vi "HandleObservationSync.vi"(8 "error in (no error)":errorcluster, 11 "S4ACS_GUI in":refnum<class "S4GUI.lvclass">) -> (0 "error out":errorcluster, 3 "S4ACS_GUI out":refnum<class "S4GUI.lvclass">)   [LabVIEW 2018, in "S4GUI.lvclass"]
uses:
  S4GUI.lvclass
  S4GUI.lvclass/S4GUI.ctl
  Instrument/Instrument.lvclass/Instrument.ctl
  Device/Optics/Optics.lvclass/Optics.ctl
  Server/Server.lvclass/Server.ctl
  Interface/Interface.lvclass/Interface.ctl
  Device/Optics/Opt_Selector/Opt_Selector.lvclass
  C:/Users/observer/Desktop/Sparc4GUI/SPARC4_GUI/Device/Optics/Optics.lvclass
  Acquisition/Acquisition.lvclass
  C:/Users/observer/Desktop/Sparc4GUI/SPARC4_GUI/Server/Server.lvclass
  SyncBox/Sync Box.lvclass
  Instrument/Instrument.lvclass
  Device/Optics/Opt_Continuous/Opt_Continuous.lvclass
  StateMachine/State Machine.lvclass
  Trigger/Trigger.lvclass
  Channel/Channel.lvclass
  Interface/Interface.lvclass
  Device/Optics/Optics.lvclass
  Server/Server.lvclass
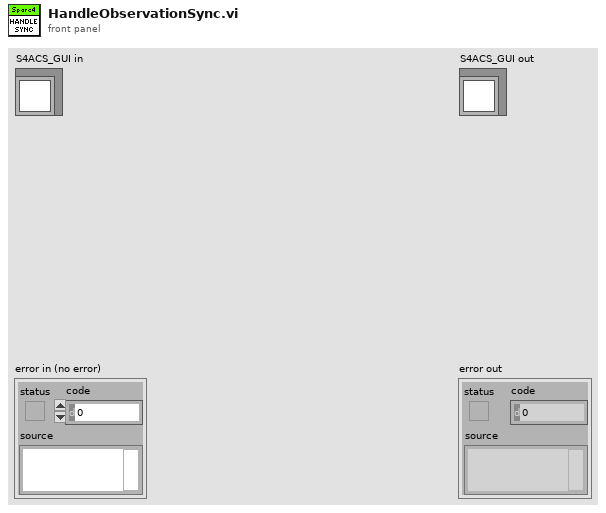
[diagram p1: front panel]
types:
  T1 = cluster{"ACQUISITION_MODE":u8, "TRIGGER_MODE":u8, "READ_MODE":u8, "PREAMP":u8, "READOUT_RATE":u8, "VERTICAL_SHIFT_SPEED":u8, "EM_MODE":u8, "EM_GAIN":u16, "SHUTTER_MODE":u8, "SHUTTER_TTL":u8, "SHUTTER_OPENING_TIME":u16, "SHUTTER_CLOSING_TIME":u16, "VBIN":u16, "HBIN":u16, "INITIAL_LINE":u16, "INITIAL_COLUMN":u16, "FINAL_LINE":u16, "FINAL_COLUMN":u16, "FRAME_TRANSFER":bool, "VERTICAL_CLOCK_VOLTAGE":u8, "AD_CHANNEL":u32}
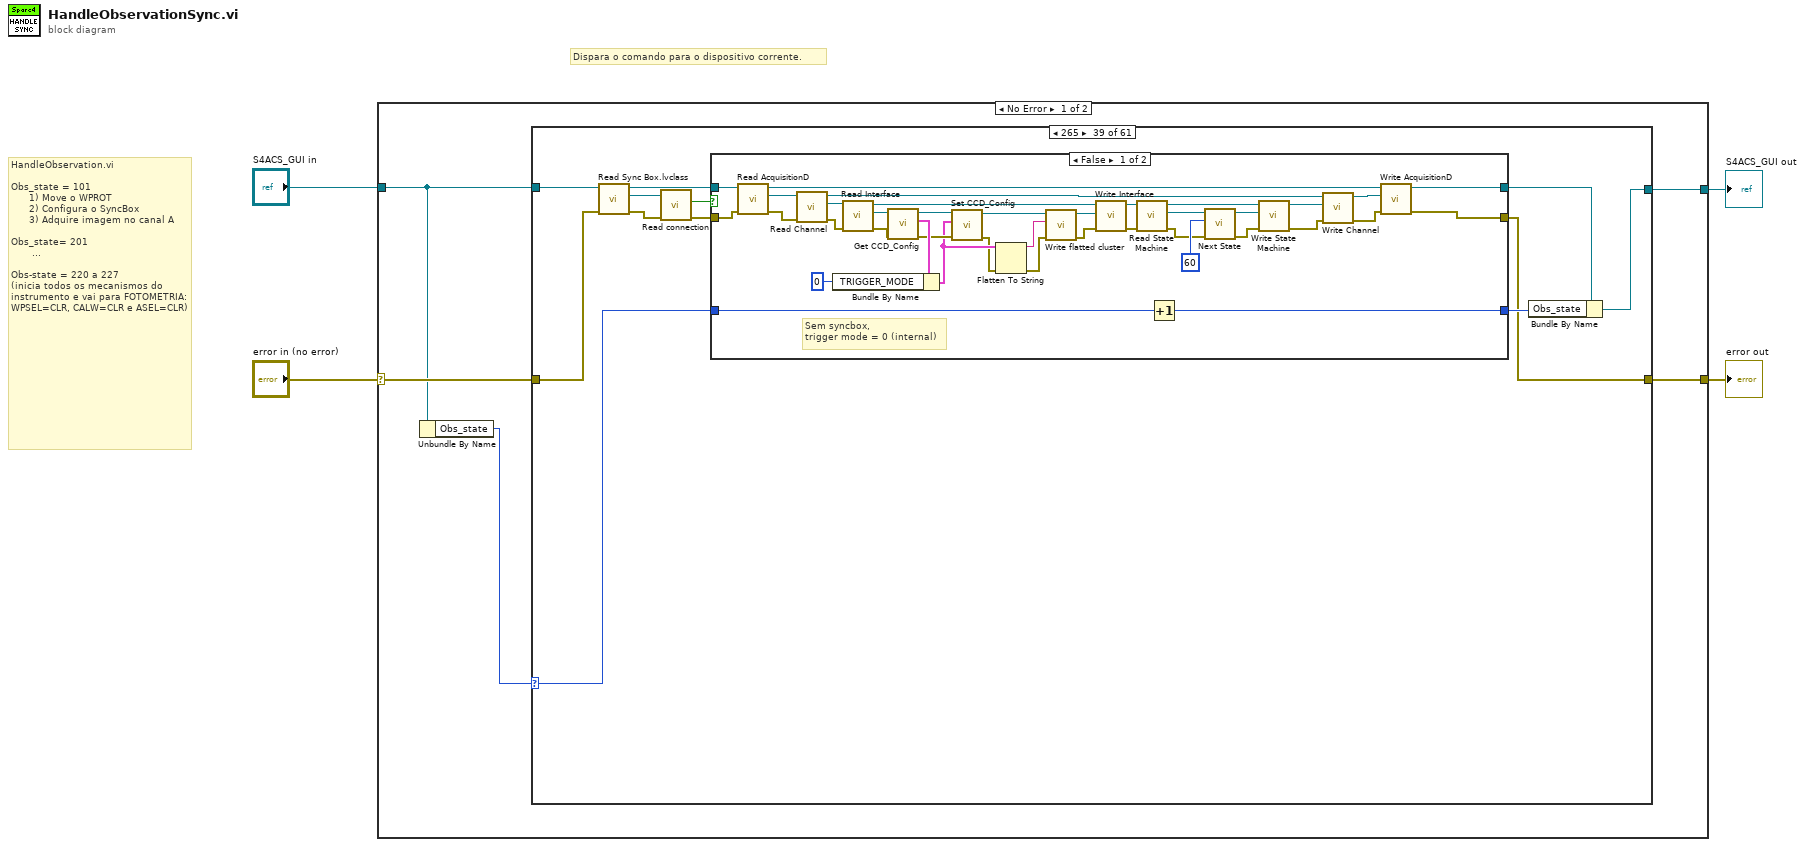
[diagram p0: block diagram]
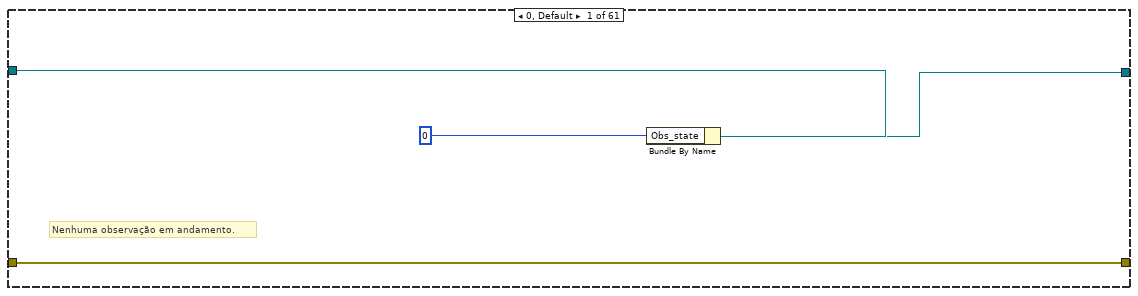
[diagram p2: hidden frame]
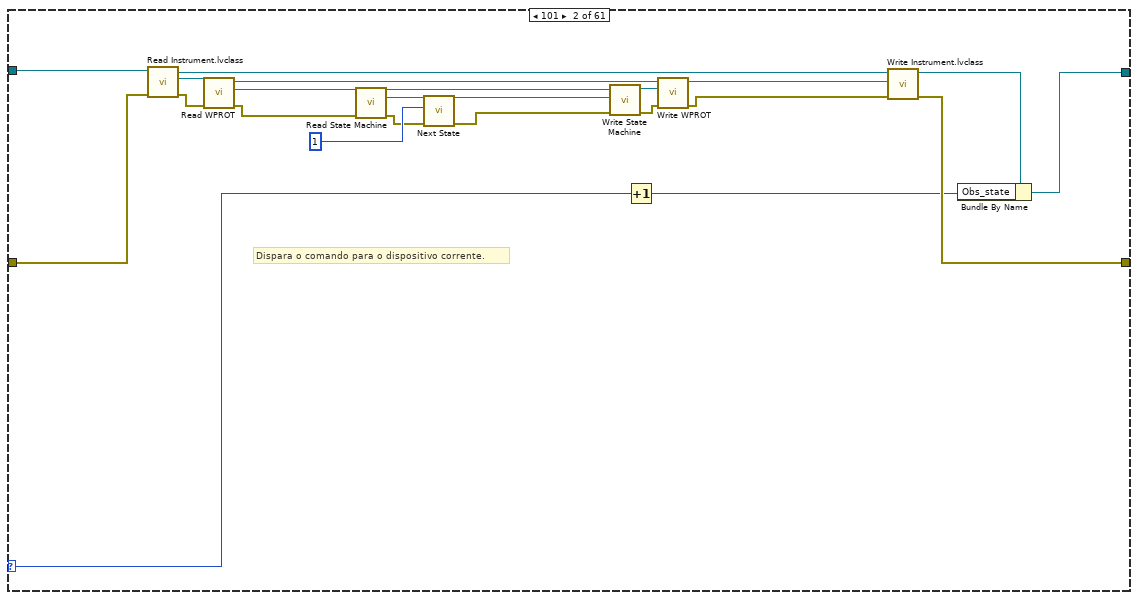
[diagram p3: hidden frame]
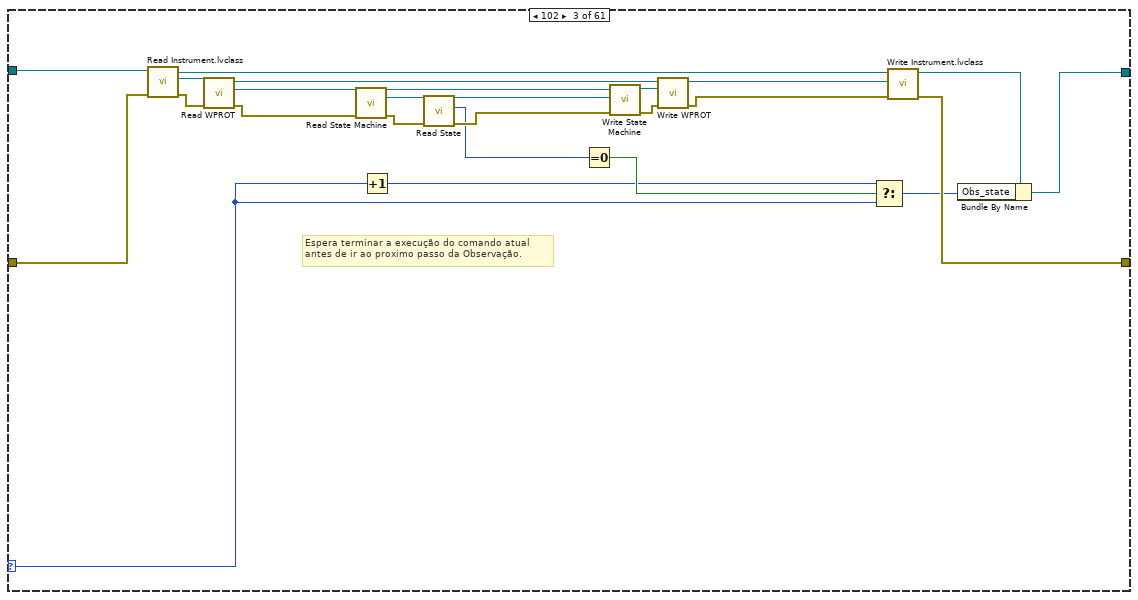
[diagram p4: hidden frame]
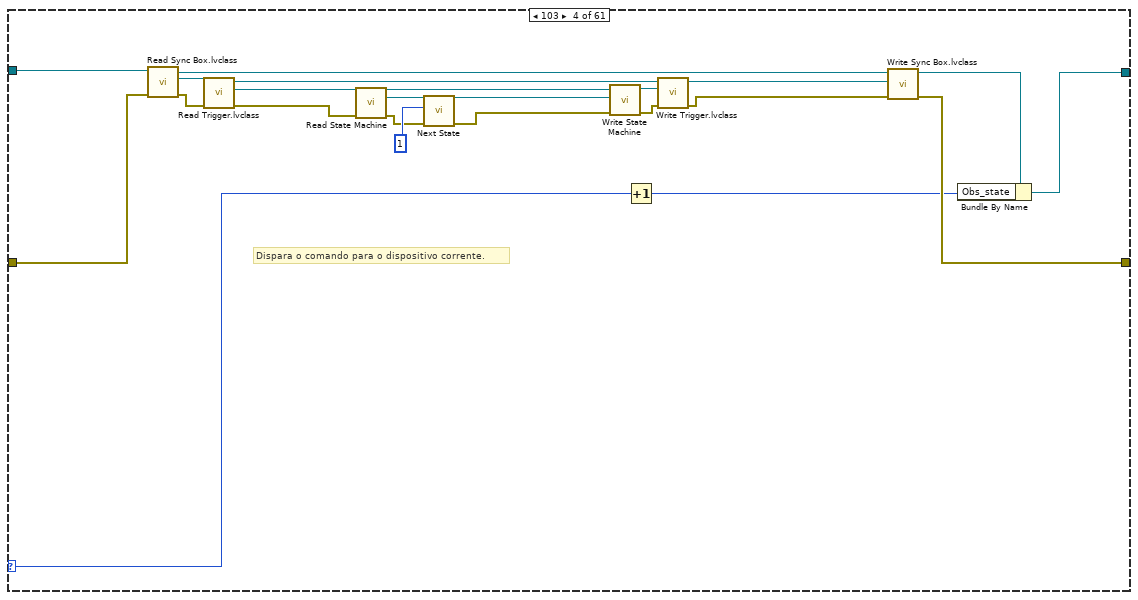
[diagram p5: hidden frame]
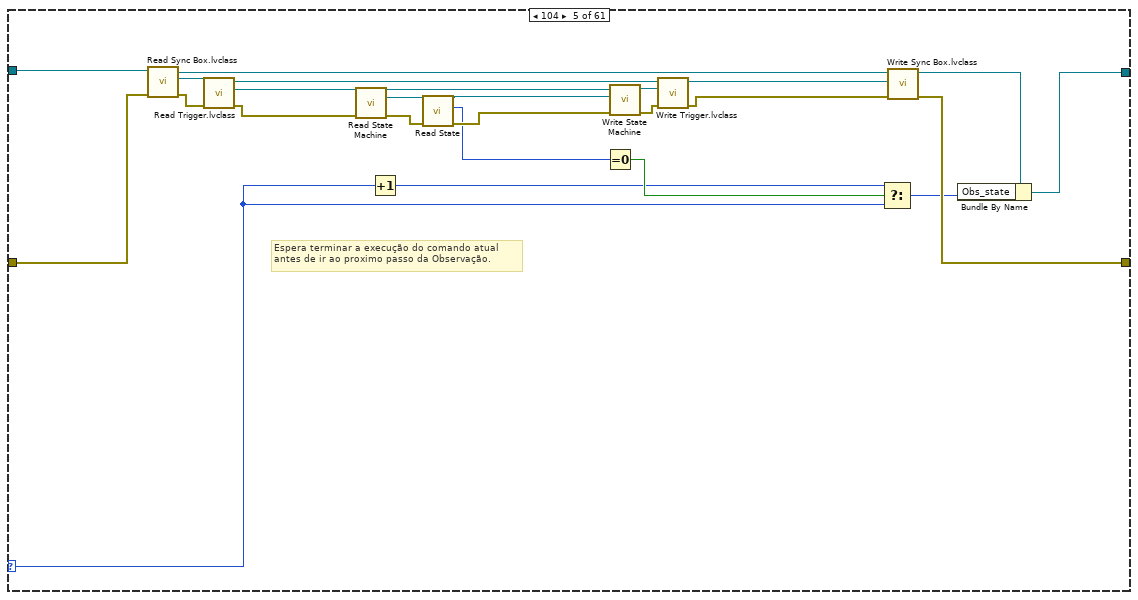
[diagram p6: hidden frame]
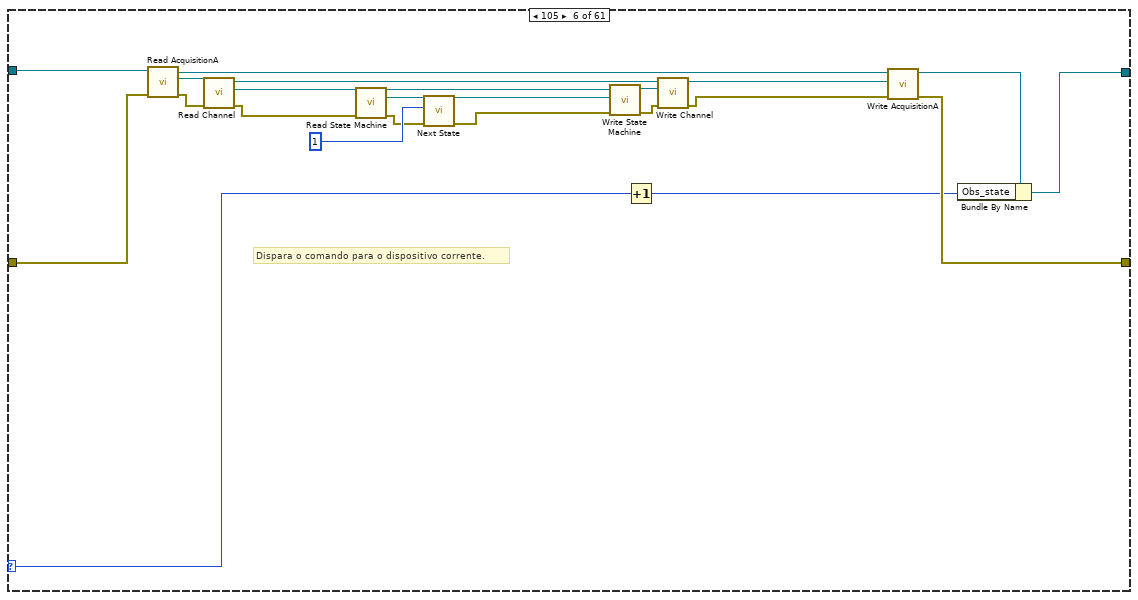
[diagram p7: hidden frame]
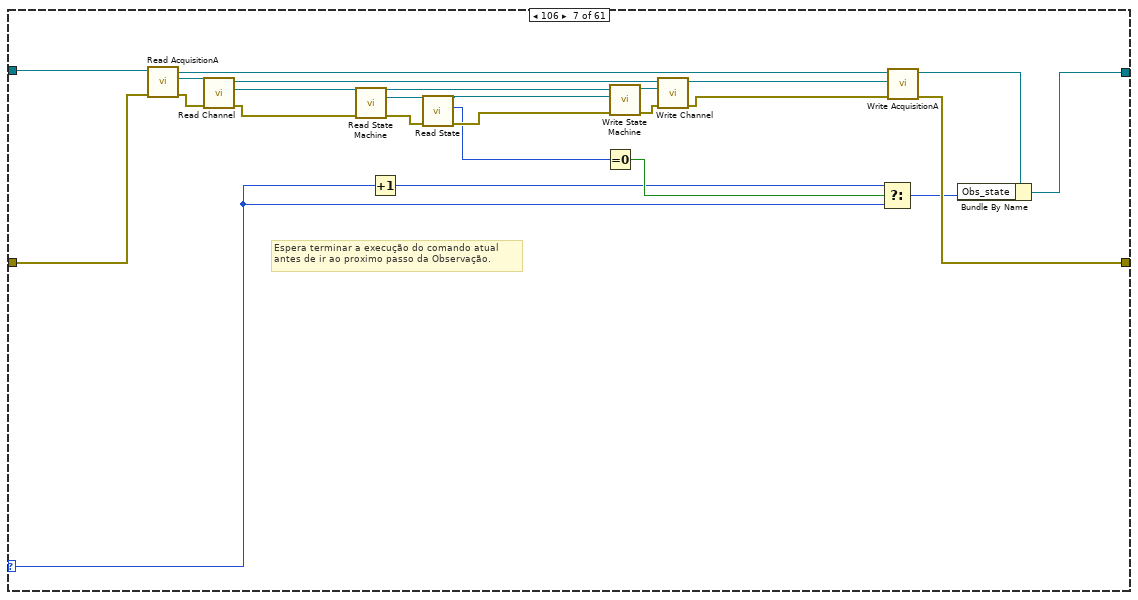
[diagram p8: hidden frame]
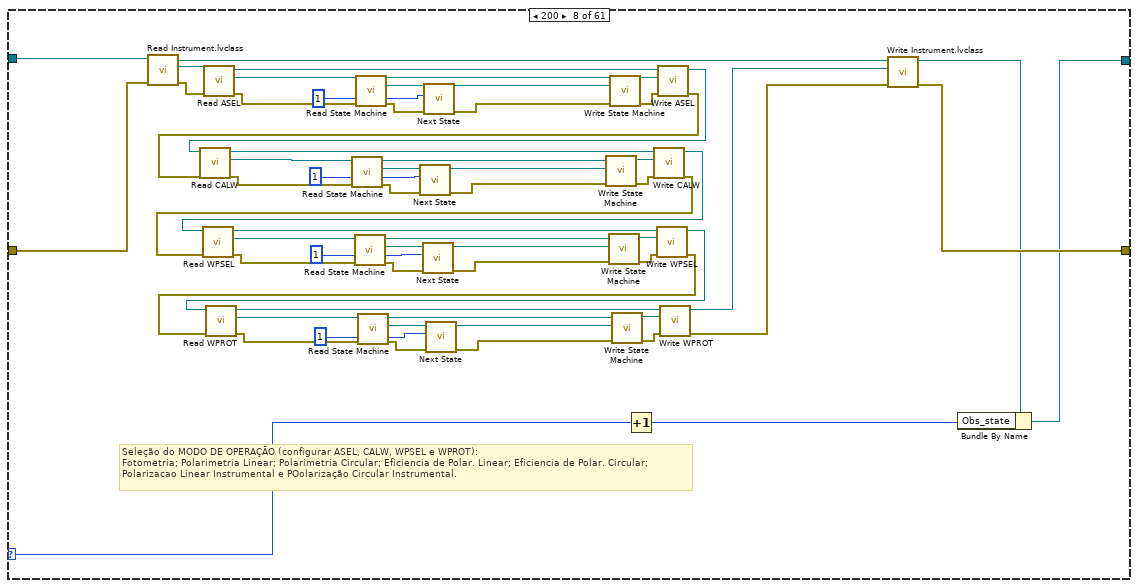
[diagram p9: hidden frame]
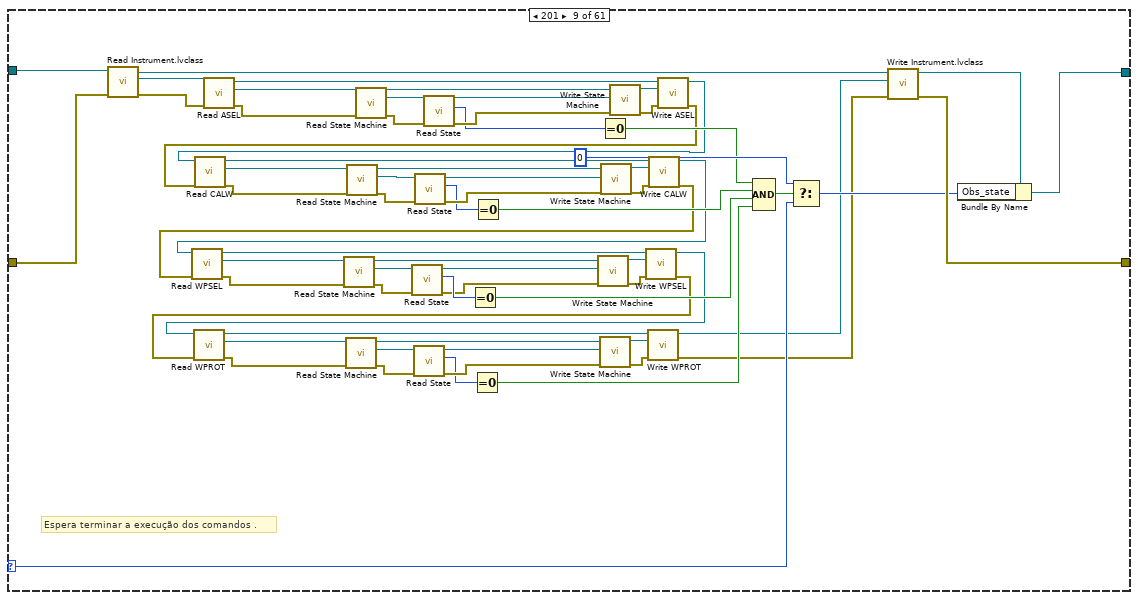
[diagram p10: hidden frame]
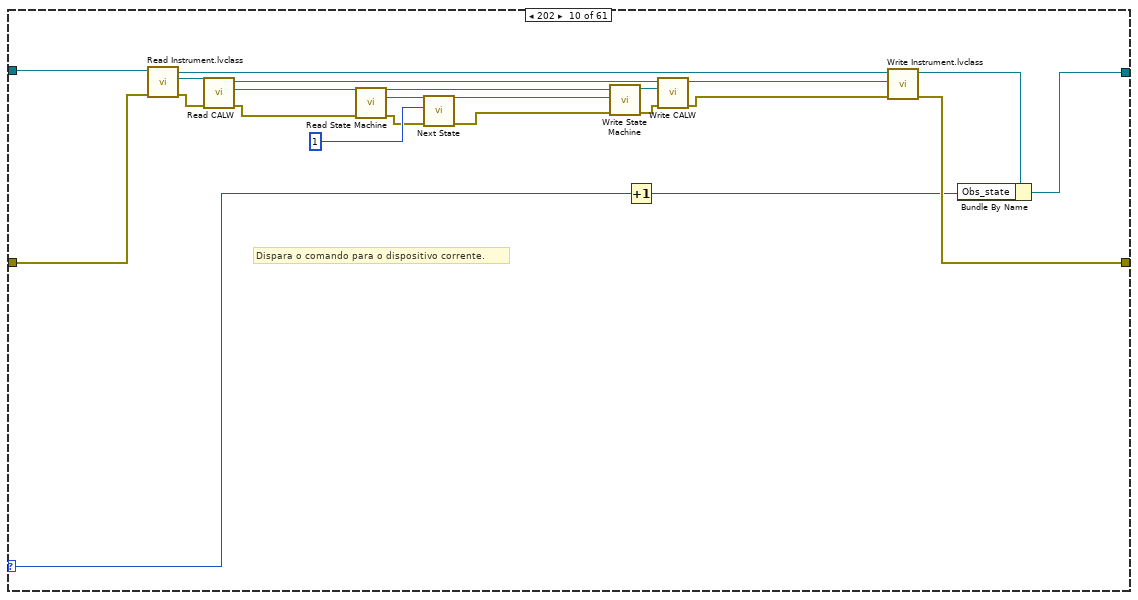
[diagram p11: hidden frame]
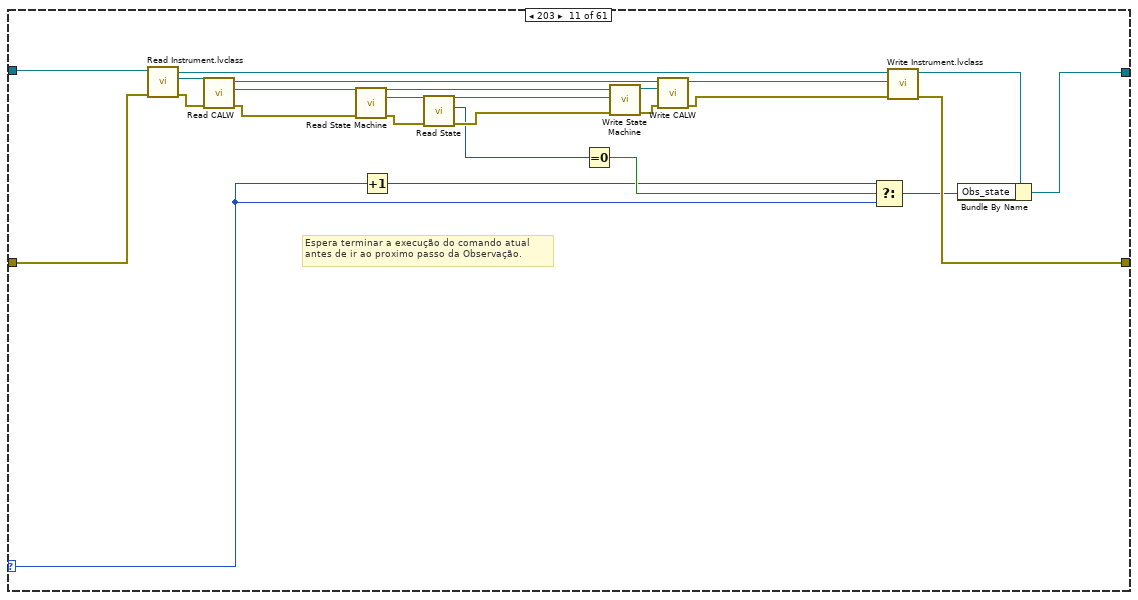
[diagram p12: hidden frame]
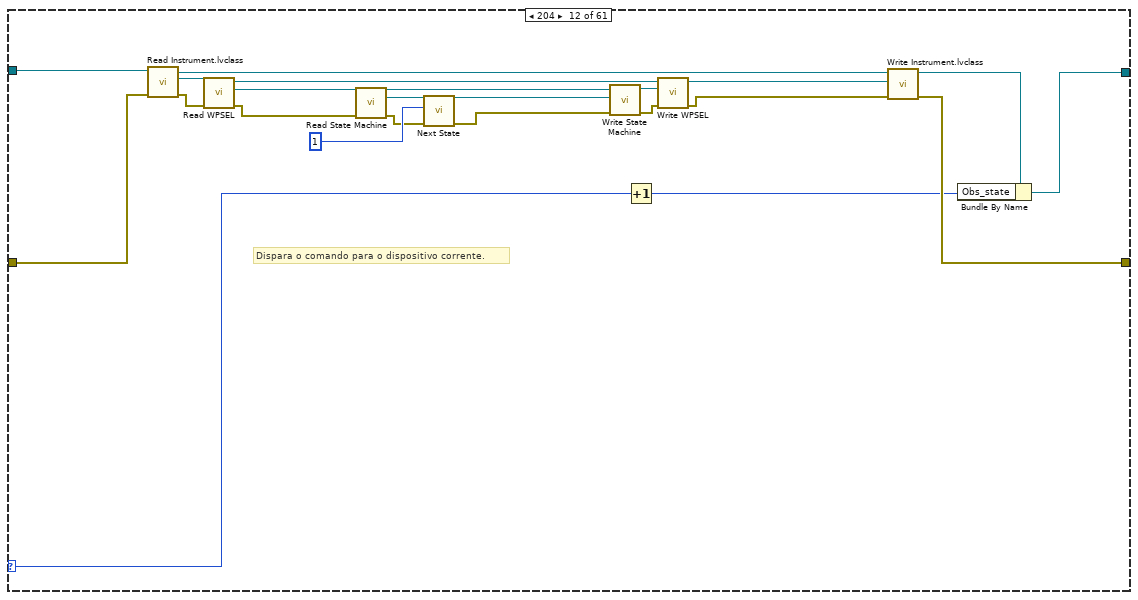
[diagram p13: hidden frame]
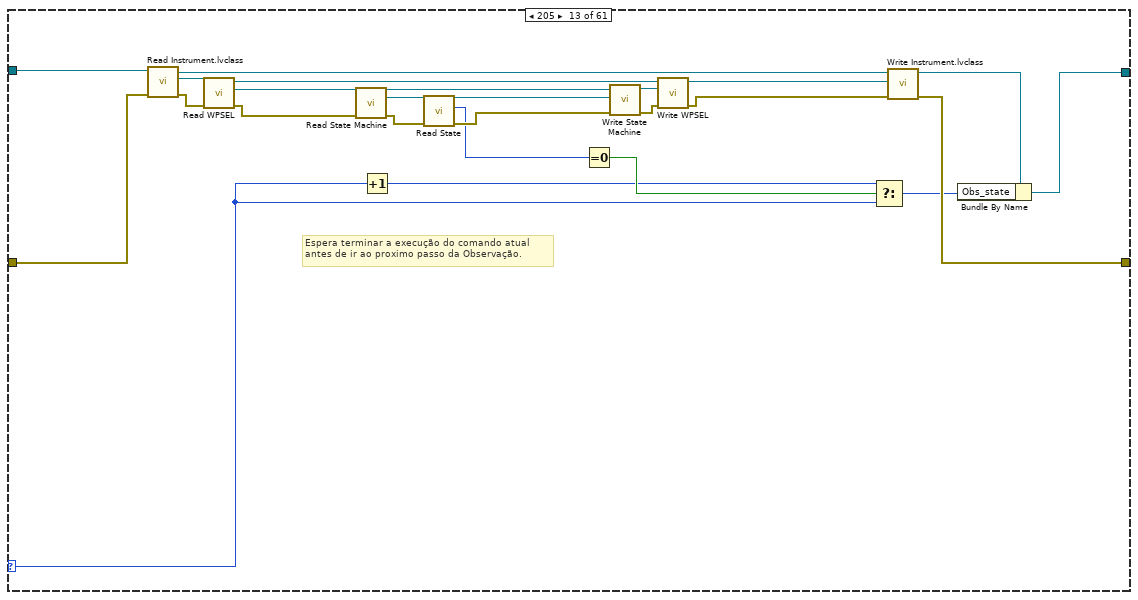
[diagram p14: hidden frame]
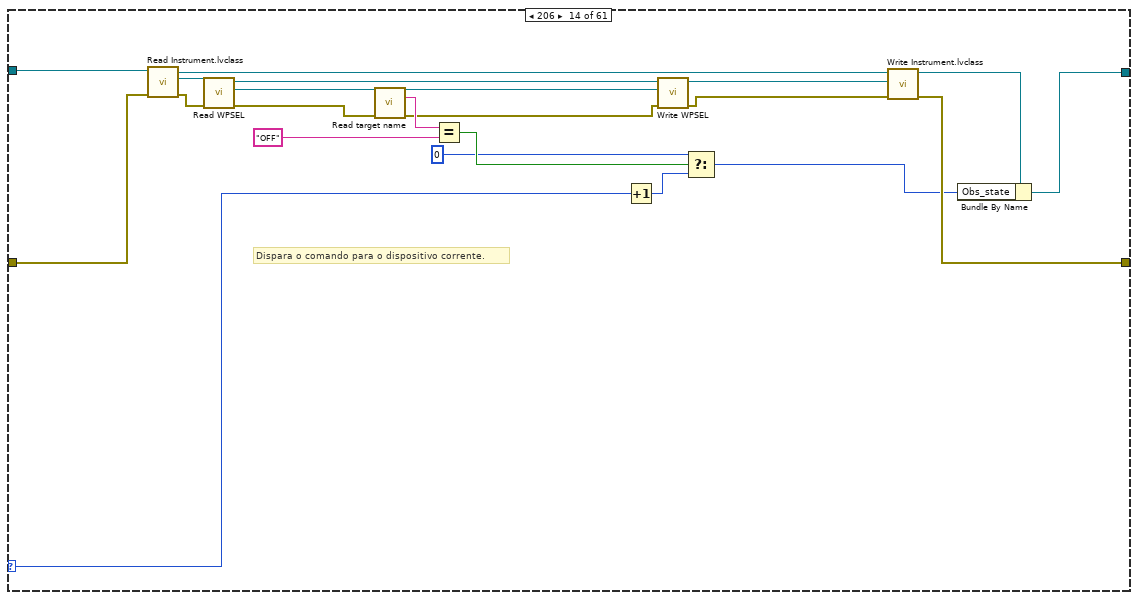
[diagram p15: hidden frame]
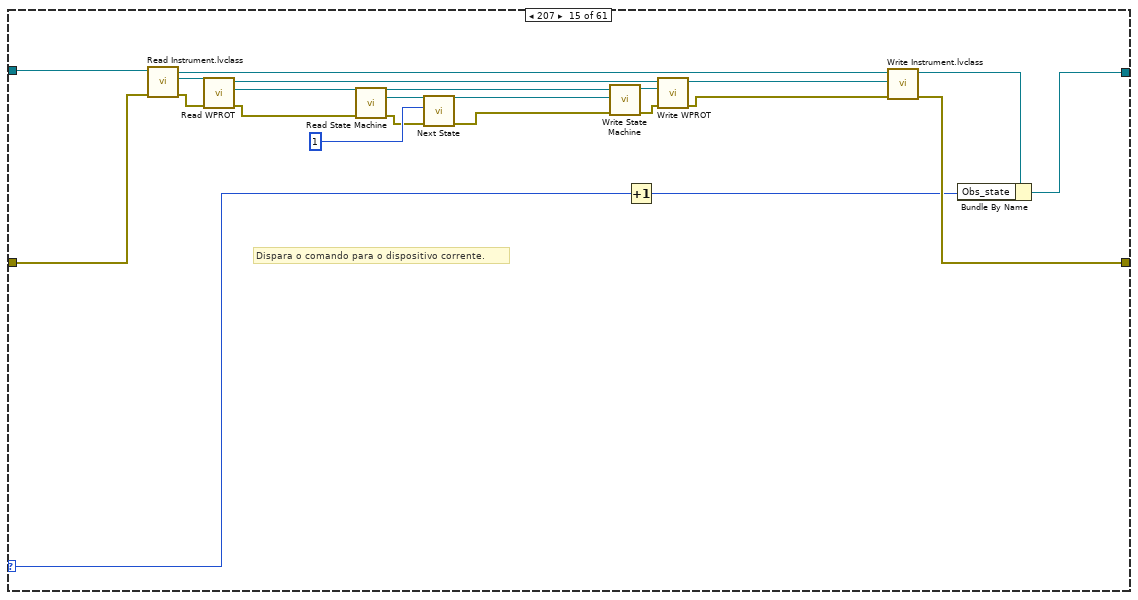
[diagram p16: hidden frame]
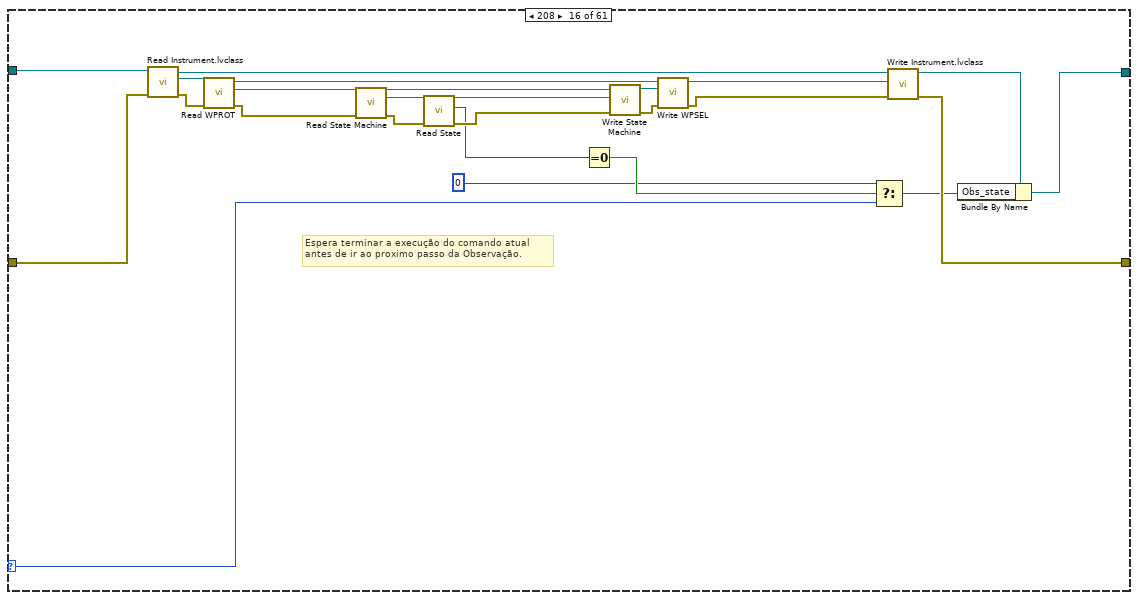
[diagram p17: hidden frame]
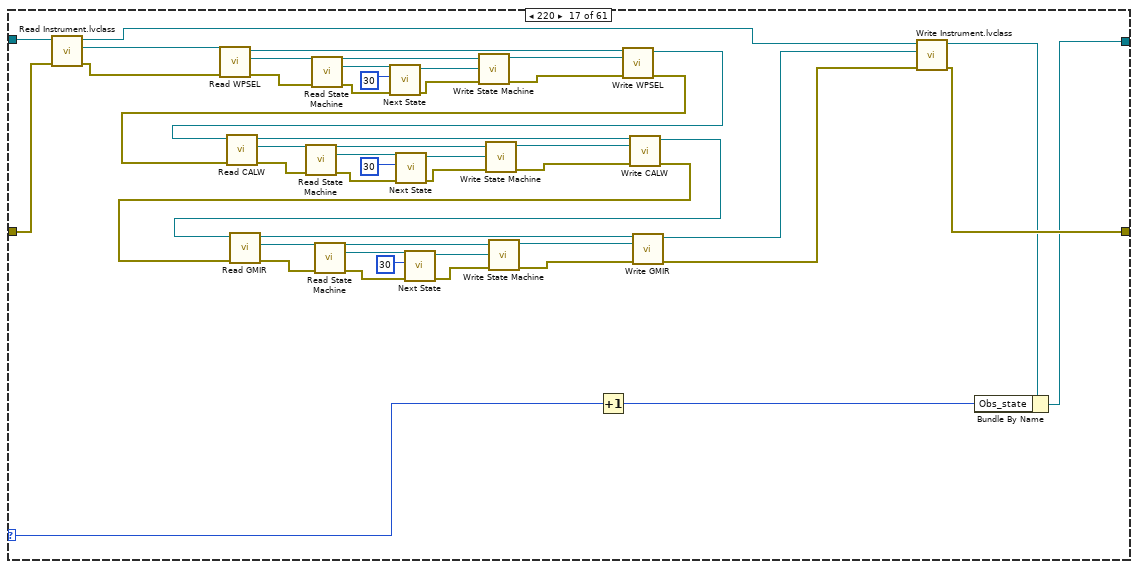
[diagram p18: hidden frame]
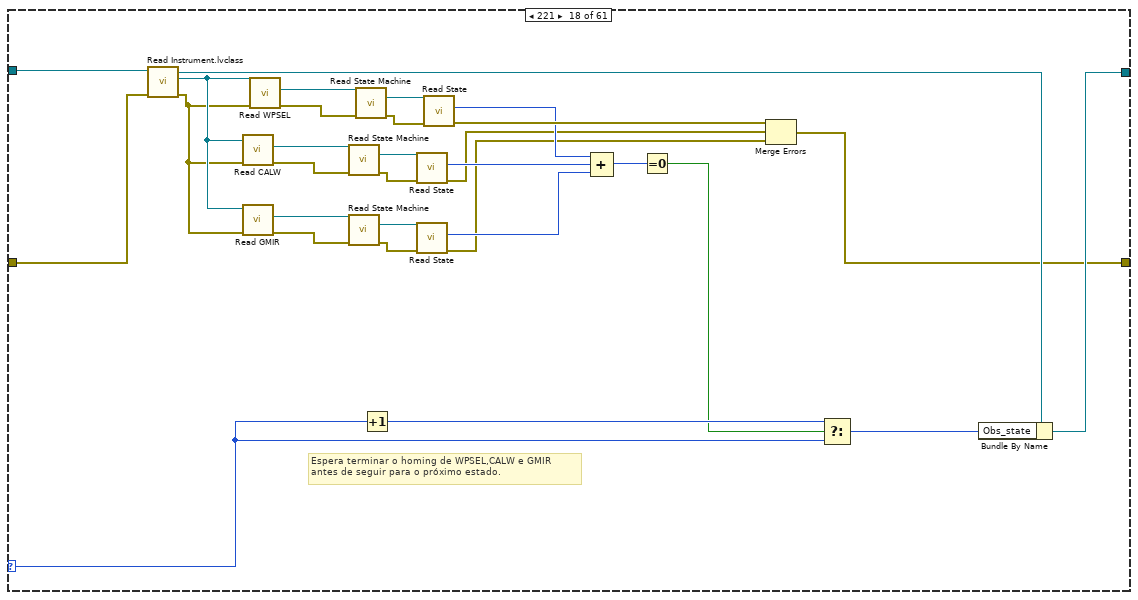
[diagram p19: hidden frame]
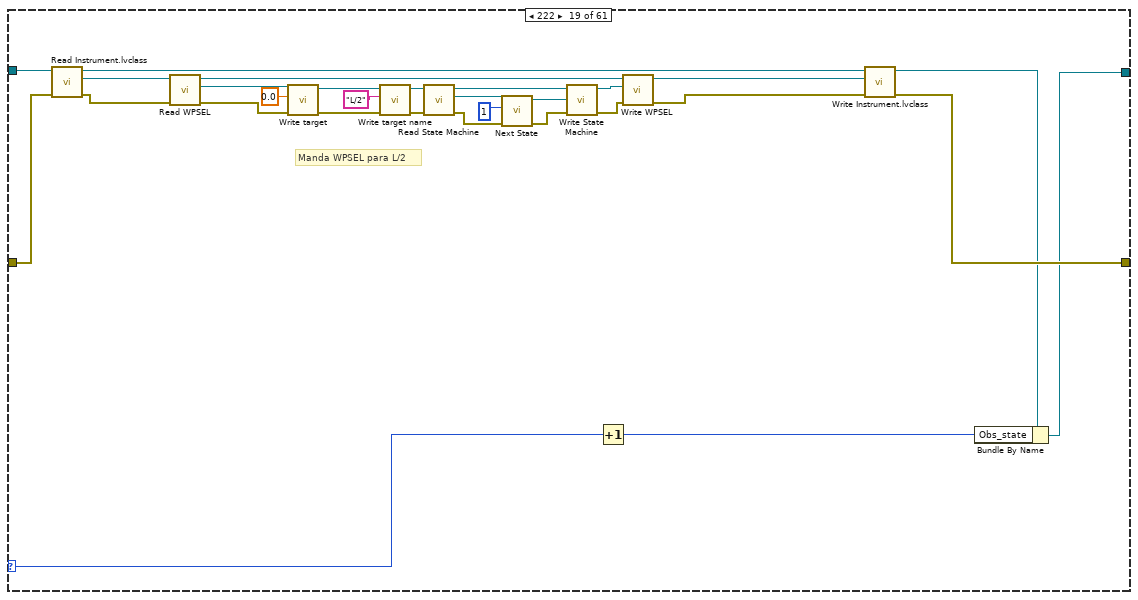
[diagram p20: hidden frame]
diagram:
  # "Dispara o comando para o dispositivo corrente."
  # "HandleObservation.vi\n\nObs_state = 101\n      1) Move o WPROT\n      2) Configura o SyncBox\n      3) Adquire imagem no canal A\n\nObs_state= 201\n       ...\n\nObs-state = 220 a 227 \n(inicia todos os mecanismos do instrumento e vai para FOTOMETRIA: WPSEL=CLR, CALW=CLR e ASEL=CLR)"
  n1 = case shown="No Error" "error in (no error)" {
    selector: "error in (no error)" -> [w8 w2519]
    tunnel: [w7 w2519] -> w3
    tunnel: [w9 w2518] -> w1
    tunnel: "S4ACS_GUI in" -> [w6 w2518]
    frame No Error {
      n2 = Unbundle By Name(w6) -> ("Obs_state"=w5:u32)
      n3 = case shown="265" w5 {
        selector: w5 -> [_ w16 w38 w64 w86 w112 w134 w202 w265 w290 w312 w338 w360 w395 w408 w430 w492 w524 w551 w569 w616 w648 w713 w745 w761 w796 w835 w879 w914 w950 w985 w1030 w1061 w1097 w1132 w1177 w1208 w1240 w1275 w1318 _ w1384 w1430 w1452 w1483 w1517 w1580 w1660 w1792 w1823 w1886 _ w1991 w2031 w2099 w2223 w2312 w2349 w2417 _ _]
        tunnel: w6 -> [w12 w30 w55 w78 w103 w126 w151 w216 w283 w304 w329 w352 w377 w399 w422 w447 w501 w532 w560 w577 w625 w656 w722 w753 w765 w814 w827 w897 w918 w967 w977 w1047 w1065 w1114 w1124 w1194 w1212 w1257 w1267 w1335 w1352 w1388 w1445 w1469 w1487 w1534 w1582 w1701 w1796 w1840 w1895 w1984 w2001 w2048 w2058 w2227 w2322 w2366 w2421 w2510 w2517]
        tunnel: [w10 w14 w42 w62 w94 w110 w142 w200 w270 w288 w316 w336 w364 w394 w406 w434 w496 w526 w555 w571 w620 w650 w717 w747 w759 w805 w833 w888 w912 w958 w983 w1038 w1059 w1105 w1130 w1185 w1206 w1248 w1273 w1326 w1350 w1382 w1434 w1460 w1481 w1525 w1578 w1699 w1790 w1831 w1893 w1980 w1997 w2039 w2097 w2225 w2318 w2357 w2419 w2506 w2517] -> w9
        tunnel: w8 -> [w13 w29 w54 w77 w102 w125 w150 w215 w282 w303 w328 w351 w376 w398 w421 w446 w500 w531 w559 w576 w624 w655 w721 w752 w764 w813 w828 w896 w917 w966 w978 w1046 w1064 w1113 w1125 w1193 w1211 w1256 w1268 w1334 w1351 w1387 w1444 w1468 w1486 w1533 w1581 w1700 w1795 w1839 w1894 w1983 w2000 w2047 w2057 w2226 w2321 w2365 w2420 w2509 w2516]
        tunnel: [w13 w28 w53 w76 w101 w124 w149 w214 w281 w302 w327 w350 w375 w397 w420 w445 w499 w505 w558 w563 w623 w629 w720 w727 w763 w812 w825 w895 w916 w965 w975 w1045 w1063 w1112 w1122 w1192 w1210 w1255 w1265 w1333 w1342 w1386 w1443 w1467 w1485 w1532 w1562 w1682 w1794 w1838 w1868 w1982 w1999 w2046 w2055 w2205 w2320 w2364 w2395 w2508 w2516] -> w7
        frame 0, Default {
          # "Nenhuma observação em andamento."
          n4 = Bundle By Name(cluster=w12, "Obs_state"=u32 0) -> (w10:refnum<class "S4GUI.lvclass">)
        }
        frame 101 {
          # "Dispara o comando para o dispositivo corrente."
          n5 = call "Read Instrument.lvclass.vi"("error in (no error)"=w29, "S4ACS_GUI in"=w30) -> ("error out"=w35:errorcluster, "Instrument.lvclass"=w36:refnum<class "Instrument.lvclass">, "S4ACS_GUI out"=w32:refnum<class "S4GUI.lvclass">)  [unwired: 7 in]
          n6 = call "Read WPROT.vi"("error in (no error)"=w35, "Instrument in"=w36) -> ("error out"=w22:errorcluster, "Opt_Selector.lvclass"=w21:refnum<class "Opt_Selector.lvclass">, "Instrument out"=w34:refnum<class "Instrument.lvclass">)  [unwired: 7 in]
          n7 = call-dynamic "Read State Machine.vi"("error in (no error)"=w22, "Device in"=w21) -> ("error out"=w25:errorcluster, "State Machine.lvclass"=w27:refnum<class "State Machine.lvclass">, "Device out"=w19:refnum<class "Opt_Selector.lvclass">)  [unwired: 7 in]
          n8 = call "Next State.vi"("error in (no error)"=w25, "New_State"=1, "State Machine in"=w27) -> ("error out"=w24:errorcluster, "State Machine out"=w23:refnum<class "State Machine.lvclass">)  [unwired: 7 in]
          n9 = call-dynamic "Write State Machine.vi"("error in (no error)"=w24, "State Machine.lvclass"=w23, "Device in"=w19) -> ("error out"=w18:errorcluster, "Device out"=w20:refnum<class "Opt_Selector.lvclass">)  [unwired: 7 in]
          n10 = Increment(x=w16) -> (x+1=w15:u32)
          n11 = call "Write WPROT.vi"("error in (no error)"=w18, "Opt_Selector.lvclass"=w20, "Instrument in"=w34) -> ("error out"=w31:errorcluster, "Instrument out"=w33:refnum<class "Instrument.lvclass">)  [unwired: 7 in]
          n12 = call "Write Instrument.lvclass.vi"("error in (no error)"=w31, "Instrument.lvclass"=w33, "S4ACS_GUI in"=w32) -> ("error out"=w28:errorcluster, "S4ACS_GUI out"=w17:refnum<class "S4GUI.lvclass">)  [unwired: 7 in]
          n13 = Bundle By Name(cluster=w17, "Obs_state"=w15) -> (w14:refnum<class "S4GUI.lvclass">)
        }
        frame 102 {
          # "Espera terminar a execução do comando atual \nantes de ir ao proximo passo da Observação."
          n14 = call "Read Instrument.lvclass.vi"("error in (no error)"=w54, "S4ACS_GUI in"=w55) -> ("error out"=w60:errorcluster, "Instrument.lvclass"=w61:refnum<class "Instrument.lvclass">, "S4ACS_GUI out"=w57:refnum<class "S4GUI.lvclass">)  [unwired: 7 in]
          n15 = call "Read WPROT.vi"("error in (no error)"=w60, "Instrument in"=w61) -> ("error out"=w48:errorcluster, "Opt_Selector.lvclass"=w47:refnum<class "Opt_Selector.lvclass">, "Instrument out"=w59:refnum<class "Instrument.lvclass">)  [unwired: 7 in]
          n16 = call-dynamic "Read State Machine.vi"("error in (no error)"=w48, "Device in"=w47) -> ("error out"=w51:errorcluster, "State Machine.lvclass"=w52:refnum<class "State Machine.lvclass">, "Device out"=w45:refnum<class "Opt_Selector.lvclass">)  [unwired: 7 in]
          n17 = Increment(x=w38) -> (x+1=w37:u32)
          n18 = call-dynamic "Read State.vi"("error in (no error)"=w51, "State Machine in"=w52) -> ("error out"=w50:errorcluster, "State"=w40:i32, "State Machine out"=w49:refnum<class "State Machine.lvclass">)  [unwired: 7 in]
          n19 = Equal To 0?(x=w40) -> (x = 0?=w41:bool)
          n20 = call-dynamic "Write State Machine.vi"("error in (no error)"=w50, "State Machine.lvclass"=w49, "Device in"=w45) -> ("error out"=w44:errorcluster, "Device out"=w46:refnum<class "Opt_Selector.lvclass">)  [unwired: 7 in]
          n21 = call "Write WPROT.vi"("error in (no error)"=w44, "Opt_Selector.lvclass"=w46, "Instrument in"=w59) -> ("error out"=w56:errorcluster, "Instrument out"=w58:refnum<class "Instrument.lvclass">)  [unwired: 7 in]
          n22 = Select(t=w37, s=w41, f=w38) -> (s? t:f=w39:u32)
          n23 = call "Write Instrument.lvclass.vi"("error in (no error)"=w56, "Instrument.lvclass"=w58, "S4ACS_GUI in"=w57) -> ("error out"=w53:errorcluster, "S4ACS_GUI out"=w43:refnum<class "S4GUI.lvclass">)  [unwired: 7 in]
          n24 = Bundle By Name(cluster=w43, "Obs_state"=w39) -> (w42:refnum<class "S4GUI.lvclass">)
        }
        frame 103 {
          # "Dispara o comando para o dispositivo corrente."
          n25 = call-dynamic "Read Sync Box.lvclass.vi"("error in (no error)"=w77, "SPARC4_AC in"=w78) -> ("error out"=w83:errorcluster, "Sync Box.lvclass"=w84:refnum<class "Sync Box.lvclass">, "SPARC4_AC out"=w80:refnum<class "S4GUI.lvclass">)  [unwired: 7 in]
          n26 = call-dynamic "Read Trigger.lvclass.vi"("error in (no error)"=w83, "Sync Box in"=w84) -> ("error out"=w70:errorcluster, "Trigger.lvclass"=w69:refnum<class "Trigger.lvclass">, "Sync Box out"=w82:refnum<class "Sync Box.lvclass">)  [unwired: 7 in]
          n27 = call-dynamic "Read State Machine.vi"("error in (no error)"=w70, "Device in"=w69) -> ("error out"=w73:errorcluster, "State Machine.lvclass"=w75:refnum<class "State Machine.lvclass">, "Device out"=w67:refnum<class "Trigger.lvclass">)  [unwired: 7 in]
          n28 = call "Next State.vi"("error in (no error)"=w73, "New_State"=1, "State Machine in"=w75) -> ("error out"=w72:errorcluster, "State Machine out"=w71:refnum<class "State Machine.lvclass">)  [unwired: 7 in]
          n29 = call-dynamic "Write State Machine.vi"("error in (no error)"=w72, "State Machine.lvclass"=w71, "Device in"=w67) -> ("error out"=w66:errorcluster, "Device out"=w68:refnum<class "Trigger.lvclass">)  [unwired: 7 in]
          n30 = Increment(x=w64) -> (x+1=w63:u32)
          n31 = call-dynamic "Write Trigger.lvclass.vi"("error in (no error)"=w66, "Trigger.lvclass"=w68, "Sync Box in"=w82) -> ("error out"=w79:errorcluster, "Sync Box out"=w81:refnum<class "Sync Box.lvclass">)  [unwired: 7 in]
          n32 = call-dynamic "Write Sync Box.lvclass.vi"("error in (no error)"=w79, "Sync Box.lvclass"=w81, "SPARC4_AC in"=w80) -> ("error out"=w76:errorcluster, "SPARC4_AC out"=w65:refnum<class "S4GUI.lvclass">)  [unwired: 7 in]
          n33 = Bundle By Name(cluster=w65, "Obs_state"=w63) -> (w62:refnum<class "S4GUI.lvclass">)
        }
        frame 104 {
          # "Espera terminar a execução do comando atual \nantes de ir ao proximo passo da Observação."
          n34 = call-dynamic "Read Sync Box.lvclass.vi"("error in (no error)"=w102, "SPARC4_AC in"=w103) -> ("error out"=w108:errorcluster, "Sync Box.lvclass"=w109:refnum<class "Sync Box.lvclass">, "SPARC4_AC out"=w105:refnum<class "S4GUI.lvclass">)  [unwired: 7 in]
          n35 = call-dynamic "Read Trigger.lvclass.vi"("error in (no error)"=w108, "Sync Box in"=w109) -> ("error out"=w100:errorcluster, "Trigger.lvclass"=w99:refnum<class "Trigger.lvclass">, "Sync Box out"=w107:refnum<class "Sync Box.lvclass">)  [unwired: 7 in]
          n36 = call-dynamic "Read State Machine.vi"("error in (no error)"=w100, "Device in"=w99) -> ("error out"=w91:errorcluster, "State Machine.lvclass"=w93:refnum<class "State Machine.lvclass">, "Device out"=w97:refnum<class "Trigger.lvclass">)  [unwired: 7 in]
          n37 = Increment(x=w86) -> (x+1=w88:u32)
          n38 = call-dynamic "Read State.vi"("error in (no error)"=w91, "State Machine in"=w93) -> ("error out"=w90:errorcluster, "State"=w85:i32, "State Machine out"=w92:refnum<class "State Machine.lvclass">)  [unwired: 7 in]
          n39 = Equal To 0?(x=w85) -> (x = 0?=w89:bool)
          n40 = call-dynamic "Write State Machine.vi"("error in (no error)"=w90, "State Machine.lvclass"=w92, "Device in"=w97) -> ("error out"=w96:errorcluster, "Device out"=w98:refnum<class "Trigger.lvclass">)  [unwired: 7 in]
          n41 = call-dynamic "Write Trigger.lvclass.vi"("error in (no error)"=w96, "Trigger.lvclass"=w98, "Sync Box in"=w107) -> ("error out"=w104:errorcluster, "Sync Box out"=w106:refnum<class "Sync Box.lvclass">)  [unwired: 7 in]
          n42 = Select(t=w88, s=w89, f=w86) -> (s? t:f=w87:u32)
          n43 = call-dynamic "Write Sync Box.lvclass.vi"("error in (no error)"=w104, "Sync Box.lvclass"=w106, "SPARC4_AC in"=w105) -> ("error out"=w101:errorcluster, "SPARC4_AC out"=w95:refnum<class "S4GUI.lvclass">)  [unwired: 7 in]
          n44 = Bundle By Name(cluster=w95, "Obs_state"=w87) -> (w94:refnum<class "S4GUI.lvclass">)
        }
        frame 105 {
          # "Dispara o comando para o dispositivo corrente."
          n45 = call-dynamic "Read AcquisitionA.vi"("error in (no error)"=w125, "S4ACS_GUI in"=w126) -> ("error out"=w131:errorcluster, "Acquisition.lvclass"=w132:refnum<class "Acquisition.lvclass">, "S4ACS_GUI out"=w128:refnum<class "S4GUI.lvclass">)  [unwired: 7 in]
          n46 = call-dynamic "Read Channel.vi"("error in (no error)"=w131, "Acquisition in"=w132) -> ("error out"=w118:errorcluster, "Channel.lvclass"=w117:refnum<class "Channel.lvclass">, "Acquisition out"=w130:refnum<class "Acquisition.lvclass">)  [unwired: 7 in]
          n47 = call-dynamic "Read State Machine.vi"("error in (no error)"=w118, "Device in"=w117) -> ("error out"=w121:errorcluster, "State Machine.lvclass"=w123:refnum<class "State Machine.lvclass">, "Device out"=w115:refnum<class "Channel.lvclass">)  [unwired: 7 in]
          n48 = call "Next State.vi"("error in (no error)"=w121, "New_State"=1, "State Machine in"=w123) -> ("error out"=w120:errorcluster, "State Machine out"=w119:refnum<class "State Machine.lvclass">)  [unwired: 7 in]
          n49 = call-dynamic "Write State Machine.vi"("error in (no error)"=w120, "State Machine.lvclass"=w119, "Device in"=w115) -> ("error out"=w114:errorcluster, "Device out"=w116:refnum<class "Channel.lvclass">)  [unwired: 7 in]
          n50 = Increment(x=w112) -> (x+1=w111:u32)
          n51 = call-dynamic "Write Channel.vi"("error in (no error)"=w114, "Channel.lvclass"=w116, "Acquisition in"=w130) -> ("error out"=w127:errorcluster, "Acquisition out"=w129:refnum<class "Acquisition.lvclass">)  [unwired: 7 in]
          n52 = call-dynamic "Write AcquisitionA.vi"("error in (no error)"=w127, "Acquisition.lvclass"=w129, "S4ACS_GUI in"=w128) -> ("error out"=w124:errorcluster, "S4ACS_GUI out"=w113:refnum<class "S4GUI.lvclass">)  [unwired: 7 in]
          n53 = Bundle By Name(cluster=w113, "Obs_state"=w111) -> (w110:refnum<class "S4GUI.lvclass">)
        }
        frame 106 {
          # "Espera terminar a execução do comando atual \nantes de ir ao proximo passo da Observação."
          n54 = call-dynamic "Read AcquisitionA.vi"("error in (no error)"=w150, "S4ACS_GUI in"=w151) -> ("error out"=w156:errorcluster, "Acquisition.lvclass"=w157:refnum<class "Acquisition.lvclass">, "S4ACS_GUI out"=w153:refnum<class "S4GUI.lvclass">)  [unwired: 7 in]
          n55 = call-dynamic "Read Channel.vi"("error in (no error)"=w156, "Acquisition in"=w157) -> ("error out"=w148:errorcluster, "Channel.lvclass"=w147:refnum<class "Channel.lvclass">, "Acquisition out"=w155:refnum<class "Acquisition.lvclass">)  [unwired: 7 in]
          n56 = call-dynamic "Read State Machine.vi"("error in (no error)"=w148, "Device in"=w147) -> ("error out"=w139:errorcluster, "State Machine.lvclass"=w141:refnum<class "State Machine.lvclass">, "Device out"=w145:refnum<class "Channel.lvclass">)  [unwired: 7 in]
          n57 = Increment(x=w134) -> (x+1=w136:u32)
          n58 = call-dynamic "Read State.vi"("error in (no error)"=w139, "State Machine in"=w141) -> ("error out"=w138:errorcluster, "State"=w133:i32, "State Machine out"=w140:refnum<class "State Machine.lvclass">)  [unwired: 7 in]
          n59 = Equal To 0?(x=w133) -> (x = 0?=w137:bool)
          n60 = call-dynamic "Write State Machine.vi"("error in (no error)"=w138, "State Machine.lvclass"=w140, "Device in"=w145) -> ("error out"=w144:errorcluster, "Device out"=w146:refnum<class "Channel.lvclass">)  [unwired: 7 in]
          n61 = call-dynamic "Write Channel.vi"("error in (no error)"=w144, "Channel.lvclass"=w146, "Acquisition in"=w155) -> ("error out"=w152:errorcluster, "Acquisition out"=w154:refnum<class "Acquisition.lvclass">)  [unwired: 7 in]
          n62 = Select(t=w136, s=w137, f=w134) -> (s? t:f=w135:u32)
          n63 = call-dynamic "Write AcquisitionA.vi"("error in (no error)"=w152, "Acquisition.lvclass"=w154, "S4ACS_GUI in"=w153) -> ("error out"=w149:errorcluster, "S4ACS_GUI out"=w143:refnum<class "S4GUI.lvclass">)  [unwired: 7 in]
          n64 = Bundle By Name(cluster=w143, "Obs_state"=w135) -> (w142:refnum<class "S4GUI.lvclass">)
        }
        frame 200 {
          # "Seleção do MODO DE OPERAÇÃO (configurar ASEL, CALW, WPSEL e WPROT): \nFotometria; Polarimetria Linear; Polarimetria Circular; Eficiencia de Polar. Linear; Eficiencia de Polar. Circular;\nPolarizacao Linear Instrumental e POolarização Circular Instrumental."
          n65 = call "Read Instrument.lvclass.vi"("error in (no error)"=w215, "S4ACS_GUI in"=w216) -> ("error out"=w219:errorcluster, "Instrument.lvclass"=w179:refnum<class "Instrument.lvclass">, "S4ACS_GUI out"=w217:refnum<class "S4GUI.lvclass">)  [unwired: 7 in]
          n66 = call "Read ASEL.vi"("error in (no error)"=w219, "Instrument in"=w179) -> ("error out"=w208:errorcluster, "Opt_Selector.lvclass"=w207:refnum<class "Opt_Selector.lvclass">, "Instrument out"=w218:refnum<class "Instrument.lvclass">)  [unwired: 7 in]
          n67 = call-dynamic "Read State Machine.vi"("error in (no error)"=w208, "Device in"=w207) -> ("error out"=w211:errorcluster, "State Machine.lvclass"=w213:refnum<class "State Machine.lvclass">, "Device out"=w205:refnum<class "Opt_Selector.lvclass">)  [unwired: 7 in]
          n68 = call "Next State.vi"("error in (no error)"=w211, "New_State"=1, "State Machine in"=w213) -> ("error out"=w210:errorcluster, "State Machine out"=w209:refnum<class "State Machine.lvclass">)  [unwired: 7 in]
          n69 = call-dynamic "Write State Machine.vi"("error in (no error)"=w210, "State Machine.lvclass"=w209, "Device in"=w205) -> ("error out"=w204:errorcluster, "Device out"=w206:refnum<class "Opt_Selector.lvclass">)  [unwired: 7 in]
          n70 = Increment(x=w202) -> (x+1=w201:u32)
          n71 = call "Write ASEL.vi"("error in (no error)"=w204, "Opt_Selector.lvclass"=w206, "Instrument in"=w218) -> ("error out"=w160:errorcluster, "Instrument out"=w178:refnum<class "Instrument.lvclass">)  [unwired: 7 in]
          n72 = call "Read CALW.vi"("error in (no error)"=w160, "Instrument in"=w178) -> ("error out"=w195:errorcluster, "Opt_Selector.lvclass"=w196:refnum<class "Opt_Selector.lvclass">, "Instrument out"=w177:refnum<class "Instrument.lvclass">)  [unwired: 7 in]
          n73 = call-dynamic "Read State Machine.vi"("error in (no error)"=w195, "Device in"=w196) -> ("error out"=w192:errorcluster, "State Machine.lvclass"=w190:refnum<class "State Machine.lvclass">, "Device out"=w198:refnum<class "Opt_Selector.lvclass">)  [unwired: 7 in]
          n74 = call "Next State.vi"("error in (no error)"=w192, "New_State"=1, "State Machine in"=w190) -> ("error out"=w193:errorcluster, "State Machine out"=w194:refnum<class "State Machine.lvclass">)  [unwired: 7 in]
          n75 = call-dynamic "Write State Machine.vi"("error in (no error)"=w193, "State Machine.lvclass"=w194, "Device in"=w198) -> ("error out"=w199:errorcluster, "Device out"=w197:refnum<class "Opt_Selector.lvclass">)  [unwired: 7 in]
          n76 = call "Write CALW.vi"("error in (no error)"=w199, "Opt_Selector.lvclass"=w197, "Instrument in"=w177) -> ("error out"=w159:errorcluster, "Instrument out"=w176:refnum<class "Instrument.lvclass">)  [unwired: 7 in]
          n77 = call "Read WPSEL.vi"("error in (no error)"=w159, "Instrument in"=w176) -> ("error out"=w184:errorcluster, "Opt_Selector.lvclass"=w183:refnum<class "Opt_Selector.lvclass">, "Instrument out"=w175:refnum<class "Instrument.lvclass">)  [unwired: 7 in]
          n78 = call-dynamic "Read State Machine.vi"("error in (no error)"=w184, "Device in"=w183) -> ("error out"=w187:errorcluster, "State Machine.lvclass"=w189:refnum<class "State Machine.lvclass">, "Device out"=w181:refnum<class "Opt_Selector.lvclass">)  [unwired: 7 in]
          n79 = call "Next State.vi"("error in (no error)"=w187, "New_State"=1, "State Machine in"=w189) -> ("error out"=w186:errorcluster, "State Machine out"=w185:refnum<class "State Machine.lvclass">)  [unwired: 7 in]
          n80 = call-dynamic "Write State Machine.vi"("error in (no error)"=w186, "State Machine.lvclass"=w185, "Device in"=w181) -> ("error out"=w180:errorcluster, "Device out"=w182:refnum<class "Opt_Selector.lvclass">)  [unwired: 7 in]
          n81 = call "Write WPSEL.vi"("error in (no error)"=w180, "Opt_Selector.lvclass"=w182, "Instrument in"=w175) -> ("error out"=w158:errorcluster, "Instrument out"=w164:refnum<class "Instrument.lvclass">)  [unwired: 7 in]
          n82 = call "Read WPROT.vi"("error in (no error)"=w158, "Instrument in"=w164) -> ("error out"=w170:errorcluster, "Opt_Selector.lvclass"=w171:refnum<class "Opt_Selector.lvclass">, "Instrument out"=w163:refnum<class "Instrument.lvclass">)  [unwired: 7 in]
          n83 = call-dynamic "Read State Machine.vi"("error in (no error)"=w170, "Device in"=w171) -> ("error out"=w167:errorcluster, "State Machine.lvclass"=w165:refnum<class "State Machine.lvclass">, "Device out"=w173:refnum<class "Opt_Selector.lvclass">)  [unwired: 7 in]
          n84 = call "Next State.vi"("error in (no error)"=w167, "New_State"=1, "State Machine in"=w165) -> ("error out"=w168:errorcluster, "State Machine out"=w169:refnum<class "State Machine.lvclass">)  [unwired: 7 in]
          n85 = call-dynamic "Write State Machine.vi"("error in (no error)"=w168, "State Machine.lvclass"=w169, "Device in"=w173) -> ("error out"=w174:errorcluster, "Device out"=w172:refnum<class "Opt_Selector.lvclass">)  [unwired: 7 in]
          n86 = call "Write WPROT.vi"("error in (no error)"=w174, "Opt_Selector.lvclass"=w172, "Instrument in"=w163) -> ("error out"=w161:errorcluster, "Instrument out"=w162:refnum<class "Instrument.lvclass">)  [unwired: 7 in]
          n87 = call "Write Instrument.lvclass.vi"("error in (no error)"=w161, "Instrument.lvclass"=w162, "S4ACS_GUI in"=w217) -> ("error out"=w214:errorcluster, "S4ACS_GUI out"=w203:refnum<class "S4GUI.lvclass">)  [unwired: 7 in]
          n88 = Bundle By Name(cluster=w203, "Obs_state"=w201) -> (w200:refnum<class "S4GUI.lvclass">)
        }
        frame 201 {
          # "Espera terminar a execução dos comandos ."
          n89 = call "Read Instrument.lvclass.vi"("error in (no error)"=w282, "S4ACS_GUI in"=w283) -> ("error out"=w286:errorcluster, "Instrument.lvclass"=w287:refnum<class "Instrument.lvclass">, "S4ACS_GUI out"=w284:refnum<class "S4GUI.lvclass">)  [unwired: 7 in]
          n90 = call "Read ASEL.vi"("error in (no error)"=w286, "Instrument in"=w287) -> ("error out"=w276:errorcluster, "Opt_Selector.lvclass"=w275:refnum<class "Opt_Selector.lvclass">, "Instrument out"=w285:refnum<class "Instrument.lvclass">)  [unwired: 7 in]
          n91 = call-dynamic "Read State Machine.vi"("error in (no error)"=w276, "Device in"=w275) -> ("error out"=w279:errorcluster, "State Machine.lvclass"=w280:refnum<class "State Machine.lvclass">, "Device out"=w273:refnum<class "Opt_Selector.lvclass">)  [unwired: 7 in]
          n92 = call-dynamic "Read State.vi"("error in (no error)"=w279, "State Machine in"=w280) -> ("error out"=w278:errorcluster, "State"=w269:i32, "State Machine out"=w277:refnum<class "State Machine.lvclass">)  [unwired: 7 in]
          n93 = Equal To 0?(x=w269) -> (x = 0?=w264:bool)
          n94 = call-dynamic "Write State Machine.vi"("error in (no error)"=w278, "State Machine.lvclass"=w277, "Device in"=w273) -> ("error out"=w272:errorcluster, "Device out"=w274:refnum<class "Opt_Selector.lvclass">)  [unwired: 7 in]
          n95 = call "Write ASEL.vi"("error in (no error)"=w272, "Opt_Selector.lvclass"=w274, "Instrument in"=w285) -> ("error out"=w226:errorcluster, "Instrument out"=w227:refnum<class "Instrument.lvclass">)  [unwired: 7 in]
          n96 = call "Read CALW.vi"("error in (no error)"=w226, "Instrument in"=w227) -> ("error out"=w259:errorcluster, "Opt_Selector.lvclass"=w260:refnum<class "Opt_Selector.lvclass">, "Instrument out"=w230:refnum<class "Instrument.lvclass">)  [unwired: 7 in]
          n97 = call-dynamic "Read State Machine.vi"("error in (no error)"=w259, "Device in"=w260) -> ("error out"=w256:errorcluster, "State Machine.lvclass"=w255:refnum<class "State Machine.lvclass">, "Device out"=w262:refnum<class "Opt_Selector.lvclass">)  [unwired: 7 in]
          n98 = call-dynamic "Read State.vi"("error in (no error)"=w256, "State Machine in"=w255) -> ("error out"=w257:errorcluster, "State"=w254:i32, "State Machine out"=w258:refnum<class "State Machine.lvclass">)  [unwired: 7 in]
          n99 = Equal To 0?(x=w254) -> (x = 0?=w253:bool)
          n100 = call-dynamic "Write State Machine.vi"("error in (no error)"=w257, "State Machine.lvclass"=w258, "Device in"=w262) -> ("error out"=w263:errorcluster, "Device out"=w261:refnum<class "Opt_Selector.lvclass">)  [unwired: 7 in]
          n101 = call "Write CALW.vi"("error in (no error)"=w263, "Opt_Selector.lvclass"=w261, "Instrument in"=w230) -> ("error out"=w224:errorcluster, "Instrument out"=w225:refnum<class "Instrument.lvclass">)  [unwired: 7 in]
          n102 = call "Read WPSEL.vi"("error in (no error)"=w224, "Instrument in"=w225) -> ("error out"=w247:errorcluster, "Opt_Selector.lvclass"=w246:refnum<class "Opt_Selector.lvclass">, "Instrument out"=w229:refnum<class "Instrument.lvclass">)  [unwired: 7 in]
          n103 = call-dynamic "Read State Machine.vi"("error in (no error)"=w247, "Device in"=w246) -> ("error out"=w250:errorcluster, "State Machine.lvclass"=w251:refnum<class "State Machine.lvclass">, "Device out"=w244:refnum<class "Opt_Selector.lvclass">)  [unwired: 7 in]
          n104 = call-dynamic "Read State.vi"("error in (no error)"=w250, "State Machine in"=w251) -> ("error out"=w249:errorcluster, "State"=w252:i32, "State Machine out"=w248:refnum<class "State Machine.lvclass">)  [unwired: 7 in]
          n105 = Equal To 0?(x=w252) -> (x = 0?=w232:bool)
          n106 = call-dynamic "Write State Machine.vi"("error in (no error)"=w249, "State Machine.lvclass"=w248, "Device in"=w244) -> ("error out"=w243:errorcluster, "Device out"=w245:refnum<class "Opt_Selector.lvclass">)  [unwired: 7 in]
          n107 = call "Write WPSEL.vi"("error in (no error)"=w243, "Opt_Selector.lvclass"=w245, "Instrument in"=w229) -> ("error out"=w222:errorcluster, "Instrument out"=w223:refnum<class "Instrument.lvclass">)  [unwired: 7 in]
          n108 = call "Read WPROT.vi"("error in (no error)"=w222, "Instrument in"=w223) -> ("error out"=w238:errorcluster, "Opt_Selector.lvclass"=w239:refnum<class "Opt_Selector.lvclass">, "Instrument out"=w228:refnum<class "Instrument.lvclass">)  [unwired: 7 in]
          n109 = call-dynamic "Read State Machine.vi"("error in (no error)"=w238, "Device in"=w239) -> ("error out"=w235:errorcluster, "State Machine.lvclass"=w234:refnum<class "State Machine.lvclass">, "Device out"=w241:refnum<class "Opt_Selector.lvclass">)  [unwired: 7 in]
          n110 = call-dynamic "Read State.vi"("error in (no error)"=w235, "State Machine in"=w234) -> ("error out"=w236:errorcluster, "State"=w233:i32, "State Machine out"=w237:refnum<class "State Machine.lvclass">)  [unwired: 7 in]
          n111 = Equal To 0?(x=w233) -> (x = 0?=w231:bool)
          n112 = call-dynamic "Write State Machine.vi"("error in (no error)"=w236, "State Machine.lvclass"=w237, "Device in"=w241) -> ("error out"=w242:errorcluster, "Device out"=w240:refnum<class "Opt_Selector.lvclass">)  [unwired: 7 in]
          n113 = call "Write WPROT.vi"("error in (no error)"=w242, "Opt_Selector.lvclass"=w240, "Instrument in"=w228) -> ("error out"=w220:errorcluster, "Instrument out"=w221:refnum<class "Instrument.lvclass">)  [unwired: 7 in]
          n114 = Compound Arithmetic op=AND(w264, w253, w232, w231) -> (w266:bool)
          n115 = Select(t=u32 0, s=w266, f=w265) -> (s? t:f=w268:u32)
          n116 = call "Write Instrument.lvclass.vi"("error in (no error)"=w220, "Instrument.lvclass"=w221, "S4ACS_GUI in"=w284) -> ("error out"=w281:errorcluster, "S4ACS_GUI out"=w271:refnum<class "S4GUI.lvclass">)  [unwired: 7 in]
          n117 = Bundle By Name(cluster=w271, "Obs_state"=w268) -> (w270:refnum<class "S4GUI.lvclass">)
        }
        frame 202 {
          # "Dispara o comando para o dispositivo corrente."
          n118 = call "Read Instrument.lvclass.vi"("error in (no error)"=w303, "S4ACS_GUI in"=w304) -> ("error out"=w309:errorcluster, "Instrument.lvclass"=w310:refnum<class "Instrument.lvclass">, "S4ACS_GUI out"=w306:refnum<class "S4GUI.lvclass">)  [unwired: 7 in]
          n119 = call "Read CALW.vi"("error in (no error)"=w309, "Instrument in"=w310) -> ("error out"=w296:errorcluster, "Opt_Selector.lvclass"=w295:refnum<class "Opt_Selector.lvclass">, "Instrument out"=w308:refnum<class "Instrument.lvclass">)  [unwired: 7 in]
          n120 = call-dynamic "Read State Machine.vi"("error in (no error)"=w296, "Device in"=w295) -> ("error out"=w299:errorcluster, "State Machine.lvclass"=w301:refnum<class "State Machine.lvclass">, "Device out"=w293:refnum<class "Opt_Selector.lvclass">)  [unwired: 7 in]
          n121 = call "Next State.vi"("error in (no error)"=w299, "New_State"=1, "State Machine in"=w301) -> ("error out"=w298:errorcluster, "State Machine out"=w297:refnum<class "State Machine.lvclass">)  [unwired: 7 in]
          n122 = call-dynamic "Write State Machine.vi"("error in (no error)"=w298, "State Machine.lvclass"=w297, "Device in"=w293) -> ("error out"=w292:errorcluster, "Device out"=w294:refnum<class "Opt_Selector.lvclass">)  [unwired: 7 in]
          n123 = Increment(x=w290) -> (x+1=w289:u32)
          n124 = call "Write CALW.vi"("error in (no error)"=w292, "Opt_Selector.lvclass"=w294, "Instrument in"=w308) -> ("error out"=w305:errorcluster, "Instrument out"=w307:refnum<class "Instrument.lvclass">)  [unwired: 7 in]
          n125 = call "Write Instrument.lvclass.vi"("error in (no error)"=w305, "Instrument.lvclass"=w307, "S4ACS_GUI in"=w306) -> ("error out"=w302:errorcluster, "S4ACS_GUI out"=w291:refnum<class "S4GUI.lvclass">)  [unwired: 7 in]
          n126 = Bundle By Name(cluster=w291, "Obs_state"=w289) -> (w288:refnum<class "S4GUI.lvclass">)
        }
        frame 203 {
          # "Espera terminar a execução do comando atual \nantes de ir ao proximo passo da Observação."
          n127 = call "Read Instrument.lvclass.vi"("error in (no error)"=w328, "S4ACS_GUI in"=w329) -> ("error out"=w334:errorcluster, "Instrument.lvclass"=w335:refnum<class "Instrument.lvclass">, "S4ACS_GUI out"=w331:refnum<class "S4GUI.lvclass">)  [unwired: 7 in]
          n128 = call "Read CALW.vi"("error in (no error)"=w334, "Instrument in"=w335) -> ("error out"=w322:errorcluster, "Opt_Selector.lvclass"=w321:refnum<class "Opt_Selector.lvclass">, "Instrument out"=w333:refnum<class "Instrument.lvclass">)  [unwired: 7 in]
          n129 = call-dynamic "Read State Machine.vi"("error in (no error)"=w322, "Device in"=w321) -> ("error out"=w325:errorcluster, "State Machine.lvclass"=w326:refnum<class "State Machine.lvclass">, "Device out"=w319:refnum<class "Opt_Selector.lvclass">)  [unwired: 7 in]
          n130 = Increment(x=w312) -> (x+1=w311:u32)
          n131 = call-dynamic "Read State.vi"("error in (no error)"=w325, "State Machine in"=w326) -> ("error out"=w324:errorcluster, "State"=w314:i32, "State Machine out"=w323:refnum<class "State Machine.lvclass">)  [unwired: 7 in]
          n132 = Equal To 0?(x=w314) -> (x = 0?=w315:bool)
          n133 = call-dynamic "Write State Machine.vi"("error in (no error)"=w324, "State Machine.lvclass"=w323, "Device in"=w319) -> ("error out"=w318:errorcluster, "Device out"=w320:refnum<class "Opt_Selector.lvclass">)  [unwired: 7 in]
          n134 = call "Write CALW.vi"("error in (no error)"=w318, "Opt_Selector.lvclass"=w320, "Instrument in"=w333) -> ("error out"=w330:errorcluster, "Instrument out"=w332:refnum<class "Instrument.lvclass">)  [unwired: 7 in]
          n135 = Select(t=w311, s=w315, f=w312) -> (s? t:f=w313:u32)
          n136 = call "Write Instrument.lvclass.vi"("error in (no error)"=w330, "Instrument.lvclass"=w332, "S4ACS_GUI in"=w331) -> ("error out"=w327:errorcluster, "S4ACS_GUI out"=w317:refnum<class "S4GUI.lvclass">)  [unwired: 7 in]
          n137 = Bundle By Name(cluster=w317, "Obs_state"=w313) -> (w316:refnum<class "S4GUI.lvclass">)
        }
        frame 204 {
          # "Dispara o comando para o dispositivo corrente."
          n138 = call "Read Instrument.lvclass.vi"("error in (no error)"=w351, "S4ACS_GUI in"=w352) -> ("error out"=w357:errorcluster, "Instrument.lvclass"=w358:refnum<class "Instrument.lvclass">, "S4ACS_GUI out"=w354:refnum<class "S4GUI.lvclass">)  [unwired: 7 in]
          n139 = call "Read WPSEL.vi"("error in (no error)"=w357, "Instrument in"=w358) -> ("error out"=w344:errorcluster, "Opt_Selector.lvclass"=w343:refnum<class "Opt_Selector.lvclass">, "Instrument out"=w356:refnum<class "Instrument.lvclass">)  [unwired: 7 in]
          n140 = call-dynamic "Read State Machine.vi"("error in (no error)"=w344, "Device in"=w343) -> ("error out"=w347:errorcluster, "State Machine.lvclass"=w349:refnum<class "State Machine.lvclass">, "Device out"=w341:refnum<class "Opt_Selector.lvclass">)  [unwired: 7 in]
          n141 = call "Next State.vi"("error in (no error)"=w347, "New_State"=1, "State Machine in"=w349) -> ("error out"=w346:errorcluster, "State Machine out"=w345:refnum<class "State Machine.lvclass">)  [unwired: 7 in]
          n142 = call-dynamic "Write State Machine.vi"("error in (no error)"=w346, "State Machine.lvclass"=w345, "Device in"=w341) -> ("error out"=w340:errorcluster, "Device out"=w342:refnum<class "Opt_Selector.lvclass">)  [unwired: 7 in]
          n143 = Increment(x=w338) -> (x+1=w337:u32)
          n144 = call "Write WPSEL.vi"("error in (no error)"=w340, "Opt_Selector.lvclass"=w342, "Instrument in"=w356) -> ("error out"=w353:errorcluster, "Instrument out"=w355:refnum<class "Instrument.lvclass">)  [unwired: 7 in]
          n145 = call "Write Instrument.lvclass.vi"("error in (no error)"=w353, "Instrument.lvclass"=w355, "S4ACS_GUI in"=w354) -> ("error out"=w350:errorcluster, "S4ACS_GUI out"=w339:refnum<class "S4GUI.lvclass">)  [unwired: 7 in]
          n146 = Bundle By Name(cluster=w339, "Obs_state"=w337) -> (w336:refnum<class "S4GUI.lvclass">)
        }
        frame 205 {
          # "Espera terminar a execução do comando atual \nantes de ir ao proximo passo da Observação."
          n147 = call "Read Instrument.lvclass.vi"("error in (no error)"=w376, "S4ACS_GUI in"=w377) -> ("error out"=w382:errorcluster, "Instrument.lvclass"=w383:refnum<class "Instrument.lvclass">, "S4ACS_GUI out"=w379:refnum<class "S4GUI.lvclass">)  [unwired: 7 in]
          n148 = call "Read WPSEL.vi"("error in (no error)"=w382, "Instrument in"=w383) -> ("error out"=w370:errorcluster, "Opt_Selector.lvclass"=w369:refnum<class "Opt_Selector.lvclass">, "Instrument out"=w381:refnum<class "Instrument.lvclass">)  [unwired: 7 in]
          n149 = call-dynamic "Read State Machine.vi"("error in (no error)"=w370, "Device in"=w369) -> ("error out"=w373:errorcluster, "State Machine.lvclass"=w374:refnum<class "State Machine.lvclass">, "Device out"=w367:refnum<class "Opt_Selector.lvclass">)  [unwired: 7 in]
          n150 = Increment(x=w360) -> (x+1=w359:u32)
          n151 = call-dynamic "Read State.vi"("error in (no error)"=w373, "State Machine in"=w374) -> ("error out"=w372:errorcluster, "State"=w362:i32, "State Machine out"=w371:refnum<class "State Machine.lvclass">)  [unwired: 7 in]
          n152 = Equal To 0?(x=w362) -> (x = 0?=w363:bool)
          n153 = call-dynamic "Write State Machine.vi"("error in (no error)"=w372, "State Machine.lvclass"=w371, "Device in"=w367) -> ("error out"=w366:errorcluster, "Device out"=w368:refnum<class "Opt_Selector.lvclass">)  [unwired: 7 in]
          n154 = call "Write WPSEL.vi"("error in (no error)"=w366, "Opt_Selector.lvclass"=w368, "Instrument in"=w381) -> ("error out"=w378:errorcluster, "Instrument out"=w380:refnum<class "Instrument.lvclass">)  [unwired: 7 in]
          n155 = Select(t=w359, s=w363, f=w360) -> (s? t:f=w361:u32)
          n156 = call "Write Instrument.lvclass.vi"("error in (no error)"=w378, "Instrument.lvclass"=w380, "S4ACS_GUI in"=w379) -> ("error out"=w375:errorcluster, "S4ACS_GUI out"=w365:refnum<class "S4GUI.lvclass">)  [unwired: 7 in]
          n157 = Bundle By Name(cluster=w365, "Obs_state"=w361) -> (w364:refnum<class "S4GUI.lvclass">)
        }
        frame 206 {
          # "Dispara o comando para o dispositivo corrente."
          n158 = call "Read Instrument.lvclass.vi"("error in (no error)"=w398, "S4ACS_GUI in"=w399) -> ("error out"=w404:errorcluster, "Instrument.lvclass"=w405:refnum<class "Instrument.lvclass">, "S4ACS_GUI out"=w401:refnum<class "S4GUI.lvclass">)  [unwired: 7 in]
          n159 = call "Read WPSEL.vi"("error in (no error)"=w404, "Instrument in"=w405) -> ("error out"=w392:errorcluster, "Opt_Selector.lvclass"=w393:refnum<class "Opt_Selector.lvclass">, "Instrument out"=w403:refnum<class "Instrument.lvclass">)  [unwired: 7 in]
          n160 = call "Read target name.vi"("error in (no error)"=w392, "Optics in"=w393) -> ("error out"=w386:errorcluster, "target name"=w391:string, "Optics out"=w385:refnum<class "Opt_Selector.lvclass">)  [unwired: 7 in]
          n161 = Equal?(x=w391, y="OFF") -> (x = y?=w389:bool)
          n162 = Increment(x=w395) -> (x+1=w387:u32)
          n163 = call "Write WPSEL.vi"("error in (no error)"=w386, "Opt_Selector.lvclass"=w385, "Instrument in"=w403) -> ("error out"=w400:errorcluster, "Instrument out"=w402:refnum<class "Instrument.lvclass">)  [unwired: 7 in]
          n164 = Select(t=u32 0, s=w389, f=w387) -> (s? t:f=w384:u32)
          n165 = call "Write Instrument.lvclass.vi"("error in (no error)"=w400, "Instrument.lvclass"=w402, "S4ACS_GUI in"=w401) -> ("error out"=w397:errorcluster, "S4ACS_GUI out"=w396:refnum<class "S4GUI.lvclass">)  [unwired: 7 in]
          n166 = Bundle By Name(cluster=w396, "Obs_state"=w384) -> (w394:refnum<class "S4GUI.lvclass">)
        }
        frame 207 {
          # "Dispara o comando para o dispositivo corrente."
          n167 = call "Read Instrument.lvclass.vi"("error in (no error)"=w421, "S4ACS_GUI in"=w422) -> ("error out"=w427:errorcluster, "Instrument.lvclass"=w428:refnum<class "Instrument.lvclass">, "S4ACS_GUI out"=w424:refnum<class "S4GUI.lvclass">)  [unwired: 7 in]
          n168 = call "Read WPROT.vi"("error in (no error)"=w427, "Instrument in"=w428) -> ("error out"=w414:errorcluster, "Opt_Selector.lvclass"=w413:refnum<class "Opt_Selector.lvclass">, "Instrument out"=w426:refnum<class "Instrument.lvclass">)  [unwired: 7 in]
          n169 = call-dynamic "Read State Machine.vi"("error in (no error)"=w414, "Device in"=w413) -> ("error out"=w417:errorcluster, "State Machine.lvclass"=w419:refnum<class "State Machine.lvclass">, "Device out"=w411:refnum<class "Opt_Selector.lvclass">)  [unwired: 7 in]
          n170 = call "Next State.vi"("error in (no error)"=w417, "New_State"=1, "State Machine in"=w419) -> ("error out"=w416:errorcluster, "State Machine out"=w415:refnum<class "State Machine.lvclass">)  [unwired: 7 in]
          n171 = call-dynamic "Write State Machine.vi"("error in (no error)"=w416, "State Machine.lvclass"=w415, "Device in"=w411) -> ("error out"=w410:errorcluster, "Device out"=w412:refnum<class "Opt_Selector.lvclass">)  [unwired: 7 in]
          n172 = Increment(x=w408) -> (x+1=w407:u32)
          n173 = call "Write WPROT.vi"("error in (no error)"=w410, "Opt_Selector.lvclass"=w412, "Instrument in"=w426) -> ("error out"=w423:errorcluster, "Instrument out"=w425:refnum<class "Instrument.lvclass">)  [unwired: 7 in]
          n174 = call "Write Instrument.lvclass.vi"("error in (no error)"=w423, "Instrument.lvclass"=w425, "S4ACS_GUI in"=w424) -> ("error out"=w420:errorcluster, "S4ACS_GUI out"=w409:refnum<class "S4GUI.lvclass">)  [unwired: 7 in]
          n175 = Bundle By Name(cluster=w409, "Obs_state"=w407) -> (w406:refnum<class "S4GUI.lvclass">)
        }
        frame 208 {
          # "Espera terminar a execução do comando atual \nantes de ir ao proximo passo da Observação."
          n176 = call "Read Instrument.lvclass.vi"("error in (no error)"=w446, "S4ACS_GUI in"=w447) -> ("error out"=w452:errorcluster, "Instrument.lvclass"=w453:refnum<class "Instrument.lvclass">, "S4ACS_GUI out"=w449:refnum<class "S4GUI.lvclass">)  [unwired: 7 in]
          n177 = call "Read WPROT.vi"("error in (no error)"=w452, "Instrument in"=w453) -> ("error out"=w440:errorcluster, "Opt_Selector.lvclass"=w439:refnum<class "Opt_Selector.lvclass">, "Instrument out"=w451:refnum<class "Instrument.lvclass">)  [unwired: 7 in]
          n178 = call-dynamic "Read State Machine.vi"("error in (no error)"=w440, "Device in"=w439) -> ("error out"=w443:errorcluster, "State Machine.lvclass"=w444:refnum<class "State Machine.lvclass">, "Device out"=w437:refnum<class "Opt_Selector.lvclass">)  [unwired: 7 in]
          n179 = call-dynamic "Read State.vi"("error in (no error)"=w443, "State Machine in"=w444) -> ("error out"=w442:errorcluster, "State"=w432:i32, "State Machine out"=w441:refnum<class "State Machine.lvclass">)  [unwired: 7 in]
          n180 = Equal To 0?(x=w432) -> (x = 0?=w433:bool)
          n181 = call-dynamic "Write State Machine.vi"("error in (no error)"=w442, "State Machine.lvclass"=w441, "Device in"=w437) -> ("error out"=w436:errorcluster, "Device out"=w438:refnum<class "Opt_Selector.lvclass">)  [unwired: 7 in]
          n182 = call "Write WPSEL.vi"("error in (no error)"=w436, "Opt_Selector.lvclass"=w438, "Instrument in"=w451) -> ("error out"=w448:errorcluster, "Instrument out"=w450:refnum<class "Instrument.lvclass">)  [unwired: 7 in]
          n183 = Select(t=u32 0, s=w433, f=w430) -> (s? t:f=w431:u32)
          n184 = call "Write Instrument.lvclass.vi"("error in (no error)"=w448, "Instrument.lvclass"=w450, "S4ACS_GUI in"=w449) -> ("error out"=w445:errorcluster, "S4ACS_GUI out"=w435:refnum<class "S4GUI.lvclass">)  [unwired: 7 in]
          n185 = Bundle By Name(cluster=w435, "Obs_state"=w431) -> (w434:refnum<class "S4GUI.lvclass">)
        }
        frame 220 {
          n186 = call "Read Instrument.lvclass.vi"("error in (no error)"=w500, "S4ACS_GUI in"=w501) -> ("error out"=w460:errorcluster, "Instrument.lvclass"=w461:refnum<class "Instrument.lvclass">, "S4ACS_GUI out"=w502:refnum<class "S4GUI.lvclass">)  [unwired: 7 in]
          n187 = call "Read WPSEL.vi"("error in (no error)"=w460, "Instrument in"=w461) -> ("error out"=w486:errorcluster, "Opt_Selector.lvclass"=w487:refnum<class "Opt_Selector.lvclass">, "Instrument out"=w494:refnum<class "Instrument.lvclass">)  [unwired: 7 in]
          n188 = call-dynamic "Read State Machine.vi"("error in (no error)"=w486, "Device in"=w487) -> ("error out"=w489:errorcluster, "State Machine.lvclass"=w491:refnum<class "State Machine.lvclass">, "Device out"=w488:refnum<class "Opt_Selector.lvclass">)  [unwired: 7 in]
          n189 = call "Next State.vi"("error in (no error)"=w489, "New_State"=30, "State Machine in"=w491) -> ("error out"=w485:errorcluster, "State Machine out"=w484:refnum<class "State Machine.lvclass">)  [unwired: 7 in]
          n190 = call-dynamic "Write State Machine.vi"("error in (no error)"=w485, "State Machine.lvclass"=w484, "Device in"=w488) -> ("error out"=w493:errorcluster, "Device out"=w495:refnum<class "Opt_Selector.lvclass">)  [unwired: 7 in]
          n191 = Increment(x=w492) -> (x+1=w497:u32)
          n192 = call "Write WPSEL.vi"("error in (no error)"=w493, "Opt_Selector.lvclass"=w495, "Instrument in"=w494) -> ("error out"=w458:errorcluster, "Instrument out"=w459:refnum<class "Instrument.lvclass">)  [unwired: 7 in]
          n193 = call "Read CALW.vi"("error in (no error)"=w458, "Instrument in"=w459) -> ("error out"=w475:errorcluster, "Opt_Selector.lvclass"=w476:refnum<class "Opt_Selector.lvclass">, "Instrument out"=w482:refnum<class "Instrument.lvclass">)  [unwired: 7 in]
          n194 = call-dynamic "Read State Machine.vi"("error in (no error)"=w475, "Device in"=w476) -> ("error out"=w478:errorcluster, "State Machine.lvclass"=w480:refnum<class "State Machine.lvclass">, "Device out"=w477:refnum<class "Opt_Selector.lvclass">)  [unwired: 7 in]
          n195 = call "Next State.vi"("error in (no error)"=w478, "New_State"=30, "State Machine in"=w480) -> ("error out"=w474:errorcluster, "State Machine out"=w473:refnum<class "State Machine.lvclass">)  [unwired: 7 in]
          n196 = call-dynamic "Write State Machine.vi"("error in (no error)"=w474, "State Machine.lvclass"=w473, "Device in"=w477) -> ("error out"=w481:errorcluster, "Device out"=w483:refnum<class "Opt_Selector.lvclass">)  [unwired: 7 in]
          n197 = call "Write CALW.vi"("error in (no error)"=w481, "Opt_Selector.lvclass"=w483, "Instrument in"=w482) -> ("error out"=w456:errorcluster, "Instrument out"=w457:refnum<class "Instrument.lvclass">)  [unwired: 7 in]
          n198 = call "Read GMIR.vi"("error in (no error)"=w456, "Instrument in"=w457) -> ("error out"=w464:errorcluster, "Opt_Continuous.lvclass"=w465:refnum<class "Opt_Continuous.lvclass">, "Instrument out"=w471:refnum<class "Instrument.lvclass">)  [unwired: 7 in]
          n199 = call-dynamic "Read State Machine.vi"("error in (no error)"=w464, "Device in"=w465) -> ("error out"=w467:errorcluster, "State Machine.lvclass"=w469:refnum<class "State Machine.lvclass">, "Device out"=w466:refnum<class "Opt_Continuous.lvclass">)  [unwired: 7 in]
          n200 = call "Next State.vi"("error in (no error)"=w467, "New_State"=30, "State Machine in"=w469) -> ("error out"=w463:errorcluster, "State Machine out"=w462:refnum<class "State Machine.lvclass">)  [unwired: 7 in]
          n201 = call-dynamic "Write State Machine.vi"("error in (no error)"=w463, "State Machine.lvclass"=w462, "Device in"=w466) -> ("error out"=w470:errorcluster, "Device out"=w472:refnum<class "Opt_Continuous.lvclass">)  [unwired: 7 in]
          n202 = call "Write GMIR.vi"("error in (no error)"=w470, "Opt_Continuous.lvclass"=w472, "Instrument in"=w471) -> ("error out"=w455:errorcluster, "Instrument out"=w454:refnum<class "Instrument.lvclass">)  [unwired: 7 in]
          n203 = call "Write Instrument.lvclass.vi"("error in (no error)"=w455, "Instrument.lvclass"=w454, "S4ACS_GUI in"=w502) -> ("error out"=w499:errorcluster, "S4ACS_GUI out"=w498:refnum<class "S4GUI.lvclass">)  [unwired: 7 in]
          n204 = Bundle By Name(cluster=w498, "Obs_state"=w497) -> (w496:refnum<class "S4GUI.lvclass">)
        }
        frame 221 {
          # "Espera terminar o homing de WPSEL,CALW e GMIR\nantes de seguir para o próximo estado."
          n205 = call "Read Instrument.lvclass.vi"("error in (no error)"=w531, "S4ACS_GUI in"=w532) -> ("error out"=w513:errorcluster, "Instrument.lvclass"=w514:refnum<class "Instrument.lvclass">, "S4ACS_GUI out"=w522:refnum<class "S4GUI.lvclass">)  [unwired: 7 in]
          n206 = call "Read CALW.vi"("error in (no error)"=w513, "Instrument in"=w514) -> ("error out"=w518:errorcluster, "Opt_Selector.lvclass"=w504:refnum<class "Opt_Selector.lvclass">)  [unwired: 7 in, 1 out]
          n207 = call "Read GMIR.vi"("error in (no error)"=w513, "Instrument in"=w514) -> ("error out"=w515:errorcluster, "Opt_Continuous.lvclass"=w503:refnum<class "Opt_Continuous.lvclass">)  [unwired: 7 in, 1 out]
          n208 = call "Read WPSEL.vi"("error in (no error)"=w513, "Instrument in"=w514) -> ("error out"=w528:errorcluster, "Opt_Selector.lvclass"=w527:refnum<class "Opt_Selector.lvclass">)  [unwired: 7 in, 1 out]
          n209 = call-dynamic "Read State Machine.vi"("error in (no error)"=w518, "Device in"=w504) -> ("error out"=w519:errorcluster, "State Machine.lvclass"=w520:refnum<class "State Machine.lvclass">)  [unwired: 7 in, 1 out]
          n210 = call-dynamic "Read State Machine.vi"("error in (no error)"=w515, "Device in"=w503) -> ("error out"=w516:errorcluster, "State Machine.lvclass"=w517:refnum<class "State Machine.lvclass">)  [unwired: 7 in, 1 out]
          n211 = call-dynamic "Read State Machine.vi"("error in (no error)"=w528, "Device in"=w527) -> ("error out"=w529:errorcluster, "State Machine.lvclass"=w530:refnum<class "State Machine.lvclass">)  [unwired: 7 in, 1 out]
          n212 = Increment(x=w524) -> (x+1=w523:u32)
          n213 = call-dynamic "Read State.vi"("error in (no error)"=w519, "State Machine in"=w520) -> ("error out"=w507:errorcluster, "State"=w511:i32)  [unwired: 7 in, 1 out]
          n214 = call-dynamic "Read State.vi"("error in (no error)"=w516, "State Machine in"=w517) -> ("error out"=w506:errorcluster, "State"=w510:i32)  [unwired: 7 in, 1 out]
          n215 = call-dynamic "Read State.vi"("error in (no error)"=w529, "State Machine in"=w530) -> ("error out"=w521:errorcluster, "State"=w512:i32)  [unwired: 7 in, 1 out]
          n216 = Compound Arithmetic op=ADD(w512, w511, w510) -> (w509:i32)
          n217 = Equal To 0?(x=w509) -> (x = 0?=w508:bool)
          n218 = Merge Errors(w521, w507, w506) -> (w505:errorcluster)
          n219 = Select(t=w523, s=w508, f=w524) -> (s? t:f=w525:u32)
          n220 = Bundle By Name(cluster=w522, "Obs_state"=w525) -> (w526:refnum<class "S4GUI.lvclass">)
        }
        frame 222 {
          # "Manda WPSEL para L/2"
          n221 = call "Read Instrument.lvclass.vi"("error in (no error)"=w559, "S4ACS_GUI in"=w560) -> ("error out"=w543:errorcluster, "Instrument.lvclass"=w544:refnum<class "Instrument.lvclass">, "S4ACS_GUI out"=w561:refnum<class "S4GUI.lvclass">)  [unwired: 7 in]
          n222 = call "Read WPSEL.vi"("error in (no error)"=w543, "Instrument in"=w544) -> ("error out"=w539:errorcluster, "Opt_Selector.lvclass"=w538:refnum<class "Opt_Selector.lvclass">, "Instrument out"=w553:refnum<class "Instrument.lvclass">)  [unwired: 7 in]
          n223 = call "Write target.vi"("error in (no error)"=w539, "target"=0.0, "Optics in"=w538) -> ("error out"=w542:errorcluster, "Optics out"=w537:refnum<class "Opt_Selector.lvclass">)  [unwired: 7 in]
          n224 = call "Write target name.vi"("error in (no error)"=w542, "target name"="L/2", "Optics in"=w537) -> ("error out"=w535:errorcluster, "Optics out"=w536:refnum<class "Opt_Selector.lvclass">)  [unwired: 7 in]
          n225 = call-dynamic "Read State Machine.vi"("error in (no error)"=w535, "Device in"=w536) -> ("error out"=w548:errorcluster, "State Machine.lvclass"=w550:refnum<class "State Machine.lvclass">, "Device out"=w547:refnum<class "Opt_Selector.lvclass">)  [unwired: 7 in]
          n226 = call "Next State.vi"("error in (no error)"=w548, "New_State"=1, "State Machine in"=w550) -> ("error out"=w546:errorcluster, "State Machine out"=w545:refnum<class "State Machine.lvclass">)  [unwired: 7 in]
          n227 = call-dynamic "Write State Machine.vi"("error in (no error)"=w546, "State Machine.lvclass"=w545, "Device in"=w547) -> ("error out"=w552:errorcluster, "Device out"=w554:refnum<class "Opt_Selector.lvclass">)  [unwired: 7 in]
          n228 = Increment(x=w551) -> (x+1=w556:u32)
          n229 = call "Write WPSEL.vi"("error in (no error)"=w552, "Opt_Selector.lvclass"=w554, "Instrument in"=w553) -> ("error out"=w533:errorcluster, "Instrument out"=w534:refnum<class "Instrument.lvclass">)  [unwired: 7 in]
          n230 = call "Write Instrument.lvclass.vi"("error in (no error)"=w533, "Instrument.lvclass"=w534, "S4ACS_GUI in"=w561) -> ("error out"=w558:errorcluster, "S4ACS_GUI out"=w557:refnum<class "S4GUI.lvclass">)  [unwired: 7 in]
          n231 = Bundle By Name(cluster=w557, "Obs_state"=w556) -> (w555:refnum<class "S4GUI.lvclass">)
        }
        frame 223 {
          # "Espera terminar o movimento de WPSEL para L/2, \nantes de seguir para o próximo estado."
          n232 = call "Read Instrument.lvclass.vi"("error in (no error)"=w576, "S4ACS_GUI in"=w577) -> ("error out"=w565:errorcluster, "Instrument.lvclass"=w566:refnum<class "Instrument.lvclass">, "S4ACS_GUI out"=w567:refnum<class "S4GUI.lvclass">)  [unwired: 7 in]
          n233 = call "Read WPSEL.vi"("error in (no error)"=w565, "Instrument in"=w566) -> ("error out"=w573:errorcluster, "Opt_Selector.lvclass"=w572:refnum<class "Opt_Selector.lvclass">)  [unwired: 7 in, 1 out]
          n234 = call-dynamic "Read State Machine.vi"("error in (no error)"=w573, "Device in"=w572) -> ("error out"=w574:errorcluster, "State Machine.lvclass"=w575:refnum<class "State Machine.lvclass">)  [unwired: 7 in, 1 out]
          n235 = Increment(x=w569) -> (x+1=w568:u32)
          n236 = call-dynamic "Read State.vi"("error in (no error)"=w574, "State Machine in"=w575) -> ("error out"=w563:errorcluster, "State"=w562:i32)  [unwired: 7 in, 1 out]
          n237 = Equal To 0?(x=w562) -> (x = 0?=w564:bool)
          n238 = Select(t=w568, s=w564, f=w569) -> (s? t:f=w570:u32)
          n239 = Bundle By Name(cluster=w567, "Obs_state"=w570) -> (w571:refnum<class "S4GUI.lvclass">)
        }
        frame 224 {
          n240 = call "Read Instrument.lvclass.vi"("error in (no error)"=w624, "S4ACS_GUI in"=w625) -> ("error out"=w584:errorcluster, "Instrument.lvclass"=w585:refnum<class "Instrument.lvclass">, "S4ACS_GUI out"=w626:refnum<class "S4GUI.lvclass">)  [unwired: 7 in]
          n241 = call "Read WPROT.vi"("error in (no error)"=w584, "Instrument in"=w585) -> ("error out"=w610:errorcluster, "Opt_Selector.lvclass"=w611:refnum<class "Opt_Selector.lvclass">, "Instrument out"=w618:refnum<class "Instrument.lvclass">)  [unwired: 7 in]
          n242 = call-dynamic "Read State Machine.vi"("error in (no error)"=w610, "Device in"=w611) -> ("error out"=w613:errorcluster, "State Machine.lvclass"=w615:refnum<class "State Machine.lvclass">, "Device out"=w612:refnum<class "Opt_Selector.lvclass">)  [unwired: 7 in]
          n243 = call "Next State.vi"("error in (no error)"=w613, "New_State"=30, "State Machine in"=w615) -> ("error out"=w609:errorcluster, "State Machine out"=w608:refnum<class "State Machine.lvclass">)  [unwired: 7 in]
          n244 = call-dynamic "Write State Machine.vi"("error in (no error)"=w609, "State Machine.lvclass"=w608, "Device in"=w612) -> ("error out"=w617:errorcluster, "Device out"=w619:refnum<class "Opt_Selector.lvclass">)  [unwired: 7 in]
          n245 = Increment(x=w616) -> (x+1=w621:u32)
          n246 = call "Write WPROT.vi"("error in (no error)"=w617, "Opt_Selector.lvclass"=w619, "Instrument in"=w618) -> ("error out"=w582:errorcluster, "Instrument out"=w583:refnum<class "Instrument.lvclass">)  [unwired: 7 in]
          n247 = call "Read ASEL.vi"("error in (no error)"=w582, "Instrument in"=w583) -> ("error out"=w599:errorcluster, "Opt_Selector.lvclass"=w600:refnum<class "Opt_Selector.lvclass">, "Instrument out"=w606:refnum<class "Instrument.lvclass">)  [unwired: 7 in]
          n248 = call-dynamic "Read State Machine.vi"("error in (no error)"=w599, "Device in"=w600) -> ("error out"=w602:errorcluster, "State Machine.lvclass"=w604:refnum<class "State Machine.lvclass">, "Device out"=w601:refnum<class "Opt_Selector.lvclass">)  [unwired: 7 in]
          n249 = call "Next State.vi"("error in (no error)"=w602, "New_State"=30, "State Machine in"=w604) -> ("error out"=w598:errorcluster, "State Machine out"=w597:refnum<class "State Machine.lvclass">)  [unwired: 7 in]
          n250 = call-dynamic "Write State Machine.vi"("error in (no error)"=w598, "State Machine.lvclass"=w597, "Device in"=w601) -> ("error out"=w605:errorcluster, "Device out"=w607:refnum<class "Opt_Selector.lvclass">)  [unwired: 7 in]
          n251 = call "Write ASEL.vi"("error in (no error)"=w605, "Opt_Selector.lvclass"=w607, "Instrument in"=w606) -> ("error out"=w580:errorcluster, "Instrument out"=w581:refnum<class "Instrument.lvclass">)  [unwired: 7 in]
          n252 = call "Read GFOC.vi"("error in (no error)"=w580, "Instrument in"=w581) -> ("error out"=w588:errorcluster, "Opt_Continuous.lvclass"=w589:refnum<class "Opt_Continuous.lvclass">, "Instrument out"=w595:refnum<class "Instrument.lvclass">)  [unwired: 7 in]
          n253 = call-dynamic "Read State Machine.vi"("error in (no error)"=w588, "Device in"=w589) -> ("error out"=w591:errorcluster, "State Machine.lvclass"=w593:refnum<class "State Machine.lvclass">, "Device out"=w590:refnum<class "Opt_Continuous.lvclass">)  [unwired: 7 in]
          n254 = call "Next State.vi"("error in (no error)"=w591, "New_State"=30, "State Machine in"=w593) -> ("error out"=w587:errorcluster, "State Machine out"=w586:refnum<class "State Machine.lvclass">)  [unwired: 7 in]
          n255 = call-dynamic "Write State Machine.vi"("error in (no error)"=w587, "State Machine.lvclass"=w586, "Device in"=w590) -> ("error out"=w594:errorcluster, "Device out"=w596:refnum<class "Opt_Continuous.lvclass">)  [unwired: 7 in]
          n256 = call "Write GFOC.vi"("error in (no error)"=w594, "Opt_Continuous.lvclass"=w596, "Instrument in"=w595) -> ("error out"=w579:errorcluster, "Instrument out"=w578:refnum<class "Instrument.lvclass">)  [unwired: 7 in]
          n257 = call "Write Instrument.lvclass.vi"("error in (no error)"=w579, "Instrument.lvclass"=w578, "S4ACS_GUI in"=w626) -> ("error out"=w623:errorcluster, "S4ACS_GUI out"=w622:refnum<class "S4GUI.lvclass">)  [unwired: 7 in]
          n258 = Bundle By Name(cluster=w622, "Obs_state"=w621) -> (w620:refnum<class "S4GUI.lvclass">)
        }
        frame 225 {
          # "Espera terminar o homing de WPROT,ASEL e GFOC\nantes de seguir para o próximo estado."
          n259 = call "Read Instrument.lvclass.vi"("error in (no error)"=w655, "S4ACS_GUI in"=w656) -> ("error out"=w637:errorcluster, "Instrument.lvclass"=w638:refnum<class "Instrument.lvclass">, "S4ACS_GUI out"=w646:refnum<class "S4GUI.lvclass">)  [unwired: 7 in]
          n260 = call "Read ASEL.vi"("error in (no error)"=w637, "Instrument in"=w638) -> ("error out"=w642:errorcluster, "Opt_Selector.lvclass"=w628:refnum<class "Opt_Selector.lvclass">)  [unwired: 7 in, 1 out]
          n261 = call "Read GFOC.vi"("error in (no error)"=w637, "Instrument in"=w638) -> ("error out"=w639:errorcluster, "Opt_Continuous.lvclass"=w627:refnum<class "Opt_Continuous.lvclass">)  [unwired: 7 in, 1 out]
          n262 = call "Read WPROT.vi"("error in (no error)"=w637, "Instrument in"=w638) -> ("error out"=w652:errorcluster, "Opt_Selector.lvclass"=w651:refnum<class "Opt_Selector.lvclass">)  [unwired: 7 in, 1 out]
          n263 = call-dynamic "Read State Machine.vi"("error in (no error)"=w642, "Device in"=w628) -> ("error out"=w643:errorcluster, "State Machine.lvclass"=w644:refnum<class "State Machine.lvclass">)  [unwired: 7 in, 1 out]
          n264 = call-dynamic "Read State Machine.vi"("error in (no error)"=w639, "Device in"=w627) -> ("error out"=w640:errorcluster, "State Machine.lvclass"=w641:refnum<class "State Machine.lvclass">)  [unwired: 7 in, 1 out]
          n265 = call-dynamic "Read State Machine.vi"("error in (no error)"=w652, "Device in"=w651) -> ("error out"=w653:errorcluster, "State Machine.lvclass"=w654:refnum<class "State Machine.lvclass">)  [unwired: 7 in, 1 out]
          n266 = Increment(x=w648) -> (x+1=w647:u32)
          n267 = call-dynamic "Read State.vi"("error in (no error)"=w643, "State Machine in"=w644) -> ("error out"=w631:errorcluster, "State"=w635:i32)  [unwired: 7 in, 1 out]
          n268 = call-dynamic "Read State.vi"("error in (no error)"=w640, "State Machine in"=w641) -> ("error out"=w630:errorcluster, "State"=w634:i32)  [unwired: 7 in, 1 out]
          n269 = call-dynamic "Read State.vi"("error in (no error)"=w653, "State Machine in"=w654) -> ("error out"=w645:errorcluster, "State"=w636:i32)  [unwired: 7 in, 1 out]
          n270 = Compound Arithmetic op=ADD(w636, w635, w634) -> (w633:i32)
          n271 = Equal To 0?(x=w633) -> (x = 0?=w632:bool)
          n272 = Merge Errors(w645, w631, w630) -> (w629:errorcluster)
          n273 = Select(t=w647, s=w632, f=w648) -> (s? t:f=w649:u32)
          n274 = Bundle By Name(cluster=w646, "Obs_state"=w649) -> (w650:refnum<class "S4GUI.lvclass">)
        }
        frame 226 {
          # "Manda WPSEL para CLEAR, CALW para CLEAR e ASEL para CLEAR"
          n275 = call "Read Instrument.lvclass.vi"("error in (no error)"=w721, "S4ACS_GUI in"=w722) -> ("error out"=w705:errorcluster, "Instrument.lvclass"=w706:refnum<class "Instrument.lvclass">, "S4ACS_GUI out"=w723:refnum<class "S4GUI.lvclass">)  [unwired: 7 in]
          n276 = call "Read WPSEL.vi"("error in (no error)"=w705, "Instrument in"=w706) -> ("error out"=w701:errorcluster, "Opt_Selector.lvclass"=w700:refnum<class "Opt_Selector.lvclass">, "Instrument out"=w715:refnum<class "Instrument.lvclass">)  [unwired: 7 in]
          n277 = call "Write target.vi"("error in (no error)"=w701, "target"=80.0, "Optics in"=w700) -> ("error out"=w704:errorcluster, "Optics out"=w699:refnum<class "Opt_Selector.lvclass">)  [unwired: 7 in]
          n278 = call "Write target name.vi"("error in (no error)"=w704, "target name"="CLEAR", "Optics in"=w699) -> ("error out"=w697:errorcluster, "Optics out"=w698:refnum<class "Opt_Selector.lvclass">)  [unwired: 7 in]
          n279 = call-dynamic "Read State Machine.vi"("error in (no error)"=w697, "Device in"=w698) -> ("error out"=w710:errorcluster, "State Machine.lvclass"=w712:refnum<class "State Machine.lvclass">, "Device out"=w709:refnum<class "Opt_Selector.lvclass">)  [unwired: 7 in]
          n280 = call "Next State.vi"("error in (no error)"=w710, "New_State"=1, "State Machine in"=w712) -> ("error out"=w708:errorcluster, "State Machine out"=w707:refnum<class "State Machine.lvclass">)  [unwired: 7 in]
          n281 = call-dynamic "Write State Machine.vi"("error in (no error)"=w708, "State Machine.lvclass"=w707, "Device in"=w709) -> ("error out"=w714:errorcluster, "Device out"=w716:refnum<class "Opt_Selector.lvclass">)  [unwired: 7 in]
          n282 = Increment(x=w713) -> (x+1=w718:u32)
          n283 = call "Write WPSEL.vi"("error in (no error)"=w714, "Opt_Selector.lvclass"=w716, "Instrument in"=w715) -> ("error out"=w668:errorcluster, "Instrument out"=w667:refnum<class "Instrument.lvclass">)  [unwired: 7 in]
          n284 = call "Read CALW.vi"("error in (no error)"=w668, "Instrument in"=w667) -> ("error out"=w686:errorcluster, "Opt_Selector.lvclass"=w666:refnum<class "Opt_Selector.lvclass">, "Instrument out"=w664:refnum<class "Instrument.lvclass">)  [unwired: 7 in]
          n285 = call "Write target.vi"("error in (no error)"=w686, "target"=0.0, "Optics in"=w666) -> ("error out"=w689:errorcluster, "Optics out"=w685:refnum<class "Opt_Selector.lvclass">)  [unwired: 7 in]
          n286 = call "Write target name.vi"("error in (no error)"=w689, "target name"="CLEAR", "Optics in"=w685) -> ("error out"=w683:errorcluster, "Optics out"=w684:refnum<class "Opt_Selector.lvclass">)  [unwired: 7 in]
          n287 = call-dynamic "Read State Machine.vi"("error in (no error)"=w683, "Device in"=w684) -> ("error out"=w693:errorcluster, "State Machine.lvclass"=w695:refnum<class "State Machine.lvclass">, "Device out"=w692:refnum<class "Opt_Selector.lvclass">)  [unwired: 7 in]
          n288 = call "Next State.vi"("error in (no error)"=w693, "New_State"=1, "State Machine in"=w695) -> ("error out"=w691:errorcluster, "State Machine out"=w690:refnum<class "State Machine.lvclass">)  [unwired: 7 in]
          n289 = call-dynamic "Write State Machine.vi"("error in (no error)"=w691, "State Machine.lvclass"=w690, "Device in"=w692) -> ("error out"=w696:errorcluster, "Device out"=w665:refnum<class "Opt_Selector.lvclass">)  [unwired: 7 in]
          n290 = call "Write CALW.vi"("error in (no error)"=w696, "Opt_Selector.lvclass"=w665, "Instrument in"=w664) -> ("error out"=w663:errorcluster, "Instrument out"=w662:refnum<class "Instrument.lvclass">)  [unwired: 7 in]
          n291 = call "Read ASEL.vi"("error in (no error)"=w663, "Instrument in"=w662) -> ("error out"=w672:errorcluster, "Opt_Selector.lvclass"=w661:refnum<class "Opt_Selector.lvclass">, "Instrument out"=w659:refnum<class "Instrument.lvclass">)  [unwired: 7 in]
          n292 = call "Write target.vi"("error in (no error)"=w672, "target"=0.0, "Optics in"=w661) -> ("error out"=w675:errorcluster, "Optics out"=w671:refnum<class "Opt_Selector.lvclass">)  [unwired: 7 in]
          n293 = call "Write target name.vi"("error in (no error)"=w675, "target name"="CLEAR", "Optics in"=w671) -> ("error out"=w669:errorcluster, "Optics out"=w670:refnum<class "Opt_Selector.lvclass">)  [unwired: 7 in]
          n294 = call-dynamic "Read State Machine.vi"("error in (no error)"=w669, "Device in"=w670) -> ("error out"=w679:errorcluster, "State Machine.lvclass"=w681:refnum<class "State Machine.lvclass">, "Device out"=w678:refnum<class "Opt_Selector.lvclass">)  [unwired: 7 in]
          n295 = call "Next State.vi"("error in (no error)"=w679, "New_State"=1, "State Machine in"=w681) -> ("error out"=w677:errorcluster, "State Machine out"=w676:refnum<class "State Machine.lvclass">)  [unwired: 7 in]
          n296 = call-dynamic "Write State Machine.vi"("error in (no error)"=w677, "State Machine.lvclass"=w676, "Device in"=w678) -> ("error out"=w682:errorcluster, "Device out"=w660:refnum<class "Opt_Selector.lvclass">)  [unwired: 7 in]
          n297 = call "Write ASEL.vi"("error in (no error)"=w682, "Opt_Selector.lvclass"=w660, "Instrument in"=w659) -> ("error out"=w657:errorcluster, "Instrument out"=w658:refnum<class "Instrument.lvclass">)  [unwired: 7 in]
          n298 = call "Write Instrument.lvclass.vi"("error in (no error)"=w657, "Instrument.lvclass"=w658, "S4ACS_GUI in"=w723) -> ("error out"=w720:errorcluster, "S4ACS_GUI out"=w719:refnum<class "S4GUI.lvclass">)  [unwired: 7 in]
          n299 = Bundle By Name(cluster=w719, "Obs_state"=w718) -> (w717:refnum<class "S4GUI.lvclass">)
        }
        frame 227 {
          # "Espera terminar o movimento de WPSEL, ASEL e CALW para CLEAR."
          n300 = call "Read Instrument.lvclass.vi"("error in (no error)"=w752, "S4ACS_GUI in"=w753) -> ("error out"=w735:errorcluster, "Instrument.lvclass"=w736:refnum<class "Instrument.lvclass">, "S4ACS_GUI out"=w744:refnum<class "S4GUI.lvclass">)  [unwired: 7 in]
          n301 = call "Read ASEL.vi"("error in (no error)"=w735, "Instrument in"=w736) -> ("error out"=w740:errorcluster, "Opt_Selector.lvclass"=w726:refnum<class "Opt_Selector.lvclass">)  [unwired: 7 in, 1 out]
          n302 = call "Read CALW.vi"("error in (no error)"=w735, "Instrument in"=w736) -> ("error out"=w737:errorcluster, "Opt_Selector.lvclass"=w725:refnum<class "Opt_Selector.lvclass">)  [unwired: 7 in, 1 out]
          n303 = call "Read WPSEL.vi"("error in (no error)"=w735, "Instrument in"=w736) -> ("error out"=w749:errorcluster, "Opt_Selector.lvclass"=w748:refnum<class "Opt_Selector.lvclass">)  [unwired: 7 in, 1 out]
          n304 = call-dynamic "Read State Machine.vi"("error in (no error)"=w740, "Device in"=w726) -> ("error out"=w741:errorcluster, "State Machine.lvclass"=w742:refnum<class "State Machine.lvclass">)  [unwired: 7 in, 1 out]
          n305 = call-dynamic "Read State Machine.vi"("error in (no error)"=w737, "Device in"=w725) -> ("error out"=w738:errorcluster, "State Machine.lvclass"=w739:refnum<class "State Machine.lvclass">)  [unwired: 7 in, 1 out]
          n306 = call-dynamic "Read State Machine.vi"("error in (no error)"=w749, "Device in"=w748) -> ("error out"=w750:errorcluster, "State Machine.lvclass"=w751:refnum<class "State Machine.lvclass">)  [unwired: 7 in, 1 out]
          n307 = call-dynamic "Read State.vi"("error in (no error)"=w741, "State Machine in"=w742) -> ("error out"=w729:errorcluster, "State"=w733:i32)  [unwired: 7 in, 1 out]
          n308 = call-dynamic "Read State.vi"("error in (no error)"=w738, "State Machine in"=w739) -> ("error out"=w728:errorcluster, "State"=w732:i32)  [unwired: 7 in, 1 out]
          n309 = call-dynamic "Read State.vi"("error in (no error)"=w750, "State Machine in"=w751) -> ("error out"=w743:errorcluster, "State"=w734:i32)  [unwired: 7 in, 1 out]
          n310 = Compound Arithmetic op=ADD(w734, w733, w732) -> (w731:i32)
          n311 = Equal To 0?(x=w731) -> (x = 0?=w730:bool)
          n312 = Merge Errors(w743, w729, w728) -> (w727:errorcluster)
          n313 = Select(t=u32 0, s=w730, f=w745) -> (s? t:f=w746:u32)
          n314 = Bundle By Name(cluster=w744, "Obs_state"=w746) -> (w747:refnum<class "S4GUI.lvclass">)
        }
        frame 251 {
          n315 = call-dynamic "Read AcquisitionA.vi"("error in (no error)"=w764, "S4ACS_GUI in"=w765) -> ("error out"=w757:errorcluster, "Acquisition.lvclass"=w758:refnum<class "Acquisition.lvclass">, "S4ACS_GUI out"=w767:refnum<class "S4GUI.lvclass">)  [unwired: 7 in]
          n316 = call "Read connection.vi"("error in (no error)"=w757, "Server in"=w758) -> ("error out"=w756:errorcluster, "connection"=w754:bool, "Server out"=w755:refnum<class "Acquisition.lvclass">)  [unwired: 7 in]
          n317 = case shown="True" w754 {
            tunnel: w755 -> [w775 w795]
            tunnel: w756 -> [w774 w794]
            tunnel: [w775 w792] -> w768
            tunnel: [w774 w791] -> w766
            tunnel: w761 -> [w773 w784]
            tunnel: [w769 w783] -> w760
            frame False {
              n318 = Increment(x=w773) -> (x+1=w772:u32)
              n319 = Increment(x=w772) -> (x+1=w771:u32)
              n320 = Increment(x=w771) -> (x+1=w770:u32)
              n321 = Increment(x=w770) -> (x+1=w769:u32)
            }
            frame True {
              # "configura o canal,\nmas não dispara\na exposicao."
              n322 = call-dynamic "Read Channel.vi"("error in (no error)"=w794, "Acquisition in"=w795) -> ("error out"=w780:errorcluster, "Channel.lvclass"=w782:refnum<class "Channel.lvclass">, "Acquisition out"=w793:refnum<class "Acquisition.lvclass">)  [unwired: 7 in]
              n323 = call-dynamic "Write expose.vi"("error in (no error)"=w780, "expose"=FALSE, "Channel in"=w782) -> ("error out"=w779:errorcluster, "Channel out"=w781:refnum<class "Channel.lvclass">)  [unwired: 7 in]
              n324 = call-dynamic "Read State Machine.vi"("error in (no error)"=w779, "Device in"=w781) -> ("error out"=w788:errorcluster, "State Machine.lvclass"=w790:refnum<class "State Machine.lvclass">, "Device out"=w786:refnum<class "Channel.lvclass">)  [unwired: 7 in]
              n325 = call "Next State.vi"("error in (no error)"=w788, "New_State"=1, "State Machine in"=w790) -> ("error out"=w776:errorcluster, "State Machine out"=w777:refnum<class "State Machine.lvclass">)  [unwired: 7 in]
              n326 = Increment(x=w784) -> (x+1=w783:u32)
              n327 = call-dynamic "Write State Machine.vi"("error in (no error)"=w776, "State Machine.lvclass"=w777, "Device in"=w786) -> ("error out"=w785:errorcluster, "Device out"=w787:refnum<class "Channel.lvclass">)  [unwired: 7 in]
              n328 = call-dynamic "Write Channel.vi"("error in (no error)"=w785, "Channel.lvclass"=w787, "Acquisition in"=w793) -> ("error out"=w791:errorcluster, "Acquisition out"=w792:refnum<class "Acquisition.lvclass">)  [unwired: 7 in]
            }
          }
          n329 = call-dynamic "Write AcquisitionA.vi"("error in (no error)"=w766, "Acquisition.lvclass"=w768, "S4ACS_GUI in"=w767) -> ("error out"=w763:errorcluster, "S4ACS_GUI out"=w762:refnum<class "S4GUI.lvclass">)  [unwired: 7 in]
          n330 = Bundle By Name(cluster=w762, "Obs_state"=w760) -> (w759:refnum<class "S4GUI.lvclass">)
        }
        frame 252 {
          # "Espera terminar a execução do comando atual \nantes de ir ao proximo passo da Observação."
          n331 = call-dynamic "Read AcquisitionA.vi"("error in (no error)"=w813, "S4ACS_GUI in"=w814) -> ("error out"=w819:errorcluster, "Acquisition.lvclass"=w820:refnum<class "Acquisition.lvclass">, "S4ACS_GUI out"=w816:refnum<class "S4GUI.lvclass">)  [unwired: 7 in]
          n332 = call-dynamic "Read Channel.vi"("error in (no error)"=w819, "Acquisition in"=w820) -> ("error out"=w811:errorcluster, "Channel.lvclass"=w810:refnum<class "Channel.lvclass">, "Acquisition out"=w818:refnum<class "Acquisition.lvclass">)  [unwired: 7 in]
          n333 = call-dynamic "Read State Machine.vi"("error in (no error)"=w811, "Device in"=w810) -> ("error out"=w802:errorcluster, "State Machine.lvclass"=w804:refnum<class "State Machine.lvclass">, "Device out"=w808:refnum<class "Channel.lvclass">)  [unwired: 7 in]
          n334 = call-dynamic "Read State.vi"("error in (no error)"=w802, "State Machine in"=w804) -> ("error out"=w801:errorcluster, "State"=w798:i32, "State Machine out"=w803:refnum<class "State Machine.lvclass">)  [unwired: 7 in]
          n335 = Equal To 0?(x=w798) -> (x = 0?=w800:bool)
          n336 = call-dynamic "Write State Machine.vi"("error in (no error)"=w801, "State Machine.lvclass"=w803, "Device in"=w808) -> ("error out"=w807:errorcluster, "Device out"=w809:refnum<class "Channel.lvclass">)  [unwired: 7 in]
          n337 = call-dynamic "Write Channel.vi"("error in (no error)"=w807, "Channel.lvclass"=w809, "Acquisition in"=w818) -> ("error out"=w815:errorcluster, "Acquisition out"=w817:refnum<class "Acquisition.lvclass">)  [unwired: 7 in]
          n338 = disable-structure shown="Enabled" {
            disable-tunnel: [u32 299 ("t") w822] -> w797
            disable-tunnel: w796 -> [_ w823]
            frame Disabled {
            }
            frame Enabled {
              n339 = Increment(x=w823) -> (x+1=w822:u32)
            }
          }
          n340 = Select(t=w797, s=w800, f=w796) -> (s? t:f=w799:u32)
          n341 = call-dynamic "Write AcquisitionA.vi"("error in (no error)"=w815, "Acquisition.lvclass"=w817, "S4ACS_GUI in"=w816) -> ("error out"=w812:errorcluster, "S4ACS_GUI out"=w806:refnum<class "S4GUI.lvclass">)  [unwired: 7 in]
          n342 = Bundle By Name(cluster=w806, "Obs_state"=w799) -> (w805:refnum<class "S4GUI.lvclass">)
        }
        frame 253 {
          n343 = call-dynamic "Read Sync Box.lvclass.vi"("error in (no error)"=w828, "SPARC4_AC in"=w827) -> ("error out"=w831:errorcluster, "Sync Box.lvclass"=w832:refnum<class "Sync Box.lvclass">, "SPARC4_AC out"=w826:refnum<class "S4GUI.lvclass">)  [unwired: 7 in]
          n344 = call "Read connection.vi"("error in (no error)"=w831, "Server in"=w832) -> ("error out"=w830:errorcluster, "connection"=w829:bool)  [unwired: 7 in, 1 out]
          n345 = case shown="False" w829 {
            tunnel: w830 -> [w854 w878]
            tunnel: [w856 w878] -> w825
            tunnel: w835 -> [w866 w877]
            tunnel: [w865 w875] -> w834
            tunnel: w826 -> [w862 w874]
            tunnel: [w855 w874] -> w824
            frame False {
              # "Sem syncbox, \ntrigger mode = 0 (internal)"
              n346 = call-dynamic "Read AcquisitionA.vi"("error in (no error)"=w854, "S4ACS_GUI in"=w862) -> ("error out"=w860:errorcluster, "Acquisition.lvclass"=w861:refnum<class "Acquisition.lvclass">, "S4ACS_GUI out"=w859:refnum<class "S4GUI.lvclass">)  [unwired: 7 in]
              n347 = call-dynamic "Read Channel.vi"("error in (no error)"=w860, "Acquisition in"=w861) -> ("error out"=w840:errorcluster, "Channel.lvclass"=w839:refnum<class "Channel.lvclass">, "Acquisition out"=w873:refnum<class "Acquisition.lvclass">)  [unwired: 7 in]
              n348 = call-dynamic "Read Interface.vi"("error in (no error)"=w840, "Channel in"=w839) -> ("error out"=w838:errorcluster, "Interface.lvclass"=w844:refnum<class "Interface.lvclass">, "Channel out"=w843:refnum<class "Channel.lvclass">)  [unwired: 7 in]
              n349 = call-dynamic "Get CCD_Config.vi"("error in (no error)"=w838, "Interface in"=w844) -> ("error out"=w851:errorcluster, "output cluster"=w853:T1, "Interface out"=w850:refnum<class "Interface.lvclass">)  [unwired: 7 in]
              n350 = Bundle By Name(cluster=w853, "TRIGGER_MODE"=u8 0) -> (w849:T1)
              n351 = call-dynamic "Set CCD_Config.vi"("error in (no error)"=w851, "input cluster"=w849, "Interface in"=w850) -> ("error out"=w847:errorcluster, "Interface out"=w845:refnum<class "Interface.lvclass">)  [unwired: 7 in]
              n352 = Flatten To String(anything=w849, error in (no error)=w847) -> (data string=w848:string, error out=w846:errorcluster)  [unwired: 2 in, 1 out]
              n353 = call "Write flatted cluster.vi"("error in (no error)"=w846, "flatted cluster"=w848, "Interface in"=w845) -> ("error out"=w841:errorcluster, "Interface out"=w842:refnum<class "Interface.lvclass">)  [unwired: 7 in]
              n354 = call-dynamic "Write Interface.vi"("error in (no error)"=w841, "Interface.lvclass"=w842, "Channel in"=w843) -> ("error out"=w837:errorcluster, "Channel out"=w836:refnum<class "Channel.lvclass">)  [unwired: 7 in]
              n355 = call-dynamic "Read State Machine.vi"("error in (no error)"=w837, "Device in"=w836) -> ("error out"=w870:errorcluster, "State Machine.lvclass"=w872:refnum<class "State Machine.lvclass">, "Device out"=w868:refnum<class "Channel.lvclass">)  [unwired: 7 in]
              n356 = Increment(x=w866) -> (x+1=w865:u32)
              n357 = call "Next State.vi"("error in (no error)"=w870, "New_State"=60, "State Machine in"=w872) -> ("error out"=w863:errorcluster, "State Machine out"=w864:refnum<class "State Machine.lvclass">)  [unwired: 7 in]
              n358 = call-dynamic "Write State Machine.vi"("error in (no error)"=w863, "State Machine.lvclass"=w864, "Device in"=w868) -> ("error out"=w867:errorcluster, "Device out"=w869:refnum<class "Channel.lvclass">)  [unwired: 7 in]
              n359 = call-dynamic "Write Channel.vi"("error in (no error)"=w867, "Channel.lvclass"=w869, "Acquisition in"=w873) -> ("error out"=w857:errorcluster, "Acquisition out"=w858:refnum<class "Acquisition.lvclass">)  [unwired: 7 in]
              n360 = call-dynamic "Write AcquisitionA.vi"("error in (no error)"=w857, "Acquisition.lvclass"=w858, "S4ACS_GUI in"=w859) -> ("error out"=w856:errorcluster, "S4ACS_GUI out"=w855:refnum<class "S4GUI.lvclass">)  [unwired: 7 in]
            }
            frame True {
              n361 = Increment(x=w877) -> (x+1=w876:u32)
              n362 = Increment(x=w876) -> (x+1=w875:u32)
            }
          }
          n363 = Bundle By Name(cluster=w824, "Obs_state"=w834) -> (w833:refnum<class "S4GUI.lvclass">)
        }
        frame 254 {
          # "Espera terminar a execução do comando atual \nantes de ir ao proximo passo da Observação."
          n364 = call-dynamic "Read AcquisitionA.vi"("error in (no error)"=w896, "S4ACS_GUI in"=w897) -> ("error out"=w902:errorcluster, "Acquisition.lvclass"=w903:refnum<class "Acquisition.lvclass">, "S4ACS_GUI out"=w899:refnum<class "S4GUI.lvclass">)  [unwired: 7 in]
          n365 = call-dynamic "Read Channel.vi"("error in (no error)"=w902, "Acquisition in"=w903) -> ("error out"=w894:errorcluster, "Channel.lvclass"=w893:refnum<class "Channel.lvclass">, "Acquisition out"=w901:refnum<class "Acquisition.lvclass">)  [unwired: 7 in]
          n366 = call-dynamic "Read State Machine.vi"("error in (no error)"=w894, "Device in"=w893) -> ("error out"=w885:errorcluster, "State Machine.lvclass"=w887:refnum<class "State Machine.lvclass">, "Device out"=w891:refnum<class "Channel.lvclass">)  [unwired: 7 in]
          n367 = call-dynamic "Read State.vi"("error in (no error)"=w885, "State Machine in"=w887) -> ("error out"=w884:errorcluster, "State"=w881:i32, "State Machine out"=w886:refnum<class "State Machine.lvclass">)  [unwired: 7 in]
          n368 = Equal To 0?(x=w881) -> (x = 0?=w883:bool)
          n369 = call-dynamic "Write State Machine.vi"("error in (no error)"=w884, "State Machine.lvclass"=w886, "Device in"=w891) -> ("error out"=w890:errorcluster, "Device out"=w892:refnum<class "Channel.lvclass">)  [unwired: 7 in]
          n370 = call-dynamic "Write Channel.vi"("error in (no error)"=w890, "Channel.lvclass"=w892, "Acquisition in"=w901) -> ("error out"=w898:errorcluster, "Acquisition out"=w900:refnum<class "Acquisition.lvclass">)  [unwired: 7 in]
          n371 = disable-structure shown="Enabled" {
            disable-tunnel: [u32 299 ("t") w905] -> w880
            disable-tunnel: w879 -> [_ w906]
            frame Disabled {
            }
            frame Enabled {
              n372 = Increment(x=w906) -> (x+1=w905:u32)
            }
          }
          n373 = Select(t=w880, s=w883, f=w879) -> (s? t:f=w882:u32)
          n374 = call-dynamic "Write AcquisitionA.vi"("error in (no error)"=w898, "Acquisition.lvclass"=w900, "S4ACS_GUI in"=w899) -> ("error out"=w895:errorcluster, "S4ACS_GUI out"=w889:refnum<class "S4GUI.lvclass">)  [unwired: 7 in]
          n375 = Bundle By Name(cluster=w889, "Obs_state"=w882) -> (w888:refnum<class "S4GUI.lvclass">)
        }
        frame 255 {
          n376 = call "Read AcquisitionB.vi"("error in (no error)"=w917, "S4ACS_GUI in"=w918) -> ("error out"=w910:errorcluster, "Acquisition.lvclass"=w911:refnum<class "Acquisition.lvclass">, "S4ACS_GUI out"=w920:refnum<class "S4GUI.lvclass">)  [unwired: 7 in]
          n377 = call "Read connection.vi"("error in (no error)"=w910, "Server in"=w911) -> ("error out"=w909:errorcluster, "connection"=w907:bool, "Server out"=w908:refnum<class "Acquisition.lvclass">)  [unwired: 7 in]
          n378 = case shown="True" w907 {
            tunnel: w908 -> [w928 w948]
            tunnel: w909 -> [w927 w947]
            tunnel: [w928 w945] -> w921
            tunnel: [w927 w944] -> w919
            tunnel: w914 -> [w926 w937]
            tunnel: [w922 w936] -> w913
            frame False {
              n379 = Increment(x=w926) -> (x+1=w925:u32)
              n380 = Increment(x=w925) -> (x+1=w924:u32)
              n381 = Increment(x=w924) -> (x+1=w923:u32)
              n382 = Increment(x=w923) -> (x+1=w922:u32)
            }
            frame True {
              # "configura o canal,\nmas não dispara\na exposicao."
              n383 = call-dynamic "Read Channel.vi"("error in (no error)"=w947, "Acquisition in"=w948) -> ("error out"=w933:errorcluster, "Channel.lvclass"=w935:refnum<class "Channel.lvclass">, "Acquisition out"=w946:refnum<class "Acquisition.lvclass">)  [unwired: 7 in]
              n384 = call-dynamic "Write expose.vi"("error in (no error)"=w933, "expose"=FALSE, "Channel in"=w935) -> ("error out"=w932:errorcluster, "Channel out"=w934:refnum<class "Channel.lvclass">)  [unwired: 7 in]
              n385 = call-dynamic "Read State Machine.vi"("error in (no error)"=w932, "Device in"=w934) -> ("error out"=w941:errorcluster, "State Machine.lvclass"=w943:refnum<class "State Machine.lvclass">, "Device out"=w939:refnum<class "Channel.lvclass">)  [unwired: 7 in]
              n386 = call "Next State.vi"("error in (no error)"=w941, "New_State"=1, "State Machine in"=w943) -> ("error out"=w929:errorcluster, "State Machine out"=w930:refnum<class "State Machine.lvclass">)  [unwired: 7 in]
              n387 = Increment(x=w937) -> (x+1=w936:u32)
              n388 = call-dynamic "Write State Machine.vi"("error in (no error)"=w929, "State Machine.lvclass"=w930, "Device in"=w939) -> ("error out"=w938:errorcluster, "Device out"=w940:refnum<class "Channel.lvclass">)  [unwired: 7 in]
              n389 = call-dynamic "Write Channel.vi"("error in (no error)"=w938, "Channel.lvclass"=w940, "Acquisition in"=w946) -> ("error out"=w944:errorcluster, "Acquisition out"=w945:refnum<class "Acquisition.lvclass">)  [unwired: 7 in]
            }
          }
          n390 = call "Write AcquisitionB.vi"("error in (no error)"=w919, "Acquisition.lvclass"=w921, "S4ACS_GUI in"=w920) -> ("error out"=w916:errorcluster, "S4ACS_GUI out"=w915:refnum<class "S4GUI.lvclass">)  [unwired: 7 in]
          n391 = Bundle By Name(cluster=w915, "Obs_state"=w913) -> (w912:refnum<class "S4GUI.lvclass">)
        }
        frame 256 {
          # "Espera terminar a execução do comando atual \nantes de ir ao proximo passo da Observação."
          n392 = call "Read AcquisitionB.vi"("error in (no error)"=w966, "S4ACS_GUI in"=w967) -> ("error out"=w972:errorcluster, "Acquisition.lvclass"=w973:refnum<class "Acquisition.lvclass">, "S4ACS_GUI out"=w969:refnum<class "S4GUI.lvclass">)  [unwired: 7 in]
          n393 = call-dynamic "Read Channel.vi"("error in (no error)"=w972, "Acquisition in"=w973) -> ("error out"=w964:errorcluster, "Channel.lvclass"=w963:refnum<class "Channel.lvclass">, "Acquisition out"=w971:refnum<class "Acquisition.lvclass">)  [unwired: 7 in]
          n394 = call-dynamic "Read State Machine.vi"("error in (no error)"=w964, "Device in"=w963) -> ("error out"=w955:errorcluster, "State Machine.lvclass"=w957:refnum<class "State Machine.lvclass">, "Device out"=w961:refnum<class "Channel.lvclass">)  [unwired: 7 in]
          n395 = call-dynamic "Read State.vi"("error in (no error)"=w955, "State Machine in"=w957) -> ("error out"=w954:errorcluster, "State"=w951:i32, "State Machine out"=w956:refnum<class "State Machine.lvclass">)  [unwired: 7 in]
          n396 = call-dynamic "Write State Machine.vi"("error in (no error)"=w954, "State Machine.lvclass"=w956, "Device in"=w961) -> ("error out"=w960:errorcluster, "Device out"=w962:refnum<class "Channel.lvclass">)  [unwired: 7 in]
          n397 = call-dynamic "Write Channel.vi"("error in (no error)"=w960, "Channel.lvclass"=w962, "Acquisition in"=w971) -> ("error out"=w968:errorcluster, "Acquisition out"=w970:refnum<class "Acquisition.lvclass">)  [unwired: 7 in]
          n398 = Equal To 0?(x=w951) -> (x = 0?=w953:bool)
          n399 = Increment(x=w950) -> (x+1=w949:u32)
          n400 = Select(t=w949, s=w953, f=w950) -> (s? t:f=w952:u32)
          n401 = call "Write AcquisitionB.vi"("error in (no error)"=w968, "Acquisition.lvclass"=w970, "S4ACS_GUI in"=w969) -> ("error out"=w965:errorcluster, "S4ACS_GUI out"=w959:refnum<class "S4GUI.lvclass">)  [unwired: 7 in]
          n402 = Bundle By Name(cluster=w959, "Obs_state"=w952) -> (w958:refnum<class "S4GUI.lvclass">)
        }
        frame 257 {
          n403 = call-dynamic "Read Sync Box.lvclass.vi"("error in (no error)"=w978, "SPARC4_AC in"=w977) -> ("error out"=w981:errorcluster, "Sync Box.lvclass"=w982:refnum<class "Sync Box.lvclass">, "SPARC4_AC out"=w976:refnum<class "S4GUI.lvclass">)  [unwired: 7 in]
          n404 = call "Read connection.vi"("error in (no error)"=w981, "Server in"=w982) -> ("error out"=w980:errorcluster, "connection"=w979:bool)  [unwired: 7 in, 1 out]
          n405 = case shown="True" w979 {
            tunnel: w980 -> [w1004 w1028]
            tunnel: [w1006 w1028] -> w975
            tunnel: w985 -> [w1016 w1027]
            tunnel: [w1015 w1025] -> w984
            tunnel: w976 -> [w1012 w1024]
            tunnel: [w1005 w1024] -> w974
            frame False {
              # "Sem syncbox, \ntrigger mode = 0 (internal)"
              n406 = call "Read AcquisitionB.vi"("error in (no error)"=w1004, "S4ACS_GUI in"=w1012) -> ("error out"=w1010:errorcluster, "Acquisition.lvclass"=w1011:refnum<class "Acquisition.lvclass">, "S4ACS_GUI out"=w1009:refnum<class "S4GUI.lvclass">)  [unwired: 7 in]
              n407 = call-dynamic "Read Channel.vi"("error in (no error)"=w1010, "Acquisition in"=w1011) -> ("error out"=w990:errorcluster, "Channel.lvclass"=w989:refnum<class "Channel.lvclass">, "Acquisition out"=w1023:refnum<class "Acquisition.lvclass">)  [unwired: 7 in]
              n408 = call-dynamic "Read Interface.vi"("error in (no error)"=w990, "Channel in"=w989) -> ("error out"=w988:errorcluster, "Interface.lvclass"=w994:refnum<class "Interface.lvclass">, "Channel out"=w993:refnum<class "Channel.lvclass">)  [unwired: 7 in]
              n409 = call-dynamic "Get CCD_Config.vi"("error in (no error)"=w988, "Interface in"=w994) -> ("error out"=w1001:errorcluster, "output cluster"=w1003:T1, "Interface out"=w1000:refnum<class "Interface.lvclass">)  [unwired: 7 in]
              n410 = Bundle By Name(cluster=w1003, "TRIGGER_MODE"=u8 0) -> (w999:T1)
              n411 = call-dynamic "Set CCD_Config.vi"("error in (no error)"=w1001, "input cluster"=w999, "Interface in"=w1000) -> ("error out"=w997:errorcluster, "Interface out"=w995:refnum<class "Interface.lvclass">)  [unwired: 7 in]
              n412 = Flatten To String(anything=w999, error in (no error)=w997) -> (data string=w998:string, error out=w996:errorcluster)  [unwired: 2 in, 1 out]
              n413 = call "Write flatted cluster.vi"("error in (no error)"=w996, "flatted cluster"=w998, "Interface in"=w995) -> ("error out"=w991:errorcluster, "Interface out"=w992:refnum<class "Interface.lvclass">)  [unwired: 7 in]
              n414 = call-dynamic "Write Interface.vi"("error in (no error)"=w991, "Interface.lvclass"=w992, "Channel in"=w993) -> ("error out"=w987:errorcluster, "Channel out"=w986:refnum<class "Channel.lvclass">)  [unwired: 7 in]
              n415 = call-dynamic "Read State Machine.vi"("error in (no error)"=w987, "Device in"=w986) -> ("error out"=w1020:errorcluster, "State Machine.lvclass"=w1022:refnum<class "State Machine.lvclass">, "Device out"=w1018:refnum<class "Channel.lvclass">)  [unwired: 7 in]
              n416 = Increment(x=w1016) -> (x+1=w1015:u32)
              n417 = call "Next State.vi"("error in (no error)"=w1020, "New_State"=60, "State Machine in"=w1022) -> ("error out"=w1013:errorcluster, "State Machine out"=w1014:refnum<class "State Machine.lvclass">)  [unwired: 7 in]
              n418 = call-dynamic "Write State Machine.vi"("error in (no error)"=w1013, "State Machine.lvclass"=w1014, "Device in"=w1018) -> ("error out"=w1017:errorcluster, "Device out"=w1019:refnum<class "Channel.lvclass">)  [unwired: 7 in]
              n419 = call-dynamic "Write Channel.vi"("error in (no error)"=w1017, "Channel.lvclass"=w1019, "Acquisition in"=w1023) -> ("error out"=w1007:errorcluster, "Acquisition out"=w1008:refnum<class "Acquisition.lvclass">)  [unwired: 7 in]
              n420 = call "Write AcquisitionB.vi"("error in (no error)"=w1007, "Acquisition.lvclass"=w1008, "S4ACS_GUI in"=w1009) -> ("error out"=w1006:errorcluster, "S4ACS_GUI out"=w1005:refnum<class "S4GUI.lvclass">)  [unwired: 7 in]
            }
            frame True {
              n421 = Increment(x=w1027) -> (x+1=w1026:u32)
              n422 = Increment(x=w1026) -> (x+1=w1025:u32)
            }
          }
          n423 = Bundle By Name(cluster=w974, "Obs_state"=w984) -> (w983:refnum<class "S4GUI.lvclass">)
        }
        frame 258 {
          # "Espera terminar a execução do comando atual \nantes de ir ao proximo passo da Observação."
          n424 = call "Read AcquisitionB.vi"("error in (no error)"=w1046, "S4ACS_GUI in"=w1047) -> ("error out"=w1052:errorcluster, "Acquisition.lvclass"=w1053:refnum<class "Acquisition.lvclass">, "S4ACS_GUI out"=w1049:refnum<class "S4GUI.lvclass">)  [unwired: 7 in]
          n425 = call-dynamic "Read Channel.vi"("error in (no error)"=w1052, "Acquisition in"=w1053) -> ("error out"=w1044:errorcluster, "Channel.lvclass"=w1043:refnum<class "Channel.lvclass">, "Acquisition out"=w1051:refnum<class "Acquisition.lvclass">)  [unwired: 7 in]
          n426 = call-dynamic "Read State Machine.vi"("error in (no error)"=w1044, "Device in"=w1043) -> ("error out"=w1035:errorcluster, "State Machine.lvclass"=w1037:refnum<class "State Machine.lvclass">, "Device out"=w1041:refnum<class "Channel.lvclass">)  [unwired: 7 in]
          n427 = call-dynamic "Read State.vi"("error in (no error)"=w1035, "State Machine in"=w1037) -> ("error out"=w1034:errorcluster, "State"=w1031:i32, "State Machine out"=w1036:refnum<class "State Machine.lvclass">)  [unwired: 7 in]
          n428 = call-dynamic "Write State Machine.vi"("error in (no error)"=w1034, "State Machine.lvclass"=w1036, "Device in"=w1041) -> ("error out"=w1040:errorcluster, "Device out"=w1042:refnum<class "Channel.lvclass">)  [unwired: 7 in]
          n429 = call-dynamic "Write Channel.vi"("error in (no error)"=w1040, "Channel.lvclass"=w1042, "Acquisition in"=w1051) -> ("error out"=w1048:errorcluster, "Acquisition out"=w1050:refnum<class "Acquisition.lvclass">)  [unwired: 7 in]
          n430 = Equal To 0?(x=w1031) -> (x = 0?=w1033:bool)
          n431 = Increment(x=w1030) -> (x+1=w1029:u32)
          n432 = Select(t=w1029, s=w1033, f=w1030) -> (s? t:f=w1032:u32)
          n433 = call "Write AcquisitionB.vi"("error in (no error)"=w1048, "Acquisition.lvclass"=w1050, "S4ACS_GUI in"=w1049) -> ("error out"=w1045:errorcluster, "S4ACS_GUI out"=w1039:refnum<class "S4GUI.lvclass">)  [unwired: 7 in]
          n434 = Bundle By Name(cluster=w1039, "Obs_state"=w1032) -> (w1038:refnum<class "S4GUI.lvclass">)
        }
        frame 259 {
          n435 = call-dynamic "Read AcquisitionC.vi"("error in (no error)"=w1064, "S4ACS_GUI in"=w1065) -> ("error out"=w1056:errorcluster, "Acquisition.lvclass"=w1058:refnum<class "Acquisition.lvclass">, "S4ACS_GUI out"=w1067:refnum<class "S4GUI.lvclass">)  [unwired: 7 in]
          n436 = call "Read connection.vi"("error in (no error)"=w1056, "Server in"=w1058) -> ("error out"=w1055:errorcluster, "connection"=w1054:bool, "Server out"=w1057:refnum<class "Acquisition.lvclass">)  [unwired: 7 in]
          n437 = case shown="True" w1054 {
            tunnel: w1057 -> [w1074 w1095]
            tunnel: w1055 -> [w1075 w1094]
            tunnel: [w1074 w1092] -> w1068
            tunnel: [w1075 w1091] -> w1066
            tunnel: w1061 -> [w1073 w1084]
            tunnel: [w1069 w1083] -> w1060
            frame False {
              n438 = Increment(x=w1073) -> (x+1=w1072:u32)
              n439 = Increment(x=w1072) -> (x+1=w1071:u32)
              n440 = Increment(x=w1071) -> (x+1=w1070:u32)
              n441 = Increment(x=w1070) -> (x+1=w1069:u32)
            }
            frame True {
              # "configura o canal,\nmas não dispara\na exposicao."
              n442 = call-dynamic "Read Channel.vi"("error in (no error)"=w1094, "Acquisition in"=w1095) -> ("error out"=w1080:errorcluster, "Channel.lvclass"=w1082:refnum<class "Channel.lvclass">, "Acquisition out"=w1093:refnum<class "Acquisition.lvclass">)  [unwired: 7 in]
              n443 = call-dynamic "Write expose.vi"("error in (no error)"=w1080, "expose"=FALSE, "Channel in"=w1082) -> ("error out"=w1079:errorcluster, "Channel out"=w1081:refnum<class "Channel.lvclass">)  [unwired: 7 in]
              n444 = call-dynamic "Read State Machine.vi"("error in (no error)"=w1079, "Device in"=w1081) -> ("error out"=w1088:errorcluster, "State Machine.lvclass"=w1090:refnum<class "State Machine.lvclass">, "Device out"=w1086:refnum<class "Channel.lvclass">)  [unwired: 7 in]
              n445 = call "Next State.vi"("error in (no error)"=w1088, "New_State"=1, "State Machine in"=w1090) -> ("error out"=w1076:errorcluster, "State Machine out"=w1077:refnum<class "State Machine.lvclass">)  [unwired: 7 in]
              n446 = Increment(x=w1084) -> (x+1=w1083:u32)
              n447 = call-dynamic "Write State Machine.vi"("error in (no error)"=w1076, "State Machine.lvclass"=w1077, "Device in"=w1086) -> ("error out"=w1085:errorcluster, "Device out"=w1087:refnum<class "Channel.lvclass">)  [unwired: 7 in]
              n448 = call-dynamic "Write Channel.vi"("error in (no error)"=w1085, "Channel.lvclass"=w1087, "Acquisition in"=w1093) -> ("error out"=w1091:errorcluster, "Acquisition out"=w1092:refnum<class "Acquisition.lvclass">)  [unwired: 7 in]
            }
          }
          n449 = call-dynamic "Write AcquisitionC.vi"("error in (no error)"=w1066, "Acquisition.lvclass"=w1068, "S4ACS_GUI in"=w1067) -> ("error out"=w1063:errorcluster, "S4ACS_GUI out"=w1062:refnum<class "S4GUI.lvclass">)  [unwired: 7 in]
          n450 = Bundle By Name(cluster=w1062, "Obs_state"=w1060) -> (w1059:refnum<class "S4GUI.lvclass">)
        }
        frame 260 {
          # "Espera terminar a execução do comando atual \nantes de ir ao proximo passo da Observação."
          n451 = call-dynamic "Read AcquisitionC.vi"("error in (no error)"=w1113, "S4ACS_GUI in"=w1114) -> ("error out"=w1119:errorcluster, "Acquisition.lvclass"=w1120:refnum<class "Acquisition.lvclass">, "S4ACS_GUI out"=w1116:refnum<class "S4GUI.lvclass">)  [unwired: 7 in]
          n452 = call-dynamic "Read Channel.vi"("error in (no error)"=w1119, "Acquisition in"=w1120) -> ("error out"=w1111:errorcluster, "Channel.lvclass"=w1110:refnum<class "Channel.lvclass">, "Acquisition out"=w1118:refnum<class "Acquisition.lvclass">)  [unwired: 7 in]
          n453 = call-dynamic "Read State Machine.vi"("error in (no error)"=w1111, "Device in"=w1110) -> ("error out"=w1102:errorcluster, "State Machine.lvclass"=w1104:refnum<class "State Machine.lvclass">, "Device out"=w1108:refnum<class "Channel.lvclass">)  [unwired: 7 in]
          n454 = call-dynamic "Read State.vi"("error in (no error)"=w1102, "State Machine in"=w1104) -> ("error out"=w1101:errorcluster, "State"=w1098:i32, "State Machine out"=w1103:refnum<class "State Machine.lvclass">)  [unwired: 7 in]
          n455 = Equal To 0?(x=w1098) -> (x = 0?=w1100:bool)
          n456 = call-dynamic "Write State Machine.vi"("error in (no error)"=w1101, "State Machine.lvclass"=w1103, "Device in"=w1108) -> ("error out"=w1107:errorcluster, "Device out"=w1109:refnum<class "Channel.lvclass">)  [unwired: 7 in]
          n457 = call-dynamic "Write Channel.vi"("error in (no error)"=w1107, "Channel.lvclass"=w1109, "Acquisition in"=w1118) -> ("error out"=w1115:errorcluster, "Acquisition out"=w1117:refnum<class "Acquisition.lvclass">)  [unwired: 7 in]
          n458 = Increment(x=w1097) -> (x+1=w1096:u32)
          n459 = Select(t=w1096, s=w1100, f=w1097) -> (s? t:f=w1099:u32)
          n460 = call-dynamic "Write AcquisitionC.vi"("error in (no error)"=w1115, "Acquisition.lvclass"=w1117, "S4ACS_GUI in"=w1116) -> ("error out"=w1112:errorcluster, "S4ACS_GUI out"=w1106:refnum<class "S4GUI.lvclass">)  [unwired: 7 in]
          n461 = Bundle By Name(cluster=w1106, "Obs_state"=w1099) -> (w1105:refnum<class "S4GUI.lvclass">)
        }
        frame 261 {
          n462 = call-dynamic "Read Sync Box.lvclass.vi"("error in (no error)"=w1125, "SPARC4_AC in"=w1124) -> ("error out"=w1128:errorcluster, "Sync Box.lvclass"=w1129:refnum<class "Sync Box.lvclass">, "SPARC4_AC out"=w1123:refnum<class "S4GUI.lvclass">)  [unwired: 7 in]
          n463 = call "Read connection.vi"("error in (no error)"=w1128, "Server in"=w1129) -> ("error out"=w1127:errorcluster, "connection"=w1126:bool)  [unwired: 7 in, 1 out]
          n464 = case shown="True" w1126 {
            tunnel: w1127 -> [w1151 w1175]
            tunnel: [w1153 w1175] -> w1122
            tunnel: w1132 -> [w1163 w1174]
            tunnel: [w1162 w1172] -> w1131
            tunnel: w1123 -> [w1159 w1171]
            tunnel: [w1152 w1171] -> w1121
            frame False {
              # "Sem syncbox, \ntrigger mode = 0 (internal)"
              n465 = call-dynamic "Read AcquisitionC.vi"("error in (no error)"=w1151, "S4ACS_GUI in"=w1159) -> ("error out"=w1157:errorcluster, "Acquisition.lvclass"=w1158:refnum<class "Acquisition.lvclass">, "S4ACS_GUI out"=w1156:refnum<class "S4GUI.lvclass">)  [unwired: 7 in]
              n466 = call-dynamic "Read Channel.vi"("error in (no error)"=w1157, "Acquisition in"=w1158) -> ("error out"=w1137:errorcluster, "Channel.lvclass"=w1136:refnum<class "Channel.lvclass">, "Acquisition out"=w1170:refnum<class "Acquisition.lvclass">)  [unwired: 7 in]
              n467 = call-dynamic "Read Interface.vi"("error in (no error)"=w1137, "Channel in"=w1136) -> ("error out"=w1135:errorcluster, "Interface.lvclass"=w1141:refnum<class "Interface.lvclass">, "Channel out"=w1140:refnum<class "Channel.lvclass">)  [unwired: 7 in]
              n468 = call-dynamic "Get CCD_Config.vi"("error in (no error)"=w1135, "Interface in"=w1141) -> ("error out"=w1148:errorcluster, "output cluster"=w1150:T1, "Interface out"=w1147:refnum<class "Interface.lvclass">)  [unwired: 7 in]
              n469 = Bundle By Name(cluster=w1150, "TRIGGER_MODE"=u8 0) -> (w1146:T1)
              n470 = call-dynamic "Set CCD_Config.vi"("error in (no error)"=w1148, "input cluster"=w1146, "Interface in"=w1147) -> ("error out"=w1144:errorcluster, "Interface out"=w1142:refnum<class "Interface.lvclass">)  [unwired: 7 in]
              n471 = Flatten To String(anything=w1146, error in (no error)=w1144) -> (data string=w1145:string, error out=w1143:errorcluster)  [unwired: 2 in, 1 out]
              n472 = call "Write flatted cluster.vi"("error in (no error)"=w1143, "flatted cluster"=w1145, "Interface in"=w1142) -> ("error out"=w1138:errorcluster, "Interface out"=w1139:refnum<class "Interface.lvclass">)  [unwired: 7 in]
              n473 = call-dynamic "Write Interface.vi"("error in (no error)"=w1138, "Interface.lvclass"=w1139, "Channel in"=w1140) -> ("error out"=w1134:errorcluster, "Channel out"=w1133:refnum<class "Channel.lvclass">)  [unwired: 7 in]
              n474 = call-dynamic "Read State Machine.vi"("error in (no error)"=w1134, "Device in"=w1133) -> ("error out"=w1167:errorcluster, "State Machine.lvclass"=w1169:refnum<class "State Machine.lvclass">, "Device out"=w1165:refnum<class "Channel.lvclass">)  [unwired: 7 in]
              n475 = Increment(x=w1163) -> (x+1=w1162:u32)
              n476 = call "Next State.vi"("error in (no error)"=w1167, "New_State"=60, "State Machine in"=w1169) -> ("error out"=w1160:errorcluster, "State Machine out"=w1161:refnum<class "State Machine.lvclass">)  [unwired: 7 in]
              n477 = call-dynamic "Write State Machine.vi"("error in (no error)"=w1160, "State Machine.lvclass"=w1161, "Device in"=w1165) -> ("error out"=w1164:errorcluster, "Device out"=w1166:refnum<class "Channel.lvclass">)  [unwired: 7 in]
              n478 = call-dynamic "Write Channel.vi"("error in (no error)"=w1164, "Channel.lvclass"=w1166, "Acquisition in"=w1170) -> ("error out"=w1154:errorcluster, "Acquisition out"=w1155:refnum<class "Acquisition.lvclass">)  [unwired: 7 in]
              n479 = call-dynamic "Write AcquisitionC.vi"("error in (no error)"=w1154, "Acquisition.lvclass"=w1155, "S4ACS_GUI in"=w1156) -> ("error out"=w1153:errorcluster, "S4ACS_GUI out"=w1152:refnum<class "S4GUI.lvclass">)  [unwired: 7 in]
            }
            frame True {
              n480 = Increment(x=w1174) -> (x+1=w1173:u32)
              n481 = Increment(x=w1173) -> (x+1=w1172:u32)
            }
          }
          n482 = Bundle By Name(cluster=w1121, "Obs_state"=w1131) -> (w1130:refnum<class "S4GUI.lvclass">)
        }
        frame 262 {
          # "Espera terminar a execução do comando atual \nantes de ir ao proximo passo da Observação."
          n483 = call-dynamic "Read AcquisitionC.vi"("error in (no error)"=w1193, "S4ACS_GUI in"=w1194) -> ("error out"=w1199:errorcluster, "Acquisition.lvclass"=w1200:refnum<class "Acquisition.lvclass">, "S4ACS_GUI out"=w1196:refnum<class "S4GUI.lvclass">)  [unwired: 7 in]
          n484 = call-dynamic "Read Channel.vi"("error in (no error)"=w1199, "Acquisition in"=w1200) -> ("error out"=w1191:errorcluster, "Channel.lvclass"=w1190:refnum<class "Channel.lvclass">, "Acquisition out"=w1198:refnum<class "Acquisition.lvclass">)  [unwired: 7 in]
          n485 = call-dynamic "Read State Machine.vi"("error in (no error)"=w1191, "Device in"=w1190) -> ("error out"=w1182:errorcluster, "State Machine.lvclass"=w1184:refnum<class "State Machine.lvclass">, "Device out"=w1188:refnum<class "Channel.lvclass">)  [unwired: 7 in]
          n486 = call-dynamic "Read State.vi"("error in (no error)"=w1182, "State Machine in"=w1184) -> ("error out"=w1181:errorcluster, "State"=w1178:i32, "State Machine out"=w1183:refnum<class "State Machine.lvclass">)  [unwired: 7 in]
          n487 = Equal To 0?(x=w1178) -> (x = 0?=w1180:bool)
          n488 = call-dynamic "Write State Machine.vi"("error in (no error)"=w1181, "State Machine.lvclass"=w1183, "Device in"=w1188) -> ("error out"=w1187:errorcluster, "Device out"=w1189:refnum<class "Channel.lvclass">)  [unwired: 7 in]
          n489 = call-dynamic "Write Channel.vi"("error in (no error)"=w1187, "Channel.lvclass"=w1189, "Acquisition in"=w1198) -> ("error out"=w1195:errorcluster, "Acquisition out"=w1197:refnum<class "Acquisition.lvclass">)  [unwired: 7 in]
          n490 = Increment(x=w1177) -> (x+1=w1176:u32)
          n491 = Select(t=w1176, s=w1180, f=w1177) -> (s? t:f=w1179:u32)
          n492 = call-dynamic "Write AcquisitionC.vi"("error in (no error)"=w1195, "Acquisition.lvclass"=w1197, "S4ACS_GUI in"=w1196) -> ("error out"=w1192:errorcluster, "S4ACS_GUI out"=w1186:refnum<class "S4GUI.lvclass">)  [unwired: 7 in]
          n493 = Bundle By Name(cluster=w1186, "Obs_state"=w1179) -> (w1185:refnum<class "S4GUI.lvclass">)
        }
        frame 263 {
          # "Dispara o comando para o dispositivo corrente."
          n494 = call-dynamic "Read AcquisitionD.vi"("error in (no error)"=w1211, "S4ACS_GUI in"=w1212) -> ("error out"=w1204:errorcluster, "Acquisition.lvclass"=w1205:refnum<class "Acquisition.lvclass">, "S4ACS_GUI out"=w1214:refnum<class "S4GUI.lvclass">)  [unwired: 7 in]
          n495 = call "Read connection.vi"("error in (no error)"=w1204, "Server in"=w1205) -> ("error out"=w1202:errorcluster, "connection"=w1201:bool, "Server out"=w1203:refnum<class "Acquisition.lvclass">)  [unwired: 7 in]
          n496 = case shown="False" w1201 {
            tunnel: w1203 -> [w1218 w1238]
            tunnel: w1202 -> [w1217 w1237]
            tunnel: [w1218 w1235] -> w1215
            tunnel: [w1217 w1234] -> w1213
            tunnel: w1208 -> [_ w1227]
            tunnel: [u32 299 w1226] -> w1207
            frame False {
            }
            frame True {
              # "configura o canal,\nmas não dispara\na exposicao."
              n497 = call-dynamic "Read Channel.vi"("error in (no error)"=w1237, "Acquisition in"=w1238) -> ("error out"=w1223:errorcluster, "Channel.lvclass"=w1225:refnum<class "Channel.lvclass">, "Acquisition out"=w1236:refnum<class "Acquisition.lvclass">)  [unwired: 7 in]
              n498 = call-dynamic "Write expose.vi"("error in (no error)"=w1223, "expose"=FALSE, "Channel in"=w1225) -> ("error out"=w1222:errorcluster, "Channel out"=w1224:refnum<class "Channel.lvclass">)  [unwired: 7 in]
              n499 = call-dynamic "Read State Machine.vi"("error in (no error)"=w1222, "Device in"=w1224) -> ("error out"=w1231:errorcluster, "State Machine.lvclass"=w1233:refnum<class "State Machine.lvclass">, "Device out"=w1229:refnum<class "Channel.lvclass">)  [unwired: 7 in]
              n500 = call "Next State.vi"("error in (no error)"=w1231, "New_State"=1, "State Machine in"=w1233) -> ("error out"=w1219:errorcluster, "State Machine out"=w1220:refnum<class "State Machine.lvclass">)  [unwired: 7 in]
              n501 = Increment(x=w1227) -> (x+1=w1226:u32)
              n502 = call-dynamic "Write State Machine.vi"("error in (no error)"=w1219, "State Machine.lvclass"=w1220, "Device in"=w1229) -> ("error out"=w1228:errorcluster, "Device out"=w1230:refnum<class "Channel.lvclass">)  [unwired: 7 in]
              n503 = call-dynamic "Write Channel.vi"("error in (no error)"=w1228, "Channel.lvclass"=w1230, "Acquisition in"=w1236) -> ("error out"=w1234:errorcluster, "Acquisition out"=w1235:refnum<class "Acquisition.lvclass">)  [unwired: 7 in]
            }
          }
          n504 = call-dynamic "Write AcquisitionD.vi"("error in (no error)"=w1213, "Acquisition.lvclass"=w1215, "S4ACS_GUI in"=w1214) -> ("error out"=w1210:errorcluster, "S4ACS_GUI out"=w1209:refnum<class "S4GUI.lvclass">)  [unwired: 7 in]
          n505 = Bundle By Name(cluster=w1209, "Obs_state"=w1207) -> (w1206:refnum<class "S4GUI.lvclass">)
        }
        frame 264 {
          # "Espera terminar a execução do comando atual \nantes de ir ao proximo passo da Observação."
          n506 = call-dynamic "Read AcquisitionD.vi"("error in (no error)"=w1256, "S4ACS_GUI in"=w1257) -> ("error out"=w1262:errorcluster, "Acquisition.lvclass"=w1263:refnum<class "Acquisition.lvclass">, "S4ACS_GUI out"=w1259:refnum<class "S4GUI.lvclass">)  [unwired: 7 in]
          n507 = call-dynamic "Read Channel.vi"("error in (no error)"=w1262, "Acquisition in"=w1263) -> ("error out"=w1254:errorcluster, "Channel.lvclass"=w1253:refnum<class "Channel.lvclass">, "Acquisition out"=w1261:refnum<class "Acquisition.lvclass">)  [unwired: 7 in]
          n508 = call-dynamic "Read State Machine.vi"("error in (no error)"=w1254, "Device in"=w1253) -> ("error out"=w1245:errorcluster, "State Machine.lvclass"=w1247:refnum<class "State Machine.lvclass">, "Device out"=w1251:refnum<class "Channel.lvclass">)  [unwired: 7 in]
          n509 = call-dynamic "Read State.vi"("error in (no error)"=w1245, "State Machine in"=w1247) -> ("error out"=w1244:errorcluster, "State"=w1241:i32, "State Machine out"=w1246:refnum<class "State Machine.lvclass">)  [unwired: 7 in]
          n510 = Equal To 0?(x=w1241) -> (x = 0?=w1243:bool)
          n511 = call-dynamic "Write State Machine.vi"("error in (no error)"=w1244, "State Machine.lvclass"=w1246, "Device in"=w1251) -> ("error out"=w1250:errorcluster, "Device out"=w1252:refnum<class "Channel.lvclass">)  [unwired: 7 in]
          n512 = call-dynamic "Write Channel.vi"("error in (no error)"=w1250, "Channel.lvclass"=w1252, "Acquisition in"=w1261) -> ("error out"=w1258:errorcluster, "Acquisition out"=w1260:refnum<class "Acquisition.lvclass">)  [unwired: 7 in]
          n513 = Increment(x=w1240) -> (x+1=w1239:u32)
          n514 = Select(t=w1239, s=w1243, f=w1240) -> (s? t:f=w1242:u32)
          n515 = call-dynamic "Write AcquisitionD.vi"("error in (no error)"=w1258, "Acquisition.lvclass"=w1260, "S4ACS_GUI in"=w1259) -> ("error out"=w1255:errorcluster, "S4ACS_GUI out"=w1249:refnum<class "S4GUI.lvclass">)  [unwired: 7 in]
          n516 = Bundle By Name(cluster=w1249, "Obs_state"=w1242) -> (w1248:refnum<class "S4GUI.lvclass">)
        }
        frame 265 {
          n517 = call-dynamic "Read Sync Box.lvclass.vi"("error in (no error)"=w1268, "SPARC4_AC in"=w1267) -> ("error out"=w1271:errorcluster, "Sync Box.lvclass"=w1272:refnum<class "Sync Box.lvclass">, "SPARC4_AC out"=w1266:refnum<class "S4GUI.lvclass">)  [unwired: 7 in]
          n518 = call "Read connection.vi"("error in (no error)"=w1271, "Server in"=w1272) -> ("error out"=w1270:errorcluster, "connection"=w1269:bool)  [unwired: 7 in, 1 out]
          n519 = case shown="False" w1269 {
            tunnel: w1270 -> [w1294 w1316]
            tunnel: [w1296 w1316] -> w1265
            tunnel: w1275 -> [w1306 _]
            tunnel: [w1305 u32 299] -> w1274
            tunnel: w1266 -> [w1302 w1315]
            tunnel: [w1295 w1315] -> w1264
            frame False {
              # "Sem syncbox, \ntrigger mode = 0 (internal)"
              n520 = call-dynamic "Read AcquisitionD.vi"("error in (no error)"=w1294, "S4ACS_GUI in"=w1302) -> ("error out"=w1300:errorcluster, "Acquisition.lvclass"=w1301:refnum<class "Acquisition.lvclass">, "S4ACS_GUI out"=w1299:refnum<class "S4GUI.lvclass">)  [unwired: 7 in]
              n521 = call-dynamic "Read Channel.vi"("error in (no error)"=w1300, "Acquisition in"=w1301) -> ("error out"=w1280:errorcluster, "Channel.lvclass"=w1279:refnum<class "Channel.lvclass">, "Acquisition out"=w1313:refnum<class "Acquisition.lvclass">)  [unwired: 7 in]
              n522 = call-dynamic "Read Interface.vi"("error in (no error)"=w1280, "Channel in"=w1279) -> ("error out"=w1278:errorcluster, "Interface.lvclass"=w1284:refnum<class "Interface.lvclass">, "Channel out"=w1283:refnum<class "Channel.lvclass">)  [unwired: 7 in]
              n523 = call-dynamic "Get CCD_Config.vi"("error in (no error)"=w1278, "Interface in"=w1284) -> ("error out"=w1291:errorcluster, "output cluster"=w1293:T1, "Interface out"=w1290:refnum<class "Interface.lvclass">)  [unwired: 7 in]
              n524 = Bundle By Name(cluster=w1293, "TRIGGER_MODE"=u8 0) -> (w1289:T1)
              n525 = call-dynamic "Set CCD_Config.vi"("error in (no error)"=w1291, "input cluster"=w1289, "Interface in"=w1290) -> ("error out"=w1287:errorcluster, "Interface out"=w1285:refnum<class "Interface.lvclass">)  [unwired: 7 in]
              n526 = Flatten To String(anything=w1289, error in (no error)=w1287) -> (data string=w1288:string, error out=w1286:errorcluster)  [unwired: 2 in, 1 out]
              n527 = call "Write flatted cluster.vi"("error in (no error)"=w1286, "flatted cluster"=w1288, "Interface in"=w1285) -> ("error out"=w1281:errorcluster, "Interface out"=w1282:refnum<class "Interface.lvclass">)  [unwired: 7 in]
              n528 = call-dynamic "Write Interface.vi"("error in (no error)"=w1281, "Interface.lvclass"=w1282, "Channel in"=w1283) -> ("error out"=w1277:errorcluster, "Channel out"=w1276:refnum<class "Channel.lvclass">)  [unwired: 7 in]
              n529 = call-dynamic "Read State Machine.vi"("error in (no error)"=w1277, "Device in"=w1276) -> ("error out"=w1310:errorcluster, "State Machine.lvclass"=w1312:refnum<class "State Machine.lvclass">, "Device out"=w1308:refnum<class "Channel.lvclass">)  [unwired: 7 in]
              n530 = Increment(x=w1306) -> (x+1=w1305:u32)
              n531 = call "Next State.vi"("error in (no error)"=w1310, "New_State"=60, "State Machine in"=w1312) -> ("error out"=w1303:errorcluster, "State Machine out"=w1304:refnum<class "State Machine.lvclass">)  [unwired: 7 in]
              n532 = call-dynamic "Write State Machine.vi"("error in (no error)"=w1303, "State Machine.lvclass"=w1304, "Device in"=w1308) -> ("error out"=w1307:errorcluster, "Device out"=w1309:refnum<class "Channel.lvclass">)  [unwired: 7 in]
              n533 = call-dynamic "Write Channel.vi"("error in (no error)"=w1307, "Channel.lvclass"=w1309, "Acquisition in"=w1313) -> ("error out"=w1297:errorcluster, "Acquisition out"=w1298:refnum<class "Acquisition.lvclass">)  [unwired: 7 in]
              n534 = call-dynamic "Write AcquisitionD.vi"("error in (no error)"=w1297, "Acquisition.lvclass"=w1298, "S4ACS_GUI in"=w1299) -> ("error out"=w1296:errorcluster, "S4ACS_GUI out"=w1295:refnum<class "S4GUI.lvclass">)  [unwired: 7 in]
            }
            frame True {
            }
          }
          n535 = Bundle By Name(cluster=w1264, "Obs_state"=w1274) -> (w1273:refnum<class "S4GUI.lvclass">)
        }
        frame 266 {
          # "Espera terminar a execução do comando atual \nantes de ir ao proximo passo da Observação."
          n536 = call-dynamic "Read AcquisitionD.vi"("error in (no error)"=w1334, "S4ACS_GUI in"=w1335) -> ("error out"=w1340:errorcluster, "Acquisition.lvclass"=w1341:refnum<class "Acquisition.lvclass">, "S4ACS_GUI out"=w1337:refnum<class "S4GUI.lvclass">)  [unwired: 7 in]
          n537 = call-dynamic "Read Channel.vi"("error in (no error)"=w1340, "Acquisition in"=w1341) -> ("error out"=w1332:errorcluster, "Channel.lvclass"=w1331:refnum<class "Channel.lvclass">, "Acquisition out"=w1339:refnum<class "Acquisition.lvclass">)  [unwired: 7 in]
          n538 = call-dynamic "Read State Machine.vi"("error in (no error)"=w1332, "Device in"=w1331) -> ("error out"=w1323:errorcluster, "State Machine.lvclass"=w1325:refnum<class "State Machine.lvclass">, "Device out"=w1329:refnum<class "Channel.lvclass">)  [unwired: 7 in]
          n539 = call-dynamic "Read State.vi"("error in (no error)"=w1323, "State Machine in"=w1325) -> ("error out"=w1322:errorcluster, "State"=w1319:i32, "State Machine out"=w1324:refnum<class "State Machine.lvclass">)  [unwired: 7 in]
          n540 = Equal To 0?(x=w1319) -> (x = 0?=w1321:bool)
          n541 = call-dynamic "Write State Machine.vi"("error in (no error)"=w1322, "State Machine.lvclass"=w1324, "Device in"=w1329) -> ("error out"=w1328:errorcluster, "Device out"=w1330:refnum<class "Channel.lvclass">)  [unwired: 7 in]
          n542 = call-dynamic "Write Channel.vi"("error in (no error)"=w1328, "Channel.lvclass"=w1330, "Acquisition in"=w1339) -> ("error out"=w1336:errorcluster, "Acquisition out"=w1338:refnum<class "Acquisition.lvclass">)  [unwired: 7 in]
          n543 = Select(t=u32 299, s=w1321, f=w1318) -> (s? t:f=w1320:u32)
          n544 = call-dynamic "Write AcquisitionD.vi"("error in (no error)"=w1336, "Acquisition.lvclass"=w1338, "S4ACS_GUI in"=w1337) -> ("error out"=w1333:errorcluster, "S4ACS_GUI out"=w1327:refnum<class "S4GUI.lvclass">)  [unwired: 7 in]
          n545 = Bundle By Name(cluster=w1327, "Obs_state"=w1320) -> (w1326:refnum<class "S4GUI.lvclass">)
        }
        frame 299 {
          # "Verifica se é modo fotometria ou polarimetria:\nTrue = polarimetria\nFalse = fotometria"
          n546 = call "Read Instrument.lvclass.vi"("error in (no error)"=w1351, "S4ACS_GUI in"=w1352) -> ("error out"=w1346:errorcluster, "Instrument.lvclass"=w1347:refnum<class "Instrument.lvclass">, "S4ACS_GUI out"=w1345:refnum<class "S4GUI.lvclass">)  [unwired: 7 in]
          n547 = call-dynamic "Read mode.vi"("error in (no error)"=w1346, "Instrument in"=w1347) -> ("error out"=w1342:errorcluster, "mode"=w1344:bool)  [unwired: 7 in, 1 out]
          n548 = Select(t=u32 301, s=w1344, f=u32 321 ("t")) -> (s? t:f=w1349:u32)
          n549 = Bundle By Name(cluster=w1345, "Obs_state"=w1349) -> (w1350:refnum<class "S4GUI.lvclass">)
        }
        frame 301 {
          n550 = call "Read Instrument.lvclass.vi"("error in (no error)"=w1387, "S4ACS_GUI in"=w1388) -> ("error out"=w1391:errorcluster, "Instrument.lvclass"=w1392:refnum<class "Instrument.lvclass">, "S4ACS_GUI out"=w1389:refnum<class "S4GUI.lvclass">)  [unwired: 7 in]
          n551 = call "Read WPROT.vi"("error in (no error)"=w1391, "Instrument in"=w1392) -> ("error out"=w1380:errorcluster, "Opt_Selector.lvclass"=w1381:refnum<class "Opt_Selector.lvclass">, "Instrument out"=w1390:refnum<class "Instrument.lvclass">)  [unwired: 7 in]
          n552 = call-dynamic "getTargetPos.vi"("error in (no error)"=w1380, "Opt_Selector in"=w1381) -> ("error out"=w1379:errorcluster, "Target Pos"=w1359:u16, "Opt_Selector out"=w1378:refnum<class "Opt_Selector.lvclass">)  [unwired: 7 in]
          n553 = Build Array(-1.0 ("element"), 0.0 ("element"), 22.5 ("element"), 45.0 ("element"), 67.5 ("element"), 90.0 ("element"), 112.5 ("element"), 135.0 ("element"), 157.5 ("element"), 180.0 ("element"), 202.5 ("element"), 225.0 ("element"), 247.5 ("element"), 270.0 ("element"), 292.5 ("element"), 315.0 ("element"), 337.5 ("element")) -> (w1371:dbl[])
          n554 = Index Array(array=w1371, index=w1359) -> (element=w1358:dbl)
          n555 = case shown="1..16" w1359 {
            selector: w1359 -> [_ w1420]
            tunnel: w1390 -> [w1400 w1408]
            tunnel: [w1400 w1408] -> w1354
            tunnel: [w1397 w1407] -> w1353
            tunnel: w1384 -> [_ w1422]
            tunnel: [u32 311 w1421] -> w1383
            tunnel: w1379 -> [w1398 w1416]
            tunnel: w1378 -> [w1399 w1415]
            tunnel: w1358 -> [_ w1410]
            tunnel: [w1395 w1409] -> w1355
            frame 0, Default {
              # "Verifica os ciclos"
              # "Recupera a sequencia anterior para o caso \nde repetição da sequencia (sem precisar clicar \nnas posicoes desejadas novamente)."
              n556 = call-dynamic "Read sequencia_ant.vi"("error in (no error)"=w1398, "Opt_Selector in"=w1399) -> ("error out"=w1394:errorcluster, "sequencia_ant"=w1393:u16, "Opt_Selector out"=w1396:refnum<class "Opt_Selector.lvclass">)  [unwired: 7 in]
              n557 = call-dynamic "Write sequencia.vi"("error in (no error)"=w1394, "sequencia"=w1393, "Opt_Selector in"=w1396) -> ("error out"=w1397:errorcluster, "Opt_Selector out"=w1395:refnum<class "Opt_Selector.lvclass">)  [unwired: 7 in]
            }
            frame 1..16 {
              # "Espera até 10 x 1s (= 10s) para\nmecanismo entrar em READY"
              n558 = Number To Decimal String(number=w1420) -> (decimal integer string=w1419:string)  [unwired: 1 in]
              n559 = Concatenate Strings("WP" ("string"), w1419) -> (w1417:string)
              n560 = call "Write target name.vi"("error in (no error)"=w1416, "target name"=w1417, "Optics in"=w1415) -> ("error out"=w1413:errorcluster, "Optics out"=w1414:refnum<class "Opt_Selector.lvclass">)  [unwired: 7 in]
              n561 = call "Write target.vi"("error in (no error)"=w1413, "target"=w1410, "Optics in"=w1414) -> ("error out"=w1412:errorcluster, "Optics out"=w1411:refnum<class "Opt_Selector.lvclass">)  [unwired: 7 in]
              n562 = call-dynamic "Read State Machine.vi"("error in (no error)"=w1412, "Device in"=w1411) -> ("error out"=w1424:errorcluster, "State Machine.lvclass"=w1426:refnum<class "State Machine.lvclass">, "Device out"=w1423:refnum<class "Opt_Selector.lvclass">)  [unwired: 7 in]
              n563 = Increment(x=w1422) -> (x+1=w1421:u32)
              n564 = call "Next State.vi"("error in (no error)"=w1424, "New_State"=1, "State Machine in"=w1426) -> ("error out"=w1404:errorcluster, "State Machine out"=w1406:refnum<class "State Machine.lvclass">)  [unwired: 7 in]
              n565 = call-dynamic "Write Timer.vi"("error in (no error)"=w1404, "Timer"=u32 10, "State Machine in"=w1406) -> ("error out"=w1403:errorcluster, "State Machine out"=w1405:refnum<class "State Machine.lvclass">)  [unwired: 7 in]
              n566 = call-dynamic "Write State Machine.vi"("error in (no error)"=w1403, "State Machine.lvclass"=w1405, "Device in"=w1423) -> ("error out"=w1407:errorcluster, "Device out"=w1409:refnum<class "Opt_Selector.lvclass">)  [unwired: 7 in]
            }
          }
          n567 = call "Write WPROT.vi"("error in (no error)"=w1353, "Opt_Selector.lvclass"=w1355, "Instrument in"=w1354) -> ("error out"=w1357:errorcluster, "Instrument out"=w1356:refnum<class "Instrument.lvclass">)  [unwired: 7 in]
          n568 = call "Write Instrument.lvclass.vi"("error in (no error)"=w1357, "Instrument.lvclass"=w1356, "S4ACS_GUI in"=w1389) -> ("error out"=w1386:errorcluster, "S4ACS_GUI out"=w1385:refnum<class "S4GUI.lvclass">)  [unwired: 7 in]
          n569 = Bundle By Name(cluster=w1385, "Obs_state"=w1383) -> (w1382:refnum<class "S4GUI.lvclass">)
        }
        frame 302 {
          # "Espera terminar o movimento para a posição \"target\" do waveplate\nantes de ir para o estado de pausa."
          n570 = call "Read Instrument.lvclass.vi"("error in (no error)"=w1444, "S4ACS_GUI in"=w1445) -> ("error out"=w1450:errorcluster, "Instrument.lvclass"=w1451:refnum<class "Instrument.lvclass">, "S4ACS_GUI out"=w1447:refnum<class "S4GUI.lvclass">)  [unwired: 7 in]
          n571 = call "Read WPROT.vi"("error in (no error)"=w1450, "Instrument in"=w1451) -> ("error out"=w1440:errorcluster, "Opt_Selector.lvclass"=w1439:refnum<class "Opt_Selector.lvclass">, "Instrument out"=w1449:refnum<class "Instrument.lvclass">)  [unwired: 7 in]
          n572 = call-dynamic "Read State Machine.vi"("error in (no error)"=w1440, "Device in"=w1439) -> ("error out"=w1441:errorcluster, "State Machine.lvclass"=w1442:refnum<class "State Machine.lvclass">, "Device out"=w1437:refnum<class "Opt_Selector.lvclass">)  [unwired: 7 in]
          n573 = Increment(x=w1430) -> (x+1=w1429:u32)
          n574 = call-dynamic "Read State.vi"("error in (no error)"=w1441, "State Machine in"=w1442) -> ("error out"=w1427:errorcluster, "State"=w1432:i32, "State Machine out"=w1428:refnum<class "State Machine.lvclass">)  [unwired: 7 in]
          n575 = Equal To 0?(x=w1432) -> (x = 0?=w1433:bool)
          n576 = call-dynamic "Write State Machine.vi"("error in (no error)"=w1427, "State Machine.lvclass"=w1428, "Device in"=w1437) -> ("error out"=w1436:errorcluster, "Device out"=w1438:refnum<class "Opt_Selector.lvclass">)  [unwired: 7 in]
          n577 = call "Write WPROT.vi"("error in (no error)"=w1436, "Opt_Selector.lvclass"=w1438, "Instrument in"=w1449) -> ("error out"=w1446:errorcluster, "Instrument out"=w1448:refnum<class "Instrument.lvclass">)  [unwired: 7 in]
          n578 = Select(t=w1429, s=w1433, f=w1430) -> (s? t:f=w1431:u32)
          n579 = call "Write Instrument.lvclass.vi"("error in (no error)"=w1446, "Instrument.lvclass"=w1448, "S4ACS_GUI in"=w1447) -> ("error out"=w1443:errorcluster, "S4ACS_GUI out"=w1435:refnum<class "S4GUI.lvclass">)  [unwired: 7 in]
          n580 = Bundle By Name(cluster=w1435, "Obs_state"=w1431) -> (w1434:refnum<class "S4GUI.lvclass">)
        }
        frame 303 {
          # "Espera terminar a pausa carregada no Timer"
          n581 = call "Read Instrument.lvclass.vi"("error in (no error)"=w1468, "S4ACS_GUI in"=w1469) -> ("error out"=w1474:errorcluster, "Instrument.lvclass"=w1475:refnum<class "Instrument.lvclass">, "S4ACS_GUI out"=w1471:refnum<class "S4GUI.lvclass">)  [unwired: 7 in]
          n582 = call "Read WPROT.vi"("error in (no error)"=w1474, "Instrument in"=w1475) -> ("error out"=w1466:errorcluster, "Opt_Selector.lvclass"=w1465:refnum<class "Opt_Selector.lvclass">, "Instrument out"=w1473:refnum<class "Instrument.lvclass">)  [unwired: 7 in]
          n583 = call-dynamic "Read State Machine.vi"("error in (no error)"=w1466, "Device in"=w1465) -> ("error out"=w1455:errorcluster, "State Machine.lvclass"=w1456:refnum<class "State Machine.lvclass">, "Device out"=w1463:refnum<class "Opt_Selector.lvclass">)  [unwired: 7 in]
          n584 = Increment(x=w1452) -> (x+1=w1457:u32)
          n585 = call "Verify Timer.vi"("error in (no error)"=w1455, "State Machine in"=w1456) -> ("error out"=w1453:errorcluster, "timeout"=w1458:bool, "State Machine out"=w1454:refnum<class "State Machine.lvclass">)  [unwired: 7 in]
          n586 = call-dynamic "Write State Machine.vi"("error in (no error)"=w1453, "State Machine.lvclass"=w1454, "Device in"=w1463) -> ("error out"=w1462:errorcluster, "Device out"=w1464:refnum<class "Opt_Selector.lvclass">)  [unwired: 7 in]
          n587 = call "Write WPROT.vi"("error in (no error)"=w1462, "Opt_Selector.lvclass"=w1464, "Instrument in"=w1473) -> ("error out"=w1470:errorcluster, "Instrument out"=w1472:refnum<class "Instrument.lvclass">)  [unwired: 7 in]
          n588 = call "Write Instrument.lvclass.vi"("error in (no error)"=w1470, "Instrument.lvclass"=w1472, "S4ACS_GUI in"=w1471) -> ("error out"=w1467:errorcluster, "S4ACS_GUI out"=w1461:refnum<class "S4GUI.lvclass">)  [unwired: 7 in]
          n589 = Select(t=w1457, s=w1458, f=w1452) -> (s? t:f=w1459:u32)
          n590 = Bundle By Name(cluster=w1461, "Obs_state"=w1459) -> (w1460:refnum<class "S4GUI.lvclass">)
        }
        frame 304 {
          n591 = call-dynamic "Read Sync Box.lvclass.vi"("error in (no error)"=w1486, "SPARC4_AC in"=w1487) -> ("error out"=w1478:errorcluster, "Sync Box.lvclass"=w1480:refnum<class "Sync Box.lvclass">, "SPARC4_AC out"=w1489:refnum<class "S4GUI.lvclass">)  [unwired: 7 in]
          n592 = call "Read connection.vi"("error in (no error)"=w1478, "Server in"=w1480) -> ("error out"=w1477:errorcluster, "connection"=w1476:bool, "Server out"=w1479:refnum<class "Sync Box.lvclass">)  [unwired: 7 in]
          n593 = case shown="True" w1476 {
            tunnel: w1477 -> [w1494 w1515]
            tunnel: [w1495 w1513] -> w1490
            tunnel: [w1494 w1512] -> w1488
            tunnel: w1483 -> [w1493 w1503]
            tunnel: [w1491 w1502] -> w1482
            tunnel: w1479 -> [w1495 w1496]
            frame False {
              n594 = Increment(x=w1493) -> (x+1=w1492:u32)
              n595 = Increment(x=w1492) -> (x+1=w1491:u32)
            }
            frame True {
              # "configura delays do syncBox"
              n596 = call-dynamic "Read Trigger.lvclass.vi"("error in (no error)"=w1515, "Sync Box in"=w1496) -> ("error out"=w1508:errorcluster, "Trigger.lvclass"=w1507:refnum<class "Trigger.lvclass">, "Sync Box out"=w1514:refnum<class "Sync Box.lvclass">)  [unwired: 7 in]
              n597 = call-dynamic "Read State Machine.vi"("error in (no error)"=w1508, "Device in"=w1507) -> ("error out"=w1509:errorcluster, "State Machine.lvclass"=w1511:refnum<class "State Machine.lvclass">, "Device out"=w1505:refnum<class "Trigger.lvclass">)  [unwired: 7 in]
              n598 = call "Next State.vi"("error in (no error)"=w1509, "New_State"=10, "State Machine in"=w1511) -> ("error out"=w1498:errorcluster, "State Machine out"=w1500:refnum<class "State Machine.lvclass">)  [unwired: 7 in]
              n599 = Increment(x=w1503) -> (x+1=w1502:u32)
              n600 = call-dynamic "Write Timer.vi"("error in (no error)"=w1498, "Timer"=u32 5, "State Machine in"=w1500) -> ("error out"=w1497:errorcluster, "State Machine out"=w1499:refnum<class "State Machine.lvclass">)  [unwired: 7 in]
              n601 = call-dynamic "Write State Machine.vi"("error in (no error)"=w1497, "State Machine.lvclass"=w1499, "Device in"=w1505) -> ("error out"=w1504:errorcluster, "Device out"=w1506:refnum<class "Trigger.lvclass">)  [unwired: 7 in]
              n602 = call-dynamic "Write Trigger.lvclass.vi"("error in (no error)"=w1504, "Trigger.lvclass"=w1506, "Sync Box in"=w1514) -> ("error out"=w1512:errorcluster, "Sync Box out"=w1513:refnum<class "Sync Box.lvclass">)  [unwired: 7 in]
            }
          }
          n603 = call-dynamic "Write Sync Box.lvclass.vi"("error in (no error)"=w1488, "Sync Box.lvclass"=w1490, "SPARC4_AC in"=w1489) -> ("error out"=w1485:errorcluster, "SPARC4_AC out"=w1484:refnum<class "S4GUI.lvclass">)  [unwired: 7 in]
          n604 = Bundle By Name(cluster=w1484, "Obs_state"=w1482) -> (w1481:refnum<class "S4GUI.lvclass">)
        }
        frame 305 {
          # "Espera terminar a execução do comando atual \nantes de ir ao proximo passo da Observação."
          n605 = call-dynamic "Read Sync Box.lvclass.vi"("error in (no error)"=w1533, "SPARC4_AC in"=w1534) -> ("error out"=w1539:errorcluster, "Sync Box.lvclass"=w1540:refnum<class "Sync Box.lvclass">, "SPARC4_AC out"=w1536:refnum<class "S4GUI.lvclass">)  [unwired: 7 in]
          n606 = call-dynamic "Read Trigger.lvclass.vi"("error in (no error)"=w1539, "Sync Box in"=w1540) -> ("error out"=w1531:errorcluster, "Trigger.lvclass"=w1530:refnum<class "Trigger.lvclass">, "Sync Box out"=w1538:refnum<class "Sync Box.lvclass">)  [unwired: 7 in]
          n607 = call-dynamic "Read State Machine.vi"("error in (no error)"=w1531, "Device in"=w1530) -> ("error out"=w1522:errorcluster, "State Machine.lvclass"=w1524:refnum<class "State Machine.lvclass">, "Device out"=w1528:refnum<class "Trigger.lvclass">)  [unwired: 7 in]
          n608 = call-dynamic "Read State.vi"("error in (no error)"=w1522, "State Machine in"=w1524) -> ("error out"=w1521:errorcluster, "State"=w1518:i32, "State Machine out"=w1523:refnum<class "State Machine.lvclass">)  [unwired: 7 in]
          n609 = Equal To 0?(x=w1518) -> (x = 0?=w1520:bool)
          n610 = call-dynamic "Write State Machine.vi"("error in (no error)"=w1521, "State Machine.lvclass"=w1523, "Device in"=w1528) -> ("error out"=w1527:errorcluster, "Device out"=w1529:refnum<class "Trigger.lvclass">)  [unwired: 7 in]
          n611 = call-dynamic "Write Trigger.lvclass.vi"("error in (no error)"=w1527, "Trigger.lvclass"=w1529, "Sync Box in"=w1538) -> ("error out"=w1535:errorcluster, "Sync Box out"=w1537:refnum<class "Sync Box.lvclass">)  [unwired: 7 in]
          n612 = Increment(x=w1517) -> (x+1=w1516:u32)
          n613 = Select(t=w1516, s=w1520, f=w1517) -> (s? t:f=w1519:u32)
          n614 = call-dynamic "Write Sync Box.lvclass.vi"("error in (no error)"=w1535, "Sync Box.lvclass"=w1537, "SPARC4_AC in"=w1536) -> ("error out"=w1532:errorcluster, "SPARC4_AC out"=w1526:refnum<class "S4GUI.lvclass">)  [unwired: 7 in]
          n615 = Bundle By Name(cluster=w1526, "Obs_state"=w1519) -> (w1525:refnum<class "S4GUI.lvclass">)
        }
        frame 306 {
          n616 = call-dynamic "Read AcquisitionA.vi"("error in (no error)"=w1581, "S4ACS_GUI in"=w1582) -> ("error out"=w1557:errorcluster, "Acquisition.lvclass"=w1560:refnum<class "Acquisition.lvclass">, "S4ACS_GUI out"=w1584:refnum<class "S4GUI.lvclass">)  [unwired: 7 in]
          n617 = call "Read connection.vi"("error in (no error)"=w1557, "Server in"=w1560) -> ("error out"=w1556:errorcluster, "connection"=w1558:bool, "Server out"=w1559:refnum<class "Acquisition.lvclass">)  [unwired: 7 in]
          n618 = case shown="True" w1558 {
            tunnel: w1559 -> [w1638 w1653]
            tunnel: w1556 -> [w1637 w1652]
            tunnel: [w1638 w1650] -> w1585
            tunnel: [w1637 w1649] -> w1583
            frame False {
            }
            frame True {
              n619 = call-dynamic "Read Channel.vi"("error in (no error)"=w1652, "Acquisition in"=w1653) -> ("error out"=w1645:errorcluster, "Channel.lvclass"=w1644:refnum<class "Channel.lvclass">, "Acquisition out"=w1651:refnum<class "Acquisition.lvclass">)  [unwired: 7 in]
              n620 = call-dynamic "Read State Machine.vi"("error in (no error)"=w1645, "Device in"=w1644) -> ("error out"=w1646:errorcluster, "State Machine.lvclass"=w1648:refnum<class "State Machine.lvclass">, "Device out"=w1642:refnum<class "Channel.lvclass">)  [unwired: 7 in]
              n621 = call "Next State.vi"("error in (no error)"=w1646, "New_State"=50, "State Machine in"=w1648) -> ("error out"=w1639:errorcluster, "State Machine out"=w1640:refnum<class "State Machine.lvclass">)  [unwired: 7 in]
              n622 = call-dynamic "Write State Machine.vi"("error in (no error)"=w1639, "State Machine.lvclass"=w1640, "Device in"=w1642) -> ("error out"=w1641:errorcluster, "Device out"=w1643:refnum<class "Channel.lvclass">)  [unwired: 7 in]
              n623 = call-dynamic "Write Channel.vi"("error in (no error)"=w1641, "Channel.lvclass"=w1643, "Acquisition in"=w1651) -> ("error out"=w1649:errorcluster, "Acquisition out"=w1650:refnum<class "Acquisition.lvclass">)  [unwired: 7 in]
            }
          }
          n624 = call-dynamic "Write AcquisitionA.vi"("error in (no error)"=w1583, "Acquisition.lvclass"=w1585, "S4ACS_GUI in"=w1584) -> ("error out"=w1576:errorcluster, "S4ACS_GUI out"=w1577:refnum<class "S4GUI.lvclass">)  [unwired: 7 in]
          n625 = call "Read AcquisitionB.vi"("error in (no error)"=w1576, "S4ACS_GUI in"=w1577) -> ("error out"=w1553:errorcluster, "Acquisition.lvclass"=w1555:refnum<class "Acquisition.lvclass">, "S4ACS_GUI out"=w1574:refnum<class "S4GUI.lvclass">)  [unwired: 7 in]
          n626 = call "Read connection.vi"("error in (no error)"=w1553, "Server in"=w1555) -> ("error out"=w1552:errorcluster, "connection"=w1551:bool, "Server out"=w1554:refnum<class "Acquisition.lvclass">)  [unwired: 7 in]
          n627 = case shown="True" w1551 {
            tunnel: w1554 -> [w1621 w1636]
            tunnel: w1552 -> [w1620 w1635]
            tunnel: [w1621 w1633] -> w1575
            tunnel: [w1620 w1632] -> w1573
            frame False {
            }
            frame True {
              n628 = call-dynamic "Read Channel.vi"("error in (no error)"=w1635, "Acquisition in"=w1636) -> ("error out"=w1628:errorcluster, "Channel.lvclass"=w1627:refnum<class "Channel.lvclass">, "Acquisition out"=w1634:refnum<class "Acquisition.lvclass">)  [unwired: 7 in]
              n629 = call-dynamic "Read State Machine.vi"("error in (no error)"=w1628, "Device in"=w1627) -> ("error out"=w1629:errorcluster, "State Machine.lvclass"=w1631:refnum<class "State Machine.lvclass">, "Device out"=w1625:refnum<class "Channel.lvclass">)  [unwired: 7 in]
              n630 = call "Next State.vi"("error in (no error)"=w1629, "New_State"=50, "State Machine in"=w1631) -> ("error out"=w1622:errorcluster, "State Machine out"=w1623:refnum<class "State Machine.lvclass">)  [unwired: 7 in]
              n631 = call-dynamic "Write State Machine.vi"("error in (no error)"=w1622, "State Machine.lvclass"=w1623, "Device in"=w1625) -> ("error out"=w1624:errorcluster, "Device out"=w1626:refnum<class "Channel.lvclass">)  [unwired: 7 in]
              n632 = call-dynamic "Write Channel.vi"("error in (no error)"=w1624, "Channel.lvclass"=w1626, "Acquisition in"=w1634) -> ("error out"=w1632:errorcluster, "Acquisition out"=w1633:refnum<class "Acquisition.lvclass">)  [unwired: 7 in]
            }
          }
          n633 = call "Write AcquisitionB.vi"("error in (no error)"=w1573, "Acquisition.lvclass"=w1575, "S4ACS_GUI in"=w1574) -> ("error out"=w1569:errorcluster, "S4ACS_GUI out"=w1568:refnum<class "S4GUI.lvclass">)  [unwired: 7 in]
          n634 = call-dynamic "Read AcquisitionC.vi"("error in (no error)"=w1569, "S4ACS_GUI in"=w1568) -> ("error out"=w1548:errorcluster, "Acquisition.lvclass"=w1550:refnum<class "Acquisition.lvclass">, "S4ACS_GUI out"=w1571:refnum<class "S4GUI.lvclass">)  [unwired: 7 in]
          n635 = call "Read connection.vi"("error in (no error)"=w1548, "Server in"=w1550) -> ("error out"=w1547:errorcluster, "connection"=w1546:bool, "Server out"=w1549:refnum<class "Acquisition.lvclass">)  [unwired: 7 in]
          n636 = case shown="True" w1546 {
            tunnel: [w1603 w1611] -> w1572
            tunnel: [w1604 w1610] -> w1570
            tunnel: w1549 -> [w1604 w1608]
            tunnel: w1547 -> [w1603 w1607]
            frame False {
            }
            frame True {
              n637 = call-dynamic "Read Channel.vi"("error in (no error)"=w1607, "Acquisition in"=w1608) -> ("error out"=w1615:errorcluster, "Channel.lvclass"=w1616:refnum<class "Channel.lvclass">, "Acquisition out"=w1609:refnum<class "Acquisition.lvclass">)  [unwired: 7 in]
              n638 = call-dynamic "Read State Machine.vi"("error in (no error)"=w1615, "Device in"=w1616) -> ("error out"=w1614:errorcluster, "State Machine.lvclass"=w1612:refnum<class "State Machine.lvclass">, "Device out"=w1618:refnum<class "Channel.lvclass">)  [unwired: 7 in]
              n639 = call "Next State.vi"("error in (no error)"=w1614, "New_State"=50, "State Machine in"=w1612) -> ("error out"=w1606:errorcluster, "State Machine out"=w1605:refnum<class "State Machine.lvclass">)  [unwired: 7 in]
              n640 = call-dynamic "Write State Machine.vi"("error in (no error)"=w1606, "State Machine.lvclass"=w1605, "Device in"=w1618) -> ("error out"=w1619:errorcluster, "Device out"=w1617:refnum<class "Channel.lvclass">)  [unwired: 7 in]
              n641 = call-dynamic "Write Channel.vi"("error in (no error)"=w1619, "Channel.lvclass"=w1617, "Acquisition in"=w1609) -> ("error out"=w1611:errorcluster, "Acquisition out"=w1610:refnum<class "Acquisition.lvclass">)  [unwired: 7 in]
            }
          }
          n642 = call-dynamic "Write AcquisitionC.vi"("error in (no error)"=w1572, "Acquisition.lvclass"=w1570, "S4ACS_GUI in"=w1571) -> ("error out"=w1566:errorcluster, "S4ACS_GUI out"=w1565:refnum<class "S4GUI.lvclass">)  [unwired: 7 in]
          n643 = call-dynamic "Read AcquisitionD.vi"("error in (no error)"=w1566, "S4ACS_GUI in"=w1565) -> ("error out"=w1543:errorcluster, "Acquisition.lvclass"=w1545:refnum<class "Acquisition.lvclass">, "S4ACS_GUI out"=w1564:refnum<class "S4GUI.lvclass">)  [unwired: 7 in]
          n644 = call "Read connection.vi"("error in (no error)"=w1543, "Server in"=w1545) -> ("error out"=w1542:errorcluster, "connection"=w1541:bool, "Server out"=w1544:refnum<class "Acquisition.lvclass">)  [unwired: 7 in]
          n645 = case shown="True" w1541 {
            tunnel: w1542 -> [w1586 w1602]
            tunnel: [w1586 w1601] -> w1567
            tunnel: w1544 -> [w1587 w1592]
            tunnel: [w1587 w1590] -> w1563
            frame False {
            }
            frame True {
              n646 = call-dynamic "Read Channel.vi"("error in (no error)"=w1602, "Acquisition in"=w1592) -> ("error out"=w1597:errorcluster, "Channel.lvclass"=w1596:refnum<class "Channel.lvclass">, "Acquisition out"=w1591:refnum<class "Acquisition.lvclass">)  [unwired: 7 in]
              n647 = call-dynamic "Read State Machine.vi"("error in (no error)"=w1597, "Device in"=w1596) -> ("error out"=w1598:errorcluster, "State Machine.lvclass"=w1600:refnum<class "State Machine.lvclass">, "Device out"=w1594:refnum<class "Channel.lvclass">)  [unwired: 7 in]
              n648 = call "Next State.vi"("error in (no error)"=w1598, "New_State"=50, "State Machine in"=w1600) -> ("error out"=w1588:errorcluster, "State Machine out"=w1589:refnum<class "State Machine.lvclass">)  [unwired: 7 in]
              n649 = call-dynamic "Write State Machine.vi"("error in (no error)"=w1588, "State Machine.lvclass"=w1589, "Device in"=w1594) -> ("error out"=w1593:errorcluster, "Device out"=w1595:refnum<class "Channel.lvclass">)  [unwired: 7 in]
              n650 = call-dynamic "Write Channel.vi"("error in (no error)"=w1593, "Channel.lvclass"=w1595, "Acquisition in"=w1591) -> ("error out"=w1601:errorcluster, "Acquisition out"=w1590:refnum<class "Acquisition.lvclass">)  [unwired: 7 in]
            }
          }
          n651 = call-dynamic "Write AcquisitionD.vi"("error in (no error)"=w1567, "Acquisition.lvclass"=w1563, "S4ACS_GUI in"=w1564) -> ("error out"=w1562:errorcluster, "S4ACS_GUI out"=w1561:refnum<class "S4GUI.lvclass">)  [unwired: 7 in]
          n652 = Increment(x=w1580) -> (x+1=w1579:u32)
          n653 = Bundle By Name(cluster=w1561, "Obs_state"=w1579) -> (w1578:refnum<class "S4GUI.lvclass">)
        }
        frame 307 {
          # "Espera todos os canais chegarem ao estado ACTIVE\n(estados 54 e 55 de Channel:Run.vi)."
          n654 = call-dynamic "Read AcquisitionA.vi"("error in (no error)"=w1700, "S4ACS_GUI in"=w1701) -> ("error out"=w1677:errorcluster, "Acquisition.lvclass"=w1678:refnum<class "Acquisition.lvclass">, "S4ACS_GUI out"=w1703:refnum<class "S4GUI.lvclass">)  [unwired: 7 in]
          n655 = call "Read connection.vi"("error in (no error)"=w1677, "Server in"=w1678) -> ("error out"=w1679:errorcluster, "connection"=w1681:bool, "Server out"=w1680:refnum<class "Acquisition.lvclass">)  [unwired: 7 in]
          n656 = case shown="True" w1681 {
            tunnel: [w1767 w1783] -> w1704
            tunnel: [w1766 w1782] -> w1702
            tunnel: w1680 -> [w1767 w1772]
            tunnel: w1679 -> [w1766 w1771]
            tunnel: [TRUE w1770] -> w1657
            frame False {
            }
            frame True {
              n657 = call-dynamic "Read Channel.vi"("error in (no error)"=w1771, "Acquisition in"=w1772) -> ("error out"=w1781:errorcluster, "Channel.lvclass"=w1780:refnum<class "Channel.lvclass">, "Acquisition out"=w1784:refnum<class "Acquisition.lvclass">)  [unwired: 7 in]
              n658 = call-dynamic "Read State Machine.vi"("error in (no error)"=w1781, "Device in"=w1780) -> ("error out"=w1774:errorcluster, "State Machine.lvclass"=w1776:refnum<class "State Machine.lvclass">, "Device out"=w1778:refnum<class "Channel.lvclass">)  [unwired: 7 in]
              n659 = call-dynamic "Read State.vi"("error in (no error)"=w1774, "State Machine in"=w1776) -> ("error out"=w1773:errorcluster, "State"=w1769:i32, "State Machine out"=w1775:refnum<class "State Machine.lvclass">)  [unwired: 7 in]
              n660 = Greater?(x=w1769, y=53) -> (0:w1770:bool)
              n661 = call-dynamic "Write State Machine.vi"("error in (no error)"=w1773, "State Machine.lvclass"=w1775, "Device in"=w1778) -> ("error out"=w1777:errorcluster, "Device out"=w1779:refnum<class "Channel.lvclass">)  [unwired: 7 in]
              n662 = call-dynamic "Write Channel.vi"("error in (no error)"=w1777, "Channel.lvclass"=w1779, "Acquisition in"=w1784) -> ("error out"=w1782:errorcluster, "Acquisition out"=w1783:refnum<class "Acquisition.lvclass">)  [unwired: 7 in]
            }
          }
          n663 = call-dynamic "Write AcquisitionA.vi"("error in (no error)"=w1702, "Acquisition.lvclass"=w1704, "S4ACS_GUI in"=w1703) -> ("error out"=w1696:errorcluster, "S4ACS_GUI out"=w1697:refnum<class "S4GUI.lvclass">)  [unwired: 7 in]
          n664 = call "Read AcquisitionB.vi"("error in (no error)"=w1696, "S4ACS_GUI in"=w1697) -> ("error out"=w1674:errorcluster, "Acquisition.lvclass"=w1676:refnum<class "Acquisition.lvclass">, "S4ACS_GUI out"=w1694:refnum<class "S4GUI.lvclass">)  [unwired: 7 in]
          n665 = call "Read connection.vi"("error in (no error)"=w1674, "Server in"=w1676) -> ("error out"=w1673:errorcluster, "connection"=w1672:bool, "Server out"=w1675:refnum<class "Acquisition.lvclass">)  [unwired: 7 in]
          n666 = case shown="True" w1672 {
            tunnel: w1675 -> [w1747 w1764]
            tunnel: w1673 -> [w1746 w1763]
            tunnel: [w1747 w1761] -> w1695
            tunnel: [w1746 w1760] -> w1693
            tunnel: [TRUE w1749] -> w1656
            frame False {
            }
            frame True {
              n667 = call-dynamic "Read Channel.vi"("error in (no error)"=w1763, "Acquisition in"=w1764) -> ("error out"=w1759:errorcluster, "Channel.lvclass"=w1758:refnum<class "Channel.lvclass">, "Acquisition out"=w1762:refnum<class "Acquisition.lvclass">)  [unwired: 7 in]
              n668 = call-dynamic "Read State Machine.vi"("error in (no error)"=w1759, "Device in"=w1758) -> ("error out"=w1752:errorcluster, "State Machine.lvclass"=w1754:refnum<class "State Machine.lvclass">, "Device out"=w1756:refnum<class "Channel.lvclass">)  [unwired: 7 in]
              n669 = call-dynamic "Read State.vi"("error in (no error)"=w1752, "State Machine in"=w1754) -> ("error out"=w1751:errorcluster, "State"=w1748:i32, "State Machine out"=w1753:refnum<class "State Machine.lvclass">)  [unwired: 7 in]
              n670 = Greater?(x=w1748, y=53) -> (0:w1749:bool)
              n671 = call-dynamic "Write State Machine.vi"("error in (no error)"=w1751, "State Machine.lvclass"=w1753, "Device in"=w1756) -> ("error out"=w1755:errorcluster, "Device out"=w1757:refnum<class "Channel.lvclass">)  [unwired: 7 in]
              n672 = call-dynamic "Write Channel.vi"("error in (no error)"=w1755, "Channel.lvclass"=w1757, "Acquisition in"=w1762) -> ("error out"=w1760:errorcluster, "Acquisition out"=w1761:refnum<class "Acquisition.lvclass">)  [unwired: 7 in]
            }
          }
          n673 = call "Write AcquisitionB.vi"("error in (no error)"=w1693, "Acquisition.lvclass"=w1695, "S4ACS_GUI in"=w1694) -> ("error out"=w1689:errorcluster, "S4ACS_GUI out"=w1688:refnum<class "S4GUI.lvclass">)  [unwired: 7 in]
          n674 = call-dynamic "Read AcquisitionC.vi"("error in (no error)"=w1689, "S4ACS_GUI in"=w1688) -> ("error out"=w1669:errorcluster, "Acquisition.lvclass"=w1671:refnum<class "Acquisition.lvclass">, "S4ACS_GUI out"=w1691:refnum<class "S4GUI.lvclass">)  [unwired: 7 in]
          n675 = call "Read connection.vi"("error in (no error)"=w1669, "Server in"=w1671) -> ("error out"=w1668:errorcluster, "connection"=w1667:bool, "Server out"=w1670:refnum<class "Acquisition.lvclass">)  [unwired: 7 in]
          n676 = case shown="True" w1667 {
            tunnel: [w1726 w1737] -> w1692
            tunnel: [w1727 w1736] -> w1690
            tunnel: w1670 -> [w1727 w1732]
            tunnel: w1668 -> [w1726 w1731]
            tunnel: [TRUE w1728] -> w1655
            frame False {
            }
            frame True {
              n677 = call-dynamic "Read Channel.vi"("error in (no error)"=w1731, "Acquisition in"=w1732) -> ("error out"=w1738:errorcluster, "Channel.lvclass"=w1739:refnum<class "Channel.lvclass">, "Acquisition out"=w1735:refnum<class "Acquisition.lvclass">)  [unwired: 7 in]
              n678 = call-dynamic "Read State Machine.vi"("error in (no error)"=w1738, "Device in"=w1739) -> ("error out"=w1733:errorcluster, "State Machine.lvclass"=w1743:refnum<class "State Machine.lvclass">, "Device out"=w1741:refnum<class "Channel.lvclass">)  [unwired: 7 in]
              n679 = call-dynamic "Read State.vi"("error in (no error)"=w1733, "State Machine in"=w1743) -> ("error out"=w1734:errorcluster, "State"=w1729:i32, "State Machine out"=w1744:refnum<class "State Machine.lvclass">)  [unwired: 7 in]
              n680 = Greater?(x=w1729, y=53) -> (0:w1728:bool)
              n681 = call-dynamic "Write State Machine.vi"("error in (no error)"=w1734, "State Machine.lvclass"=w1744, "Device in"=w1741) -> ("error out"=w1742:errorcluster, "Device out"=w1740:refnum<class "Channel.lvclass">)  [unwired: 7 in]
              n682 = call-dynamic "Write Channel.vi"("error in (no error)"=w1742, "Channel.lvclass"=w1740, "Acquisition in"=w1735) -> ("error out"=w1737:errorcluster, "Acquisition out"=w1736:refnum<class "Acquisition.lvclass">)  [unwired: 7 in]
            }
          }
          n683 = call-dynamic "Write AcquisitionC.vi"("error in (no error)"=w1692, "Acquisition.lvclass"=w1690, "S4ACS_GUI in"=w1691) -> ("error out"=w1666:errorcluster, "S4ACS_GUI out"=w1684:refnum<class "S4GUI.lvclass">)  [unwired: 7 in]
          n684 = call-dynamic "Read AcquisitionD.vi"("error in (no error)"=w1666, "S4ACS_GUI in"=w1684) -> ("error out"=w1662:errorcluster, "Acquisition.lvclass"=w1665:refnum<class "Acquisition.lvclass">, "S4ACS_GUI out"=w1686:refnum<class "S4GUI.lvclass">)  [unwired: 7 in]
          n685 = call "Read connection.vi"("error in (no error)"=w1662, "Server in"=w1665) -> ("error out"=w1663:errorcluster, "connection"=w1661:bool, "Server out"=w1664:refnum<class "Acquisition.lvclass">)  [unwired: 7 in]
          n686 = case shown="True" w1661 {
            tunnel: [w1707 w1723] -> w1687
            tunnel: [w1706 w1722] -> w1685
            tunnel: [TRUE w1709] -> w1654
            tunnel: w1664 -> [w1707 w1712]
            tunnel: w1663 -> [w1706 w1711]
            frame False {
            }
            frame True {
              n687 = call-dynamic "Read Channel.vi"("error in (no error)"=w1711, "Acquisition in"=w1712) -> ("error out"=w1721:errorcluster, "Channel.lvclass"=w1720:refnum<class "Channel.lvclass">, "Acquisition out"=w1724:refnum<class "Acquisition.lvclass">)  [unwired: 7 in]
              n688 = call-dynamic "Read State Machine.vi"("error in (no error)"=w1721, "Device in"=w1720) -> ("error out"=w1714:errorcluster, "State Machine.lvclass"=w1716:refnum<class "State Machine.lvclass">, "Device out"=w1718:refnum<class "Channel.lvclass">)  [unwired: 7 in]
              n689 = call-dynamic "Read State.vi"("error in (no error)"=w1714, "State Machine in"=w1716) -> ("error out"=w1713:errorcluster, "State"=w1708:i32, "State Machine out"=w1715:refnum<class "State Machine.lvclass">)  [unwired: 7 in]
              n690 = Greater?(x=w1708, y=53) -> (0:w1709:bool)
              n691 = call-dynamic "Write State Machine.vi"("error in (no error)"=w1713, "State Machine.lvclass"=w1715, "Device in"=w1718) -> ("error out"=w1717:errorcluster, "Device out"=w1719:refnum<class "Channel.lvclass">)  [unwired: 7 in]
              n692 = call-dynamic "Write Channel.vi"("error in (no error)"=w1717, "Channel.lvclass"=w1719, "Acquisition in"=w1724) -> ("error out"=w1722:errorcluster, "Acquisition out"=w1723:refnum<class "Acquisition.lvclass">)  [unwired: 7 in]
            }
          }
          n693 = call-dynamic "Write AcquisitionD.vi"("error in (no error)"=w1685, "Acquisition.lvclass"=w1687, "S4ACS_GUI in"=w1686) -> ("error out"=w1682:errorcluster, "S4ACS_GUI out"=w1683:refnum<class "S4GUI.lvclass">)  [unwired: 7 in]
          n694 = Compound Arithmetic op=AND(w1657, w1656, w1655, w1654) -> (w1658:bool)
          n695 = Increment(x=w1660) -> (x+1=w1659:u32)
          n696 = Select(t=w1659, s=w1658, f=w1660) -> (s? t:f=w1698:u32)
          n697 = Bundle By Name(cluster=w1683, "Obs_state"=w1698) -> (w1699:refnum<class "S4GUI.lvclass">)
        }
        frame 308 {
          # "Dispara o comando para o dispositivo corrente."
          n698 = call-dynamic "Read Sync Box.lvclass.vi"("error in (no error)"=w1795, "SPARC4_AC in"=w1796) -> ("error out"=w1787:errorcluster, "Sync Box.lvclass"=w1789:refnum<class "Sync Box.lvclass">, "SPARC4_AC out"=w1798:refnum<class "S4GUI.lvclass">)  [unwired: 7 in]
          n699 = call "Read connection.vi"("error in (no error)"=w1787, "Server in"=w1789) -> ("error out"=w1786:errorcluster, "connection"=w1785:bool, "Server out"=w1788:refnum<class "Sync Box.lvclass">)  [unwired: 7 in]
          n700 = case shown="True" w1785 {
            tunnel: w1786 -> [w1803 w1821]
            tunnel: [w1804 w1819] -> w1799
            tunnel: [w1803 w1818] -> w1797
            tunnel: w1792 -> [w1802 w1809]
            tunnel: [w1800 w1808] -> w1791
            tunnel: w1788 -> [w1804 w1807]
            frame False {
              n701 = Increment(x=w1802) -> (x+1=w1801:u32)
              n702 = Increment(x=w1801) -> (x+1=w1800:u32)
            }
            frame True {
              # "envia comando TRIGGER para o SyncBox"
              n703 = call-dynamic "Read Trigger.lvclass.vi"("error in (no error)"=w1821, "Sync Box in"=w1807) -> ("error out"=w1814:errorcluster, "Trigger.lvclass"=w1813:refnum<class "Trigger.lvclass">, "Sync Box out"=w1820:refnum<class "Sync Box.lvclass">)  [unwired: 7 in]
              n704 = call-dynamic "Read State Machine.vi"("error in (no error)"=w1814, "Device in"=w1813) -> ("error out"=w1815:errorcluster, "State Machine.lvclass"=w1817:refnum<class "State Machine.lvclass">, "Device out"=w1811:refnum<class "Trigger.lvclass">)  [unwired: 7 in]
              n705 = call "Next State.vi"("error in (no error)"=w1815, "New_State"=30, "State Machine in"=w1817) -> ("error out"=w1805:errorcluster, "State Machine out"=w1806:refnum<class "State Machine.lvclass">)  [unwired: 7 in]
              n706 = call-dynamic "Write State Machine.vi"("error in (no error)"=w1805, "State Machine.lvclass"=w1806, "Device in"=w1811) -> ("error out"=w1810:errorcluster, "Device out"=w1812:refnum<class "Trigger.lvclass">)  [unwired: 7 in]
              n707 = Increment(x=w1809) -> (x+1=w1808:u32)
              n708 = call-dynamic "Write Trigger.lvclass.vi"("error in (no error)"=w1810, "Trigger.lvclass"=w1812, "Sync Box in"=w1820) -> ("error out"=w1818:errorcluster, "Sync Box out"=w1819:refnum<class "Sync Box.lvclass">)  [unwired: 7 in]
            }
          }
          n709 = call-dynamic "Write Sync Box.lvclass.vi"("error in (no error)"=w1797, "Sync Box.lvclass"=w1799, "SPARC4_AC in"=w1798) -> ("error out"=w1794:errorcluster, "SPARC4_AC out"=w1793:refnum<class "S4GUI.lvclass">)  [unwired: 7 in]
          n710 = Bundle By Name(cluster=w1793, "Obs_state"=w1791) -> (w1790:refnum<class "S4GUI.lvclass">)
        }
        frame 309 {
          # "Espera terminar a execução do comando atual \nantes de ir ao proximo passo da Observação."
          n711 = call-dynamic "Read Sync Box.lvclass.vi"("error in (no error)"=w1839, "SPARC4_AC in"=w1840) -> ("error out"=w1845:errorcluster, "Sync Box.lvclass"=w1846:refnum<class "Sync Box.lvclass">, "SPARC4_AC out"=w1842:refnum<class "S4GUI.lvclass">)  [unwired: 7 in]
          n712 = call-dynamic "Read Trigger.lvclass.vi"("error in (no error)"=w1845, "Sync Box in"=w1846) -> ("error out"=w1837:errorcluster, "Trigger.lvclass"=w1836:refnum<class "Trigger.lvclass">, "Sync Box out"=w1844:refnum<class "Sync Box.lvclass">)  [unwired: 7 in]
          n713 = call-dynamic "Read State Machine.vi"("error in (no error)"=w1837, "Device in"=w1836) -> ("error out"=w1828:errorcluster, "State Machine.lvclass"=w1830:refnum<class "State Machine.lvclass">, "Device out"=w1834:refnum<class "Trigger.lvclass">)  [unwired: 7 in]
          n714 = call-dynamic "Read State.vi"("error in (no error)"=w1828, "State Machine in"=w1830) -> ("error out"=w1827:errorcluster, "State"=w1824:i32, "State Machine out"=w1829:refnum<class "State Machine.lvclass">)  [unwired: 7 in]
          n715 = Equal To 0?(x=w1824) -> (x = 0?=w1826:bool)
          n716 = call-dynamic "Write State Machine.vi"("error in (no error)"=w1827, "State Machine.lvclass"=w1829, "Device in"=w1834) -> ("error out"=w1833:errorcluster, "Device out"=w1835:refnum<class "Trigger.lvclass">)  [unwired: 7 in]
          n717 = call-dynamic "Write Trigger.lvclass.vi"("error in (no error)"=w1833, "Trigger.lvclass"=w1835, "Sync Box in"=w1844) -> ("error out"=w1841:errorcluster, "Sync Box out"=w1843:refnum<class "Sync Box.lvclass">)  [unwired: 7 in]
          n718 = Increment(x=w1823) -> (x+1=w1822:u32)
          n719 = Select(t=w1822, s=w1826, f=w1823) -> (s? t:f=w1825:u32)
          n720 = call-dynamic "Write Sync Box.lvclass.vi"("error in (no error)"=w1841, "Sync Box.lvclass"=w1843, "SPARC4_AC in"=w1842) -> ("error out"=w1838:errorcluster, "SPARC4_AC out"=w1832:refnum<class "S4GUI.lvclass">)  [unwired: 7 in]
          n721 = Bundle By Name(cluster=w1832, "Obs_state"=w1825) -> (w1831:refnum<class "S4GUI.lvclass">)
        }
        frame 310 {
          # "Espera terminar a execução do comando atual \nantes de ir ao proximo passo da Observação."
          n722 = call-dynamic "Read AcquisitionA.vi"("error in (no error)"=w1894, "S4ACS_GUI in"=w1895) -> ("error out"=w1863:errorcluster, "Acquisition.lvclass"=w1864:refnum<class "Acquisition.lvclass">, "S4ACS_GUI out"=w1897:refnum<class "S4GUI.lvclass">)  [unwired: 7 in]
          n723 = call "Read connection.vi"("error in (no error)"=w1863, "Server in"=w1864) -> ("error out"=w1865:errorcluster, "connection"=w1867:bool, "Server out"=w1866:refnum<class "Acquisition.lvclass">)  [unwired: 7 in]
          n724 = case shown="False" w1867 {
            tunnel: [w1955 w1969] -> w1898
            tunnel: [w1954 w1968] -> w1896
            tunnel: [0 ("State") w1958] -> w1888
            tunnel: w1866 -> [w1955 w1957]
            tunnel: w1865 -> [w1954 w1956]
            frame False {
            }
            frame True {
              n725 = call-dynamic "Read Channel.vi"("error in (no error)"=w1956, "Acquisition in"=w1957) -> ("error out"=w1967:errorcluster, "Channel.lvclass"=w1966:refnum<class "Channel.lvclass">, "Acquisition out"=w1970:refnum<class "Acquisition.lvclass">)  [unwired: 7 in]
              n726 = call-dynamic "Read State Machine.vi"("error in (no error)"=w1967, "Device in"=w1966) -> ("error out"=w1960:errorcluster, "State Machine.lvclass"=w1962:refnum<class "State Machine.lvclass">, "Device out"=w1964:refnum<class "Channel.lvclass">)  [unwired: 7 in]
              n727 = call-dynamic "Read State.vi"("error in (no error)"=w1960, "State Machine in"=w1962) -> ("error out"=w1959:errorcluster, "State"=w1958:i32, "State Machine out"=w1961:refnum<class "State Machine.lvclass">)  [unwired: 7 in]
              n728 = call-dynamic "Write State Machine.vi"("error in (no error)"=w1959, "State Machine.lvclass"=w1961, "Device in"=w1964) -> ("error out"=w1963:errorcluster, "Device out"=w1965:refnum<class "Channel.lvclass">)  [unwired: 7 in]
              n729 = call-dynamic "Write Channel.vi"("error in (no error)"=w1963, "Channel.lvclass"=w1965, "Acquisition in"=w1970) -> ("error out"=w1968:errorcluster, "Acquisition out"=w1969:refnum<class "Acquisition.lvclass">)  [unwired: 7 in]
            }
          }
          n730 = call-dynamic "Write AcquisitionA.vi"("error in (no error)"=w1896, "Acquisition.lvclass"=w1898, "S4ACS_GUI in"=w1897) -> ("error out"=w1889:errorcluster, "S4ACS_GUI out"=w1890:refnum<class "S4GUI.lvclass">)  [unwired: 7 in]
          n731 = call "Read AcquisitionB.vi"("error in (no error)"=w1889, "S4ACS_GUI in"=w1890) -> ("error out"=w1860:errorcluster, "Acquisition.lvclass"=w1862:refnum<class "Acquisition.lvclass">, "S4ACS_GUI out"=w1883:refnum<class "S4GUI.lvclass">)  [unwired: 7 in]
          n732 = call "Read connection.vi"("error in (no error)"=w1860, "Server in"=w1862) -> ("error out"=w1859:errorcluster, "connection"=w1858:bool, "Server out"=w1861:refnum<class "Acquisition.lvclass">)  [unwired: 7 in]
          n733 = case shown="False" w1858 {
            tunnel: w1861 -> [w1937 w1952]
            tunnel: w1859 -> [w1936 w1951]
            tunnel: [w1937 w1949] -> w1884
            tunnel: [w1936 w1948] -> w1882
            tunnel: [0 ("State") w1938] -> w1881
            frame False {
            }
            frame True {
              n734 = call-dynamic "Read Channel.vi"("error in (no error)"=w1951, "Acquisition in"=w1952) -> ("error out"=w1947:errorcluster, "Channel.lvclass"=w1946:refnum<class "Channel.lvclass">, "Acquisition out"=w1950:refnum<class "Acquisition.lvclass">)  [unwired: 7 in]
              n735 = call-dynamic "Read State Machine.vi"("error in (no error)"=w1947, "Device in"=w1946) -> ("error out"=w1940:errorcluster, "State Machine.lvclass"=w1942:refnum<class "State Machine.lvclass">, "Device out"=w1944:refnum<class "Channel.lvclass">)  [unwired: 7 in]
              n736 = call-dynamic "Read State.vi"("error in (no error)"=w1940, "State Machine in"=w1942) -> ("error out"=w1939:errorcluster, "State"=w1938:i32, "State Machine out"=w1941:refnum<class "State Machine.lvclass">)  [unwired: 7 in]
              n737 = call-dynamic "Write State Machine.vi"("error in (no error)"=w1939, "State Machine.lvclass"=w1941, "Device in"=w1944) -> ("error out"=w1943:errorcluster, "Device out"=w1945:refnum<class "Channel.lvclass">)  [unwired: 7 in]
              n738 = call-dynamic "Write Channel.vi"("error in (no error)"=w1943, "Channel.lvclass"=w1945, "Acquisition in"=w1950) -> ("error out"=w1948:errorcluster, "Acquisition out"=w1949:refnum<class "Acquisition.lvclass">)  [unwired: 7 in]
            }
          }
          n739 = call "Write AcquisitionB.vi"("error in (no error)"=w1882, "Acquisition.lvclass"=w1884, "S4ACS_GUI in"=w1883) -> ("error out"=w1877:errorcluster, "S4ACS_GUI out"=w1876:refnum<class "S4GUI.lvclass">)  [unwired: 7 in]
          n740 = call-dynamic "Read AcquisitionC.vi"("error in (no error)"=w1877, "S4ACS_GUI in"=w1876) -> ("error out"=w1855:errorcluster, "Acquisition.lvclass"=w1857:refnum<class "Acquisition.lvclass">, "S4ACS_GUI out"=w1879:refnum<class "S4GUI.lvclass">)  [unwired: 7 in]
          n741 = call "Read connection.vi"("error in (no error)"=w1855, "Server in"=w1857) -> ("error out"=w1854:errorcluster, "connection"=w1853:bool, "Server out"=w1856:refnum<class "Acquisition.lvclass">)  [unwired: 7 in]
          n742 = case shown="False" w1853 {
            tunnel: [w1917 w1927] -> w1880
            tunnel: [w1918 w1926] -> w1878
            tunnel: [0 ("State") w1922] -> w1875
            tunnel: w1856 -> [w1918 w1921]
            tunnel: w1854 -> [w1917 w1920]
            frame False {
            }
            frame True {
              n743 = call-dynamic "Read Channel.vi"("error in (no error)"=w1920, "Acquisition in"=w1921) -> ("error out"=w1928:errorcluster, "Channel.lvclass"=w1929:refnum<class "Channel.lvclass">, "Acquisition out"=w1925:refnum<class "Acquisition.lvclass">)  [unwired: 7 in]
              n744 = call-dynamic "Read State Machine.vi"("error in (no error)"=w1928, "Device in"=w1929) -> ("error out"=w1923:errorcluster, "State Machine.lvclass"=w1933:refnum<class "State Machine.lvclass">, "Device out"=w1931:refnum<class "Channel.lvclass">)  [unwired: 7 in]
              n745 = call-dynamic "Read State.vi"("error in (no error)"=w1923, "State Machine in"=w1933) -> ("error out"=w1924:errorcluster, "State"=w1922:i32, "State Machine out"=w1934:refnum<class "State Machine.lvclass">)  [unwired: 7 in]
              n746 = call-dynamic "Write State Machine.vi"("error in (no error)"=w1924, "State Machine.lvclass"=w1934, "Device in"=w1931) -> ("error out"=w1932:errorcluster, "Device out"=w1930:refnum<class "Channel.lvclass">)  [unwired: 7 in]
              n747 = call-dynamic "Write Channel.vi"("error in (no error)"=w1932, "Channel.lvclass"=w1930, "Acquisition in"=w1925) -> ("error out"=w1927:errorcluster, "Acquisition out"=w1926:refnum<class "Acquisition.lvclass">)  [unwired: 7 in]
            }
          }
          n748 = call-dynamic "Write AcquisitionC.vi"("error in (no error)"=w1880, "Acquisition.lvclass"=w1878, "S4ACS_GUI in"=w1879) -> ("error out"=w1852:errorcluster, "S4ACS_GUI out"=w1871:refnum<class "S4GUI.lvclass">)  [unwired: 7 in]
          n749 = call-dynamic "Read AcquisitionD.vi"("error in (no error)"=w1852, "S4ACS_GUI in"=w1871) -> ("error out"=w1848:errorcluster, "Acquisition.lvclass"=w1851:refnum<class "Acquisition.lvclass">, "S4ACS_GUI out"=w1873:refnum<class "S4GUI.lvclass">)  [unwired: 7 in]
          n750 = call "Read connection.vi"("error in (no error)"=w1848, "Server in"=w1851) -> ("error out"=w1849:errorcluster, "connection"=w1847:bool, "Server out"=w1850:refnum<class "Acquisition.lvclass">)  [unwired: 7 in]
          n751 = case shown="True" w1847 {
            tunnel: [w1901 w1915] -> w1874
            tunnel: [w1900 w1914] -> w1872
            tunnel: [0 ("State") w1904] -> w1870
            tunnel: w1850 -> [w1901 w1903]
            tunnel: w1849 -> [w1900 w1902]
            frame False {
            }
            frame True {
              n752 = call-dynamic "Read Channel.vi"("error in (no error)"=w1902, "Acquisition in"=w1903) -> ("error out"=w1913:errorcluster, "Channel.lvclass"=w1912:refnum<class "Channel.lvclass">, "Acquisition out"=w1916:refnum<class "Acquisition.lvclass">)  [unwired: 7 in]
              n753 = call-dynamic "Read State Machine.vi"("error in (no error)"=w1913, "Device in"=w1912) -> ("error out"=w1906:errorcluster, "State Machine.lvclass"=w1908:refnum<class "State Machine.lvclass">, "Device out"=w1910:refnum<class "Channel.lvclass">)  [unwired: 7 in]
              n754 = call-dynamic "Read State.vi"("error in (no error)"=w1906, "State Machine in"=w1908) -> ("error out"=w1905:errorcluster, "State"=w1904:i32, "State Machine out"=w1907:refnum<class "State Machine.lvclass">)  [unwired: 7 in]
              n755 = call-dynamic "Write State Machine.vi"("error in (no error)"=w1905, "State Machine.lvclass"=w1907, "Device in"=w1910) -> ("error out"=w1909:errorcluster, "Device out"=w1911:refnum<class "Channel.lvclass">)  [unwired: 7 in]
              n756 = call-dynamic "Write Channel.vi"("error in (no error)"=w1909, "Channel.lvclass"=w1911, "Acquisition in"=w1916) -> ("error out"=w1914:errorcluster, "Acquisition out"=w1915:refnum<class "Acquisition.lvclass">)  [unwired: 7 in]
            }
          }
          n757 = call-dynamic "Write AcquisitionD.vi"("error in (no error)"=w1872, "Acquisition.lvclass"=w1874, "S4ACS_GUI in"=w1873) -> ("error out"=w1868:errorcluster, "S4ACS_GUI out"=w1869:refnum<class "S4GUI.lvclass">)  [unwired: 7 in]
          n758 = Compound Arithmetic op=ADD(w1888, w1881, w1875, w1870) -> (w1887:i32)
          n759 = Equal To 0?(x=w1887) -> (x = 0?=w1892:bool)
          n760 = Select(t=u32 301, s=w1892, f=w1886) -> (s? t:f=w1891:u32)
          n761 = Bundle By Name(cluster=w1869, "Obs_state"=w1891) -> (w1893:refnum<class "S4GUI.lvclass">)
        }
        frame 311 {
          n762 = call-dynamic "Read ciclos.vi"("error in (no error)"=w1983, "S4ACS_GUI in"=w1984) -> ("error out"=w1972:errorcluster, "ciclos"=w1977:u32, "S4ACS_GUI out"=w1985:refnum<class "S4GUI.lvclass">)  [unwired: 7 in]
          n763 = Decrement(x=w1977) -> (x-1=w1971:u32)
          n764 = Greater Than 0?(x=w1971) -> (x > 0?=w1978:bool)
          n765 = case shown="False" w1978 {
            selector: w1978 -> [w1987 w1989]
            tunnel: w1971 -> [_ w1988]
            tunnel: [w1987 w1989] -> w1976
            tunnel: [u32 0 w1988] -> w1973
            frame False {
            }
            frame True {
            }
          }
          n766 = Select(t=u32 301, s=w1976, f=u32 0) -> (s? t:f=w1979:u32)
          n767 = call-dynamic "Write ciclos.vi"("error in (no error)"=w1972, "ciclos"=w1973, "S4ACS_GUI in"=w1985) -> ("error out"=w1982:errorcluster, "S4ACS_GUI out"=w1981:refnum<class "S4GUI.lvclass">)  [unwired: 7 in]
          n768 = Bundle By Name(cluster=w1981, "Obs_state"=w1979) -> (w1980:refnum<class "S4GUI.lvclass">)
        }
        frame 321 {
          n769 = call-dynamic "Read Sync Box.lvclass.vi"("error in (no error)"=w2000, "SPARC4_AC in"=w2001) -> ("error out"=w1995:errorcluster, "Sync Box.lvclass"=w1996:refnum<class "Sync Box.lvclass">, "SPARC4_AC out"=w2003:refnum<class "S4GUI.lvclass">)  [unwired: 7 in]
          n770 = call "Read connection.vi"("error in (no error)"=w1995, "Server in"=w1996) -> ("error out"=w1994:errorcluster, "connection"=w1993:bool, "Server out"=w1992:refnum<class "Sync Box.lvclass">)  [unwired: 7 in]
          n771 = case shown="False" w1993 {
            tunnel: [w2009 w2028] -> w2004
            tunnel: [w2008 w2027] -> w2002
            tunnel: w1994 -> [w2008 w2013]
            tunnel: w1992 -> [w2009 w2012]
            tunnel: w1991 -> [w2007 w2011]
            tunnel: [w2005 w2010] -> w1990
            frame False {
              # "SyncBox desconectado. Desvia do estado de espera para configuração do SyncBox...."
              n772 = Increment(x=w2007) -> (x+1=w2006:u32)
              n773 = Increment(x=w2006) -> (x+1=w2005:u32)
            }
            frame True {
              # "Configura os \"delays\" do syncBox"
              n774 = call-dynamic "Read Trigger.lvclass.vi"("error in (no error)"=w2013, "Sync Box in"=w2012) -> ("error out"=w2023:errorcluster, "Trigger.lvclass"=w2022:refnum<class "Trigger.lvclass">, "Sync Box out"=w2029:refnum<class "Sync Box.lvclass">)  [unwired: 7 in]
              n775 = call-dynamic "Read State Machine.vi"("error in (no error)"=w2023, "Device in"=w2022) -> ("error out"=w2024:errorcluster, "State Machine.lvclass"=w2026:refnum<class "State Machine.lvclass">, "Device out"=w2020:refnum<class "Trigger.lvclass">)  [unwired: 7 in]
              n776 = call "Next State.vi"("error in (no error)"=w2024, "New_State"=10, "State Machine in"=w2026) -> ("error out"=w2015:errorcluster, "State Machine out"=w2017:refnum<class "State Machine.lvclass">)  [unwired: 7 in]
              n777 = call-dynamic "Write Timer.vi"("error in (no error)"=w2015, "Timer"=u32 5, "State Machine in"=w2017) -> ("error out"=w2014:errorcluster, "State Machine out"=w2016:refnum<class "State Machine.lvclass">)  [unwired: 7 in]
              n778 = call-dynamic "Write State Machine.vi"("error in (no error)"=w2014, "State Machine.lvclass"=w2016, "Device in"=w2020) -> ("error out"=w2019:errorcluster, "Device out"=w2021:refnum<class "Trigger.lvclass">)  [unwired: 7 in]
              n779 = Increment(x=w2011) -> (x+1=w2010:u32)
              n780 = call-dynamic "Write Trigger.lvclass.vi"("error in (no error)"=w2019, "Trigger.lvclass"=w2021, "Sync Box in"=w2029) -> ("error out"=w2027:errorcluster, "Sync Box out"=w2028:refnum<class "Sync Box.lvclass">)  [unwired: 7 in]
            }
          }
          n781 = call-dynamic "Write Sync Box.lvclass.vi"("error in (no error)"=w2002, "Sync Box.lvclass"=w2004, "SPARC4_AC in"=w2003) -> ("error out"=w1999:errorcluster, "SPARC4_AC out"=w1998:refnum<class "S4GUI.lvclass">)  [unwired: 7 in]
          n782 = Bundle By Name(cluster=w1998, "Obs_state"=w1990) -> (w1997:refnum<class "S4GUI.lvclass">)
        }
        frame 322 {
          # "Espera terminar a execução do comando atual \nantes de ir ao proximo passo da Observação."
          n783 = call-dynamic "Read Sync Box.lvclass.vi"("error in (no error)"=w2047, "SPARC4_AC in"=w2048) -> ("error out"=w2053:errorcluster, "Sync Box.lvclass"=w2054:refnum<class "Sync Box.lvclass">, "SPARC4_AC out"=w2050:refnum<class "S4GUI.lvclass">)  [unwired: 7 in]
          n784 = call-dynamic "Read Trigger.lvclass.vi"("error in (no error)"=w2053, "Sync Box in"=w2054) -> ("error out"=w2045:errorcluster, "Trigger.lvclass"=w2044:refnum<class "Trigger.lvclass">, "Sync Box out"=w2052:refnum<class "Sync Box.lvclass">)  [unwired: 7 in]
          n785 = call-dynamic "Read State Machine.vi"("error in (no error)"=w2045, "Device in"=w2044) -> ("error out"=w2036:errorcluster, "State Machine.lvclass"=w2038:refnum<class "State Machine.lvclass">, "Device out"=w2042:refnum<class "Trigger.lvclass">)  [unwired: 7 in]
          n786 = call-dynamic "Read State.vi"("error in (no error)"=w2036, "State Machine in"=w2038) -> ("error out"=w2035:errorcluster, "State"=w2032:i32, "State Machine out"=w2037:refnum<class "State Machine.lvclass">)  [unwired: 7 in]
          n787 = Equal To 0?(x=w2032) -> (x = 0?=w2034:bool)
          n788 = call-dynamic "Write State Machine.vi"("error in (no error)"=w2035, "State Machine.lvclass"=w2037, "Device in"=w2042) -> ("error out"=w2041:errorcluster, "Device out"=w2043:refnum<class "Trigger.lvclass">)  [unwired: 7 in]
          n789 = call-dynamic "Write Trigger.lvclass.vi"("error in (no error)"=w2041, "Trigger.lvclass"=w2043, "Sync Box in"=w2052) -> ("error out"=w2049:errorcluster, "Sync Box out"=w2051:refnum<class "Sync Box.lvclass">)  [unwired: 7 in]
          n790 = Increment(x=w2031) -> (x+1=w2030:u32)
          n791 = Select(t=w2030, s=w2034, f=w2031) -> (s? t:f=w2033:u32)
          n792 = call-dynamic "Write Sync Box.lvclass.vi"("error in (no error)"=w2049, "Sync Box.lvclass"=w2051, "SPARC4_AC in"=w2050) -> ("error out"=w2046:errorcluster, "SPARC4_AC out"=w2040:refnum<class "S4GUI.lvclass">)  [unwired: 7 in]
          n793 = Bundle By Name(cluster=w2040, "Obs_state"=w2033) -> (w2039:refnum<class "S4GUI.lvclass">)
        }
        frame 323 {
          n794 = call-dynamic "Read AcquisitionA.vi"("error in (no error)"=w2057, "S4ACS_GUI in"=w2058) -> ("error out"=w2075:errorcluster, "Acquisition.lvclass"=w2078:refnum<class "Acquisition.lvclass">, "S4ACS_GUI out"=w2095:refnum<class "S4GUI.lvclass">)  [unwired: 7 in]
          n795 = call "Read connection.vi"("error in (no error)"=w2075, "Server in"=w2078) -> ("error out"=w2074:errorcluster, "connection"=w2076:bool, "Server out"=w2077:refnum<class "Acquisition.lvclass">)  [unwired: 7 in]
          n796 = case shown="False" w2076 {
            tunnel: w2077 -> [w2161 w2179]
            tunnel: w2074 -> [w2160 w2178]
            tunnel: [w2161 w2176] -> w2096
            tunnel: [w2160 w2175] -> w2094
            frame False {
            }
            frame True {
              n797 = call-dynamic "Read Channel.vi"("error in (no error)"=w2178, "Acquisition in"=w2179) -> ("error out"=w2171:errorcluster, "Channel.lvclass"=w2170:refnum<class "Channel.lvclass">, "Acquisition out"=w2177:refnum<class "Acquisition.lvclass">)  [unwired: 7 in]
              n798 = call-dynamic "Read State Machine.vi"("error in (no error)"=w2171, "Device in"=w2170) -> ("error out"=w2172:errorcluster, "State Machine.lvclass"=w2174:refnum<class "State Machine.lvclass">, "Device out"=w2168:refnum<class "Channel.lvclass">)  [unwired: 7 in]
              n799 = call "Next State.vi"("error in (no error)"=w2172, "New_State"=50, "State Machine in"=w2174) -> ("error out"=w2163:errorcluster, "State Machine out"=w2165:refnum<class "State Machine.lvclass">)  [unwired: 7 in]
              n800 = call-dynamic "Write Timer.vi"("error in (no error)"=w2163, "Timer"=u32 2, "State Machine in"=w2165) -> ("error out"=w2162:errorcluster, "State Machine out"=w2164:refnum<class "State Machine.lvclass">)  [unwired: 7 in]
              n801 = call-dynamic "Write State Machine.vi"("error in (no error)"=w2162, "State Machine.lvclass"=w2164, "Device in"=w2168) -> ("error out"=w2167:errorcluster, "Device out"=w2169:refnum<class "Channel.lvclass">)  [unwired: 7 in]
              n802 = call-dynamic "Write Channel.vi"("error in (no error)"=w2167, "Channel.lvclass"=w2169, "Acquisition in"=w2177) -> ("error out"=w2175:errorcluster, "Acquisition out"=w2176:refnum<class "Acquisition.lvclass">)  [unwired: 7 in]
            }
          }
          n803 = call-dynamic "Write AcquisitionA.vi"("error in (no error)"=w2094, "Acquisition.lvclass"=w2096, "S4ACS_GUI in"=w2095) -> ("error out"=w2092:errorcluster, "S4ACS_GUI out"=w2093:refnum<class "S4GUI.lvclass">)  [unwired: 7 in]
          n804 = call "Read AcquisitionB.vi"("error in (no error)"=w2092, "S4ACS_GUI in"=w2093) -> ("error out"=w2071:errorcluster, "Acquisition.lvclass"=w2073:refnum<class "Acquisition.lvclass">, "S4ACS_GUI out"=w2090:refnum<class "S4GUI.lvclass">)  [unwired: 7 in]
          n805 = call "Read connection.vi"("error in (no error)"=w2071, "Server in"=w2073) -> ("error out"=w2070:errorcluster, "connection"=w2069:bool, "Server out"=w2072:refnum<class "Acquisition.lvclass">)  [unwired: 7 in]
          n806 = case shown="False" w2069 {
            tunnel: w2072 -> [w2141 w2159]
            tunnel: w2070 -> [w2140 w2158]
            tunnel: [w2141 w2156] -> w2091
            tunnel: [w2140 w2155] -> w2089
            frame False {
            }
            frame True {
              n807 = call-dynamic "Read Channel.vi"("error in (no error)"=w2158, "Acquisition in"=w2159) -> ("error out"=w2151:errorcluster, "Channel.lvclass"=w2150:refnum<class "Channel.lvclass">, "Acquisition out"=w2157:refnum<class "Acquisition.lvclass">)  [unwired: 7 in]
              n808 = call-dynamic "Read State Machine.vi"("error in (no error)"=w2151, "Device in"=w2150) -> ("error out"=w2152:errorcluster, "State Machine.lvclass"=w2154:refnum<class "State Machine.lvclass">, "Device out"=w2148:refnum<class "Channel.lvclass">)  [unwired: 7 in]
              n809 = call "Next State.vi"("error in (no error)"=w2152, "New_State"=50, "State Machine in"=w2154) -> ("error out"=w2143:errorcluster, "State Machine out"=w2145:refnum<class "State Machine.lvclass">)  [unwired: 7 in]
              n810 = call-dynamic "Write Timer.vi"("error in (no error)"=w2143, "Timer"=u32 2, "State Machine in"=w2145) -> ("error out"=w2142:errorcluster, "State Machine out"=w2144:refnum<class "State Machine.lvclass">)  [unwired: 7 in]
              n811 = call-dynamic "Write State Machine.vi"("error in (no error)"=w2142, "State Machine.lvclass"=w2144, "Device in"=w2148) -> ("error out"=w2147:errorcluster, "Device out"=w2149:refnum<class "Channel.lvclass">)  [unwired: 7 in]
              n812 = call-dynamic "Write Channel.vi"("error in (no error)"=w2147, "Channel.lvclass"=w2149, "Acquisition in"=w2157) -> ("error out"=w2155:errorcluster, "Acquisition out"=w2156:refnum<class "Acquisition.lvclass">)  [unwired: 7 in]
            }
          }
          n813 = call "Write AcquisitionB.vi"("error in (no error)"=w2089, "Acquisition.lvclass"=w2091, "S4ACS_GUI in"=w2090) -> ("error out"=w2085:errorcluster, "S4ACS_GUI out"=w2084:refnum<class "S4GUI.lvclass">)  [unwired: 7 in]
          n814 = call-dynamic "Read AcquisitionC.vi"("error in (no error)"=w2085, "S4ACS_GUI in"=w2084) -> ("error out"=w2066:errorcluster, "Acquisition.lvclass"=w2068:refnum<class "Acquisition.lvclass">, "S4ACS_GUI out"=w2087:refnum<class "S4GUI.lvclass">)  [unwired: 7 in]
          n815 = call "Read connection.vi"("error in (no error)"=w2066, "Server in"=w2068) -> ("error out"=w2065:errorcluster, "connection"=w2064:bool, "Server out"=w2067:refnum<class "Acquisition.lvclass">)  [unwired: 7 in]
          n816 = case shown="False" w2064 {
            tunnel: [w2120 w2126] -> w2088
            tunnel: [w2121 w2125] -> w2086
            tunnel: w2067 -> [w2121 w2123]
            tunnel: w2065 -> [w2120 w2122]
            frame False {
            }
            frame True {
              n817 = call-dynamic "Read Channel.vi"("error in (no error)"=w2122, "Acquisition in"=w2123) -> ("error out"=w2130:errorcluster, "Channel.lvclass"=w2131:refnum<class "Channel.lvclass">, "Acquisition out"=w2124:refnum<class "Acquisition.lvclass">)  [unwired: 7 in]
              n818 = call-dynamic "Read State Machine.vi"("error in (no error)"=w2130, "Device in"=w2131) -> ("error out"=w2129:errorcluster, "State Machine.lvclass"=w2127:refnum<class "State Machine.lvclass">, "Device out"=w2133:refnum<class "Channel.lvclass">)  [unwired: 7 in]
              n819 = call "Next State.vi"("error in (no error)"=w2129, "New_State"=50, "State Machine in"=w2127) -> ("error out"=w2138:errorcluster, "State Machine out"=w2136:refnum<class "State Machine.lvclass">)  [unwired: 7 in]
              n820 = call-dynamic "Write Timer.vi"("error in (no error)"=w2138, "Timer"=u32 2, "State Machine in"=w2136) -> ("error out"=w2139:errorcluster, "State Machine out"=w2137:refnum<class "State Machine.lvclass">)  [unwired: 7 in]
              n821 = call-dynamic "Write State Machine.vi"("error in (no error)"=w2139, "State Machine.lvclass"=w2137, "Device in"=w2133) -> ("error out"=w2134:errorcluster, "Device out"=w2132:refnum<class "Channel.lvclass">)  [unwired: 7 in]
              n822 = call-dynamic "Write Channel.vi"("error in (no error)"=w2134, "Channel.lvclass"=w2132, "Acquisition in"=w2124) -> ("error out"=w2126:errorcluster, "Acquisition out"=w2125:refnum<class "Acquisition.lvclass">)  [unwired: 7 in]
            }
          }
          n823 = call-dynamic "Write AcquisitionC.vi"("error in (no error)"=w2088, "Acquisition.lvclass"=w2086, "S4ACS_GUI in"=w2087) -> ("error out"=w2082:errorcluster, "S4ACS_GUI out"=w2081:refnum<class "S4GUI.lvclass">)  [unwired: 7 in]
          n824 = call-dynamic "Read AcquisitionD.vi"("error in (no error)"=w2082, "S4ACS_GUI in"=w2081) -> ("error out"=w2061:errorcluster, "Acquisition.lvclass"=w2063:refnum<class "Acquisition.lvclass">, "S4ACS_GUI out"=w2080:refnum<class "S4GUI.lvclass">)  [unwired: 7 in]
          n825 = call "Read connection.vi"("error in (no error)"=w2061, "Server in"=w2063) -> ("error out"=w2060:errorcluster, "connection"=w2059:bool, "Server out"=w2062:refnum<class "Acquisition.lvclass">)  [unwired: 7 in]
          n826 = case shown="True" w2059 {
            tunnel: w2060 -> [w2100 w2119]
            tunnel: [w2100 w2118] -> w2083
            tunnel: w2062 -> [w2101 w2104]
            tunnel: [w2101 w2102] -> w2079
            frame False {
            }
            frame True {
              n827 = call-dynamic "Read Channel.vi"("error in (no error)"=w2119, "Acquisition in"=w2104) -> ("error out"=w2114:errorcluster, "Channel.lvclass"=w2113:refnum<class "Channel.lvclass">, "Acquisition out"=w2103:refnum<class "Acquisition.lvclass">)  [unwired: 7 in]
              n828 = call-dynamic "Read State Machine.vi"("error in (no error)"=w2114, "Device in"=w2113) -> ("error out"=w2115:errorcluster, "State Machine.lvclass"=w2117:refnum<class "State Machine.lvclass">, "Device out"=w2111:refnum<class "Channel.lvclass">)  [unwired: 7 in]
              n829 = call "Next State.vi"("error in (no error)"=w2115, "New_State"=50, "State Machine in"=w2117) -> ("error out"=w2106:errorcluster, "State Machine out"=w2108:refnum<class "State Machine.lvclass">)  [unwired: 7 in]
              n830 = call-dynamic "Write Timer.vi"("error in (no error)"=w2106, "Timer"=u32 2, "State Machine in"=w2108) -> ("error out"=w2105:errorcluster, "State Machine out"=w2107:refnum<class "State Machine.lvclass">)  [unwired: 7 in]
              n831 = call-dynamic "Write State Machine.vi"("error in (no error)"=w2105, "State Machine.lvclass"=w2107, "Device in"=w2111) -> ("error out"=w2110:errorcluster, "Device out"=w2112:refnum<class "Channel.lvclass">)  [unwired: 7 in]
              n832 = call-dynamic "Write Channel.vi"("error in (no error)"=w2110, "Channel.lvclass"=w2112, "Acquisition in"=w2103) -> ("error out"=w2118:errorcluster, "Acquisition out"=w2102:refnum<class "Acquisition.lvclass">)  [unwired: 7 in]
            }
          }
          n833 = call-dynamic "Write AcquisitionD.vi"("error in (no error)"=w2083, "Acquisition.lvclass"=w2079, "S4ACS_GUI in"=w2080) -> ("error out"=w2055:errorcluster, "S4ACS_GUI out"=w2056:refnum<class "S4GUI.lvclass">)  [unwired: 7 in]
          n834 = Increment(x=w2099) -> (x+1=w2098:u32)
          n835 = Bundle By Name(cluster=w2056, "Obs_state"=w2098) -> (w2097:refnum<class "S4GUI.lvclass">)
        }
        frame 324 {
          # "Espera terminar a execução do comando atual \nantes de ir ao proximo passo da Observação."
          n836 = call-dynamic "Read AcquisitionA.vi"("error in (no error)"=w2226, "S4ACS_GUI in"=w2227) -> ("error out"=w2203:errorcluster, "Acquisition.lvclass"=w2204:refnum<class "Acquisition.lvclass">, "S4ACS_GUI out"=w2229:refnum<class "S4GUI.lvclass">)  [unwired: 7 in]
          n837 = call "Read connection.vi"("error in (no error)"=w2203, "Server in"=w2204) -> ("error out"=w2202:errorcluster, "connection"=w2201:bool, "Server out"=w2200:refnum<class "Acquisition.lvclass">)  [unwired: 7 in]
          n838 = case shown="True" w2201 {
            tunnel: w2202 -> [w2292 w2310]
            tunnel: [w2293 w2308] -> w2230
            tunnel: [w2292 w2307] -> w2228
            tunnel: [TRUE w2294] -> w2182
            tunnel: w2200 -> [w2293 w2297]
            frame False {
            }
            frame True {
              n839 = call-dynamic "Read Channel.vi"("error in (no error)"=w2310, "Acquisition in"=w2297) -> ("error out"=w2306:errorcluster, "Channel.lvclass"=w2305:refnum<class "Channel.lvclass">, "Acquisition out"=w2309:refnum<class "Acquisition.lvclass">)  [unwired: 7 in]
              n840 = call-dynamic "Read State Machine.vi"("error in (no error)"=w2306, "Device in"=w2305) -> ("error out"=w2299:errorcluster, "State Machine.lvclass"=w2301:refnum<class "State Machine.lvclass">, "Device out"=w2303:refnum<class "Channel.lvclass">)  [unwired: 7 in]
              n841 = call-dynamic "Read State.vi"("error in (no error)"=w2299, "State Machine in"=w2301) -> ("error out"=w2298:errorcluster, "State"=w2295:i32, "State Machine out"=w2300:refnum<class "State Machine.lvclass">)  [unwired: 7 in]
              n842 = Greater?(x=w2295, y=53 ("x")) -> (0:w2294:bool)
              n843 = call-dynamic "Write State Machine.vi"("error in (no error)"=w2298, "State Machine.lvclass"=w2300, "Device in"=w2303) -> ("error out"=w2302:errorcluster, "Device out"=w2304:refnum<class "Channel.lvclass">)  [unwired: 7 in]
              n844 = call-dynamic "Write Channel.vi"("error in (no error)"=w2302, "Channel.lvclass"=w2304, "Acquisition in"=w2309) -> ("error out"=w2307:errorcluster, "Acquisition out"=w2308:refnum<class "Acquisition.lvclass">)  [unwired: 7 in]
            }
          }
          n845 = call-dynamic "Write AcquisitionA.vi"("error in (no error)"=w2228, "Acquisition.lvclass"=w2230, "S4ACS_GUI in"=w2229) -> ("error out"=w2220:errorcluster, "S4ACS_GUI out"=w2219:refnum<class "S4GUI.lvclass">)  [unwired: 7 in]
          n846 = call "Read AcquisitionB.vi"("error in (no error)"=w2220, "S4ACS_GUI in"=w2219) -> ("error out"=w2195:errorcluster, "Acquisition.lvclass"=w2199:refnum<class "Acquisition.lvclass">, "S4ACS_GUI out"=w2221:refnum<class "S4GUI.lvclass">)  [unwired: 7 in]
          n847 = call "Read connection.vi"("error in (no error)"=w2195, "Server in"=w2199) -> ("error out"=w2196:errorcluster, "connection"=w2197:bool, "Server out"=w2198:refnum<class "Acquisition.lvclass">)  [unwired: 7 in]
          n848 = case shown="True" w2197 {
            tunnel: w2196 -> [w2272 w2280]
            tunnel: w2198 -> [w2273 w2279]
            tunnel: [TRUE w2274] -> w2184
            tunnel: [w2272 w2278] -> w2218
            tunnel: [w2273 w2277] -> w2217
            frame False {
            }
            frame True {
              n849 = call-dynamic "Read Channel.vi"("error in (no error)"=w2280, "Acquisition in"=w2279) -> ("error out"=w2282:errorcluster, "Channel.lvclass"=w2283:refnum<class "Channel.lvclass">, "Acquisition out"=w2281:refnum<class "Acquisition.lvclass">)  [unwired: 7 in]
              n850 = call-dynamic "Read State Machine.vi"("error in (no error)"=w2282, "Device in"=w2283) -> ("error out"=w2289:errorcluster, "State Machine.lvclass"=w2287:refnum<class "State Machine.lvclass">, "Device out"=w2285:refnum<class "Channel.lvclass">)  [unwired: 7 in]
              n851 = call-dynamic "Read State.vi"("error in (no error)"=w2289, "State Machine in"=w2287) -> ("error out"=w2290:errorcluster, "State"=w2276:i32, "State Machine out"=w2288:refnum<class "State Machine.lvclass">)  [unwired: 7 in]
              n852 = Greater?(x=w2276, y=53 ("x")) -> (0:w2274:bool)
              n853 = call-dynamic "Write State Machine.vi"("error in (no error)"=w2290, "State Machine.lvclass"=w2288, "Device in"=w2285) -> ("error out"=w2286:errorcluster, "Device out"=w2284:refnum<class "Channel.lvclass">)  [unwired: 7 in]
              n854 = call-dynamic "Write Channel.vi"("error in (no error)"=w2286, "Channel.lvclass"=w2284, "Acquisition in"=w2281) -> ("error out"=w2278:errorcluster, "Acquisition out"=w2277:refnum<class "Acquisition.lvclass">)  [unwired: 7 in]
            }
          }
          n855 = call "Write AcquisitionB.vi"("error in (no error)"=w2218, "Acquisition.lvclass"=w2217, "S4ACS_GUI in"=w2221) -> ("error out"=w2210:errorcluster, "S4ACS_GUI out"=w2209:refnum<class "S4GUI.lvclass">)  [unwired: 7 in]
          n856 = call-dynamic "Read AcquisitionC.vi"("error in (no error)"=w2210, "S4ACS_GUI in"=w2209) -> ("error out"=w2191:errorcluster, "Acquisition.lvclass"=w2194:refnum<class "Acquisition.lvclass">, "S4ACS_GUI out"=w2212:refnum<class "S4GUI.lvclass">)  [unwired: 7 in]
          n857 = call "Read connection.vi"("error in (no error)"=w2191, "Server in"=w2194) -> ("error out"=w2190:errorcluster, "connection"=w2192:bool, "Server out"=w2193:refnum<class "Acquisition.lvclass">)  [unwired: 7 in]
          n858 = case shown="True" w2192 {
            tunnel: [w2252 w2261] -> w2213
            tunnel: [w2253 w2260] -> w2211
            tunnel: w2190 -> [w2252 w2257]
            tunnel: w2193 -> [w2253 w2258]
            tunnel: [TRUE w2254] -> w2183
            frame False {
            }
            frame True {
              n859 = call-dynamic "Read Channel.vi"("error in (no error)"=w2257, "Acquisition in"=w2258) -> ("error out"=w2262:errorcluster, "Channel.lvclass"=w2263:refnum<class "Channel.lvclass">, "Acquisition out"=w2259:refnum<class "Acquisition.lvclass">)  [unwired: 7 in]
              n860 = call-dynamic "Read State Machine.vi"("error in (no error)"=w2262, "Device in"=w2263) -> ("error out"=w2269:errorcluster, "State Machine.lvclass"=w2267:refnum<class "State Machine.lvclass">, "Device out"=w2265:refnum<class "Channel.lvclass">)  [unwired: 7 in]
              n861 = call-dynamic "Read State.vi"("error in (no error)"=w2269, "State Machine in"=w2267) -> ("error out"=w2270:errorcluster, "State"=w2255:i32, "State Machine out"=w2268:refnum<class "State Machine.lvclass">)  [unwired: 7 in]
              n862 = Greater?(x=w2255, y=53 ("x")) -> (0:w2254:bool)
              n863 = call-dynamic "Write State Machine.vi"("error in (no error)"=w2270, "State Machine.lvclass"=w2268, "Device in"=w2265) -> ("error out"=w2266:errorcluster, "Device out"=w2264:refnum<class "Channel.lvclass">)  [unwired: 7 in]
              n864 = call-dynamic "Write Channel.vi"("error in (no error)"=w2266, "Channel.lvclass"=w2264, "Acquisition in"=w2259) -> ("error out"=w2261:errorcluster, "Acquisition out"=w2260:refnum<class "Acquisition.lvclass">)  [unwired: 7 in]
            }
          }
          n865 = call-dynamic "Write AcquisitionC.vi"("error in (no error)"=w2213, "Acquisition.lvclass"=w2211, "S4ACS_GUI in"=w2212) -> ("error out"=w2207:errorcluster, "S4ACS_GUI out"=w2208:refnum<class "S4GUI.lvclass">)  [unwired: 7 in]
          n866 = call-dynamic "Read AcquisitionD.vi"("error in (no error)"=w2207, "S4ACS_GUI in"=w2208) -> ("error out"=w2186:errorcluster, "Acquisition.lvclass"=w2189:refnum<class "Acquisition.lvclass">, "S4ACS_GUI out"=w2214:refnum<class "S4GUI.lvclass">)  [unwired: 7 in]
          n867 = call "Read connection.vi"("error in (no error)"=w2186, "Server in"=w2189) -> ("error out"=w2185:errorcluster, "connection"=w2187:bool, "Server out"=w2188:refnum<class "Acquisition.lvclass">)  [unwired: 7 in]
          n868 = case shown="True" w2187 {
            tunnel: [w2233 w2250] -> w2216
            tunnel: [w2232 w2249] -> w2215
            tunnel: w2188 -> [w2233 w2248]
            tunnel: w2185 -> [w2232 w2247]
            tunnel: [TRUE w2234] -> w2181
            frame False {
            }
            frame True {
              n869 = call-dynamic "Read Channel.vi"("error in (no error)"=w2247, "Acquisition in"=w2248) -> ("error out"=w2245:errorcluster, "Channel.lvclass"=w2244:refnum<class "Channel.lvclass">, "Acquisition out"=w2246:refnum<class "Acquisition.lvclass">)  [unwired: 7 in]
              n870 = call-dynamic "Read State Machine.vi"("error in (no error)"=w2245, "Device in"=w2244) -> ("error out"=w2238:errorcluster, "State Machine.lvclass"=w2240:refnum<class "State Machine.lvclass">, "Device out"=w2242:refnum<class "Channel.lvclass">)  [unwired: 7 in]
              n871 = call-dynamic "Read State.vi"("error in (no error)"=w2238, "State Machine in"=w2240) -> ("error out"=w2237:errorcluster, "State"=w2235:i32, "State Machine out"=w2239:refnum<class "State Machine.lvclass">)  [unwired: 7 in]
              n872 = Greater?(x=w2235, y=53 ("x")) -> (0:w2234:bool)
              n873 = call-dynamic "Write State Machine.vi"("error in (no error)"=w2237, "State Machine.lvclass"=w2239, "Device in"=w2242) -> ("error out"=w2241:errorcluster, "Device out"=w2243:refnum<class "Channel.lvclass">)  [unwired: 7 in]
              n874 = call-dynamic "Write Channel.vi"("error in (no error)"=w2241, "Channel.lvclass"=w2243, "Acquisition in"=w2246) -> ("error out"=w2249:errorcluster, "Acquisition out"=w2250:refnum<class "Acquisition.lvclass">)  [unwired: 7 in]
            }
          }
          n875 = call-dynamic "Write AcquisitionD.vi"("error in (no error)"=w2215, "Acquisition.lvclass"=w2216, "S4ACS_GUI in"=w2214) -> ("error out"=w2205:errorcluster, "S4ACS_GUI out"=w2206:refnum<class "S4GUI.lvclass">)  [unwired: 7 in]
          n876 = Compound Arithmetic op=AND(w2182, w2184, w2183, w2181) -> (w2180:bool)
          n877 = Increment(x=w2223) -> (x+1=w2222:u32)
          n878 = Select(t=w2222, s=w2180, f=w2223) -> (s? t:f=w2224:u32)
          n879 = Bundle By Name(cluster=w2206, "Obs_state"=w2224) -> (w2225:refnum<class "S4GUI.lvclass">)
        }
        frame 325 {
          n880 = call-dynamic "Read Sync Box.lvclass.vi"("error in (no error)"=w2321, "SPARC4_AC in"=w2322) -> ("error out"=w2314:errorcluster, "Sync Box.lvclass"=w2317:refnum<class "Sync Box.lvclass">, "SPARC4_AC out"=w2324:refnum<class "S4GUI.lvclass">)  [unwired: 7 in]
          n881 = call "Read connection.vi"("error in (no error)"=w2314, "Server in"=w2317) -> ("error out"=w2315:errorcluster, "connection"=w2313:bool, "Server out"=w2316:refnum<class "Sync Box.lvclass">)  [unwired: 7 in]
          n882 = case shown="True" w2313 {
            tunnel: w2315 -> [w2329 w2347]
            tunnel: [w2330 w2345] -> w2325
            tunnel: [w2329 w2344] -> w2323
            tunnel: w2316 -> [w2330 w2335]
            tunnel: w2312 -> [w2328 w2332]
            tunnel: [w2326 w2331] -> w2311
            frame False {
              # "SyncBox desconectado. Desvia do estado de disparo do SyncBox...."
              n883 = Increment(x=w2328) -> (x+1=w2327:u32)
              n884 = Increment(x=w2327) -> (x+1=w2326:u32)
            }
            frame True {
              # "Envia comando TRIGGER para o SyncBox"
              n885 = call-dynamic "Read Trigger.lvclass.vi"("error in (no error)"=w2347, "Sync Box in"=w2335) -> ("error out"=w2340:errorcluster, "Trigger.lvclass"=w2339:refnum<class "Trigger.lvclass">, "Sync Box out"=w2346:refnum<class "Sync Box.lvclass">)  [unwired: 7 in]
              n886 = call-dynamic "Read State Machine.vi"("error in (no error)"=w2340, "Device in"=w2339) -> ("error out"=w2341:errorcluster, "State Machine.lvclass"=w2343:refnum<class "State Machine.lvclass">, "Device out"=w2337:refnum<class "Trigger.lvclass">)  [unwired: 7 in]
              n887 = call "Next State.vi"("error in (no error)"=w2341, "New_State"=30, "State Machine in"=w2343) -> ("error out"=w2333:errorcluster, "State Machine out"=w2334:refnum<class "State Machine.lvclass">)  [unwired: 7 in]
              n888 = Increment(x=w2332) -> (x+1=w2331:u32)
              n889 = call-dynamic "Write State Machine.vi"("error in (no error)"=w2333, "State Machine.lvclass"=w2334, "Device in"=w2337) -> ("error out"=w2336:errorcluster, "Device out"=w2338:refnum<class "Trigger.lvclass">)  [unwired: 7 in]
              n890 = call-dynamic "Write Trigger.lvclass.vi"("error in (no error)"=w2336, "Trigger.lvclass"=w2338, "Sync Box in"=w2346) -> ("error out"=w2344:errorcluster, "Sync Box out"=w2345:refnum<class "Sync Box.lvclass">)  [unwired: 7 in]
            }
          }
          n891 = call-dynamic "Write Sync Box.lvclass.vi"("error in (no error)"=w2323, "Sync Box.lvclass"=w2325, "SPARC4_AC in"=w2324) -> ("error out"=w2320:errorcluster, "SPARC4_AC out"=w2319:refnum<class "S4GUI.lvclass">)  [unwired: 7 in]
          n892 = Bundle By Name(cluster=w2319, "Obs_state"=w2311) -> (w2318:refnum<class "S4GUI.lvclass">)
        }
        frame 326 {
          # "Espera terminar a execução do comando atual \nantes de ir ao proximo passo da Observação."
          n893 = call-dynamic "Read Sync Box.lvclass.vi"("error in (no error)"=w2365, "SPARC4_AC in"=w2366) -> ("error out"=w2371:errorcluster, "Sync Box.lvclass"=w2372:refnum<class "Sync Box.lvclass">, "SPARC4_AC out"=w2368:refnum<class "S4GUI.lvclass">)  [unwired: 7 in]
          n894 = call-dynamic "Read Trigger.lvclass.vi"("error in (no error)"=w2371, "Sync Box in"=w2372) -> ("error out"=w2363:errorcluster, "Trigger.lvclass"=w2362:refnum<class "Trigger.lvclass">, "Sync Box out"=w2370:refnum<class "Sync Box.lvclass">)  [unwired: 7 in]
          n895 = call-dynamic "Read State Machine.vi"("error in (no error)"=w2363, "Device in"=w2362) -> ("error out"=w2354:errorcluster, "State Machine.lvclass"=w2356:refnum<class "State Machine.lvclass">, "Device out"=w2360:refnum<class "Trigger.lvclass">)  [unwired: 7 in]
          n896 = call-dynamic "Read State.vi"("error in (no error)"=w2354, "State Machine in"=w2356) -> ("error out"=w2353:errorcluster, "State"=w2350:i32, "State Machine out"=w2355:refnum<class "State Machine.lvclass">)  [unwired: 7 in]
          n897 = Equal To 0?(x=w2350) -> (x = 0?=w2352:bool)
          n898 = call-dynamic "Write State Machine.vi"("error in (no error)"=w2353, "State Machine.lvclass"=w2355, "Device in"=w2360) -> ("error out"=w2359:errorcluster, "Device out"=w2361:refnum<class "Trigger.lvclass">)  [unwired: 7 in]
          n899 = call-dynamic "Write Trigger.lvclass.vi"("error in (no error)"=w2359, "Trigger.lvclass"=w2361, "Sync Box in"=w2370) -> ("error out"=w2367:errorcluster, "Sync Box out"=w2369:refnum<class "Sync Box.lvclass">)  [unwired: 7 in]
          n900 = Increment(x=w2349) -> (x+1=w2348:u32)
          n901 = Select(t=w2348, s=w2352, f=w2349) -> (s? t:f=w2351:u32)
          n902 = call-dynamic "Write Sync Box.lvclass.vi"("error in (no error)"=w2367, "Sync Box.lvclass"=w2369, "SPARC4_AC in"=w2368) -> ("error out"=w2364:errorcluster, "SPARC4_AC out"=w2358:refnum<class "S4GUI.lvclass">)  [unwired: 7 in]
          n903 = Bundle By Name(cluster=w2358, "Obs_state"=w2351) -> (w2357:refnum<class "S4GUI.lvclass">)
        }
        frame 327 {
          # "Espera terminar a execução do comando atual \nantes de ir ao proximo passo da Observação."
          n904 = call-dynamic "Read AcquisitionA.vi"("error in (no error)"=w2420, "S4ACS_GUI in"=w2421) -> ("error out"=w2391:errorcluster, "Acquisition.lvclass"=w2392:refnum<class "Acquisition.lvclass">, "S4ACS_GUI out"=w2423:refnum<class "S4GUI.lvclass">)  [unwired: 7 in]
          n905 = call "Read connection.vi"("error in (no error)"=w2391, "Server in"=w2392) -> ("error out"=w2390:errorcluster, "connection"=w2389:bool, "Server out"=w2388:refnum<class "Acquisition.lvclass">)  [unwired: 7 in]
          n906 = case shown="True" w2389 {
            tunnel: w2390 -> [w2480 w2496]
            tunnel: [w2481 w2494] -> w2424
            tunnel: [w2480 w2493] -> w2422
            tunnel: [0 ("State") w2483] -> w2414
            tunnel: w2388 -> [w2481 w2482]
            frame False {
            }
            frame True {
              n907 = call-dynamic "Read Channel.vi"("error in (no error)"=w2496, "Acquisition in"=w2482) -> ("error out"=w2492:errorcluster, "Channel.lvclass"=w2491:refnum<class "Channel.lvclass">, "Acquisition out"=w2495:refnum<class "Acquisition.lvclass">)  [unwired: 7 in]
              n908 = call-dynamic "Read State Machine.vi"("error in (no error)"=w2492, "Device in"=w2491) -> ("error out"=w2485:errorcluster, "State Machine.lvclass"=w2487:refnum<class "State Machine.lvclass">, "Device out"=w2489:refnum<class "Channel.lvclass">)  [unwired: 7 in]
              n909 = call-dynamic "Read State.vi"("error in (no error)"=w2485, "State Machine in"=w2487) -> ("error out"=w2484:errorcluster, "State"=w2483:i32, "State Machine out"=w2486:refnum<class "State Machine.lvclass">)  [unwired: 7 in]
              n910 = call-dynamic "Write State Machine.vi"("error in (no error)"=w2484, "State Machine.lvclass"=w2486, "Device in"=w2489) -> ("error out"=w2488:errorcluster, "Device out"=w2490:refnum<class "Channel.lvclass">)  [unwired: 7 in]
              n911 = call-dynamic "Write Channel.vi"("error in (no error)"=w2488, "Channel.lvclass"=w2490, "Acquisition in"=w2495) -> ("error out"=w2493:errorcluster, "Acquisition out"=w2494:refnum<class "Acquisition.lvclass">)  [unwired: 7 in]
            }
          }
          n912 = call-dynamic "Write AcquisitionA.vi"("error in (no error)"=w2422, "Acquisition.lvclass"=w2424, "S4ACS_GUI in"=w2423) -> ("error out"=w2410:errorcluster, "S4ACS_GUI out"=w2409:refnum<class "S4GUI.lvclass">)  [unwired: 7 in]
          n913 = call "Read AcquisitionB.vi"("error in (no error)"=w2410, "S4ACS_GUI in"=w2409) -> ("error out"=w2383:errorcluster, "Acquisition.lvclass"=w2387:refnum<class "Acquisition.lvclass">, "S4ACS_GUI out"=w2415:refnum<class "S4GUI.lvclass">)  [unwired: 7 in]
          n914 = call "Read connection.vi"("error in (no error)"=w2383, "Server in"=w2387) -> ("error out"=w2384:errorcluster, "connection"=w2385:bool, "Server out"=w2386:refnum<class "Acquisition.lvclass">)  [unwired: 7 in]
          n915 = case shown="True" w2385 {
            tunnel: w2384 -> [w2462 w2468]
            tunnel: w2386 -> [w2463 w2467]
            tunnel: [0 ("State") w2466] -> w2413
            tunnel: [w2462 w2465] -> w2408
            tunnel: [w2463 w2464] -> w2407
            frame False {
            }
            frame True {
              n916 = call-dynamic "Read Channel.vi"("error in (no error)"=w2468, "Acquisition in"=w2467) -> ("error out"=w2470:errorcluster, "Channel.lvclass"=w2471:refnum<class "Channel.lvclass">, "Acquisition out"=w2469:refnum<class "Acquisition.lvclass">)  [unwired: 7 in]
              n917 = call-dynamic "Read State Machine.vi"("error in (no error)"=w2470, "Device in"=w2471) -> ("error out"=w2477:errorcluster, "State Machine.lvclass"=w2475:refnum<class "State Machine.lvclass">, "Device out"=w2473:refnum<class "Channel.lvclass">)  [unwired: 7 in]
              n918 = call-dynamic "Read State.vi"("error in (no error)"=w2477, "State Machine in"=w2475) -> ("error out"=w2478:errorcluster, "State"=w2466:i32, "State Machine out"=w2476:refnum<class "State Machine.lvclass">)  [unwired: 7 in]
              n919 = call-dynamic "Write State Machine.vi"("error in (no error)"=w2478, "State Machine.lvclass"=w2476, "Device in"=w2473) -> ("error out"=w2474:errorcluster, "Device out"=w2472:refnum<class "Channel.lvclass">)  [unwired: 7 in]
              n920 = call-dynamic "Write Channel.vi"("error in (no error)"=w2474, "Channel.lvclass"=w2472, "Acquisition in"=w2469) -> ("error out"=w2465:errorcluster, "Acquisition out"=w2464:refnum<class "Acquisition.lvclass">)  [unwired: 7 in]
            }
          }
          n921 = call "Write AcquisitionB.vi"("error in (no error)"=w2408, "Acquisition.lvclass"=w2407, "S4ACS_GUI in"=w2415) -> ("error out"=w2400:errorcluster, "S4ACS_GUI out"=w2399:refnum<class "S4GUI.lvclass">)  [unwired: 7 in]
          n922 = call-dynamic "Read AcquisitionC.vi"("error in (no error)"=w2400, "S4ACS_GUI in"=w2399) -> ("error out"=w2379:errorcluster, "Acquisition.lvclass"=w2382:refnum<class "Acquisition.lvclass">, "S4ACS_GUI out"=w2402:refnum<class "S4GUI.lvclass">)  [unwired: 7 in]
          n923 = call "Read connection.vi"("error in (no error)"=w2379, "Server in"=w2382) -> ("error out"=w2378:errorcluster, "connection"=w2380:bool, "Server out"=w2381:refnum<class "Acquisition.lvclass">)  [unwired: 7 in]
          n924 = case shown="True" w2380 {
            tunnel: [w2444 w2451] -> w2403
            tunnel: [w2445 w2450] -> w2401
            tunnel: w2378 -> [w2444 w2446]
            tunnel: w2381 -> [w2445 w2448]
            tunnel: [0 ("State") w2447] -> w2394
            frame False {
            }
            frame True {
              n925 = call-dynamic "Read Channel.vi"("error in (no error)"=w2446, "Acquisition in"=w2448) -> ("error out"=w2452:errorcluster, "Channel.lvclass"=w2453:refnum<class "Channel.lvclass">, "Acquisition out"=w2449:refnum<class "Acquisition.lvclass">)  [unwired: 7 in]
              n926 = call-dynamic "Read State Machine.vi"("error in (no error)"=w2452, "Device in"=w2453) -> ("error out"=w2459:errorcluster, "State Machine.lvclass"=w2457:refnum<class "State Machine.lvclass">, "Device out"=w2455:refnum<class "Channel.lvclass">)  [unwired: 7 in]
              n927 = call-dynamic "Read State.vi"("error in (no error)"=w2459, "State Machine in"=w2457) -> ("error out"=w2460:errorcluster, "State"=w2447:i32, "State Machine out"=w2458:refnum<class "State Machine.lvclass">)  [unwired: 7 in]
              n928 = call-dynamic "Write State Machine.vi"("error in (no error)"=w2460, "State Machine.lvclass"=w2458, "Device in"=w2455) -> ("error out"=w2456:errorcluster, "Device out"=w2454:refnum<class "Channel.lvclass">)  [unwired: 7 in]
              n929 = call-dynamic "Write Channel.vi"("error in (no error)"=w2456, "Channel.lvclass"=w2454, "Acquisition in"=w2449) -> ("error out"=w2451:errorcluster, "Acquisition out"=w2450:refnum<class "Acquisition.lvclass">)  [unwired: 7 in]
            }
          }
          n930 = call-dynamic "Write AcquisitionC.vi"("error in (no error)"=w2403, "Acquisition.lvclass"=w2401, "S4ACS_GUI in"=w2402) -> ("error out"=w2397:errorcluster, "S4ACS_GUI out"=w2398:refnum<class "S4GUI.lvclass">)  [unwired: 7 in]
          n931 = call-dynamic "Read AcquisitionD.vi"("error in (no error)"=w2397, "S4ACS_GUI in"=w2398) -> ("error out"=w2374:errorcluster, "Acquisition.lvclass"=w2377:refnum<class "Acquisition.lvclass">, "S4ACS_GUI out"=w2404:refnum<class "S4GUI.lvclass">)  [unwired: 7 in]
          n932 = call "Read connection.vi"("error in (no error)"=w2374, "Server in"=w2377) -> ("error out"=w2373:errorcluster, "connection"=w2375:bool, "Server out"=w2376:refnum<class "Acquisition.lvclass">)  [unwired: 7 in]
          n933 = case shown="True" w2375 {
            tunnel: [w2427 w2442] -> w2406
            tunnel: [w2426 w2441] -> w2405
            tunnel: w2376 -> [w2427 w2440]
            tunnel: w2373 -> [w2426 w2439]
            tunnel: [0 ("State") w2428] -> w2393
            frame False {
            }
            frame True {
              n934 = call-dynamic "Read Channel.vi"("error in (no error)"=w2439, "Acquisition in"=w2440) -> ("error out"=w2437:errorcluster, "Channel.lvclass"=w2436:refnum<class "Channel.lvclass">, "Acquisition out"=w2438:refnum<class "Acquisition.lvclass">)  [unwired: 7 in]
              n935 = call-dynamic "Read State Machine.vi"("error in (no error)"=w2437, "Device in"=w2436) -> ("error out"=w2430:errorcluster, "State Machine.lvclass"=w2432:refnum<class "State Machine.lvclass">, "Device out"=w2434:refnum<class "Channel.lvclass">)  [unwired: 7 in]
              n936 = call-dynamic "Read State.vi"("error in (no error)"=w2430, "State Machine in"=w2432) -> ("error out"=w2429:errorcluster, "State"=w2428:i32, "State Machine out"=w2431:refnum<class "State Machine.lvclass">)  [unwired: 7 in]
              n937 = call-dynamic "Write State Machine.vi"("error in (no error)"=w2429, "State Machine.lvclass"=w2431, "Device in"=w2434) -> ("error out"=w2433:errorcluster, "Device out"=w2435:refnum<class "Channel.lvclass">)  [unwired: 7 in]
              n938 = call-dynamic "Write Channel.vi"("error in (no error)"=w2433, "Channel.lvclass"=w2435, "Acquisition in"=w2438) -> ("error out"=w2441:errorcluster, "Acquisition out"=w2442:refnum<class "Acquisition.lvclass">)  [unwired: 7 in]
            }
          }
          n939 = call-dynamic "Write AcquisitionD.vi"("error in (no error)"=w2405, "Acquisition.lvclass"=w2406, "S4ACS_GUI in"=w2404) -> ("error out"=w2395:errorcluster, "S4ACS_GUI out"=w2396:refnum<class "S4GUI.lvclass">)  [unwired: 7 in]
          n940 = Compound Arithmetic op=ADD(w2414, w2413, w2394, w2393) -> (w2411:i32)
          n941 = Equal To 0?(x=w2411) -> (x = 0?=w2412:bool)
          n942 = Increment(x=w2417) -> (x+1=w2416:u32)
          n943 = Select(t=w2416, s=w2412, f=w2417) -> (s? t:f=w2418:u32)
          n944 = Bundle By Name(cluster=w2396, "Obs_state"=w2418) -> (w2419:refnum<class "S4GUI.lvclass">)
        }
        frame 328 {
          n945 = call-dynamic "Read ciclos.vi"("error in (no error)"=w2509, "S4ACS_GUI in"=w2510) -> ("error out"=w2498:errorcluster, "ciclos"=w2503:u32, "S4ACS_GUI out"=w2511:refnum<class "S4GUI.lvclass">)  [unwired: 7 in]
          n946 = Decrement(x=w2503) -> (x-1=w2497:u32)
          n947 = Greater Than 0?(x=w2497) -> (x > 0?=w2504:bool)
          n948 = case shown="True" w2504 {
            selector: w2504 -> [w2513 w2515]
            tunnel: w2497 -> [_ w2514]
            tunnel: [w2513 w2515] -> w2502
            tunnel: [u32 0 w2514] -> w2499
            frame False {
            }
            frame True {
            }
          }
          n949 = Select(t=u32 321, s=w2502, f=u32 0) -> (s? t:f=w2505:u32)
          n950 = call-dynamic "Write ciclos.vi"("error in (no error)"=w2498, "ciclos"=w2499, "S4ACS_GUI in"=w2511) -> ("error out"=w2508:errorcluster, "S4ACS_GUI out"=w2507:refnum<class "S4GUI.lvclass">)  [unwired: 7 in]
          n951 = Bundle By Name(cluster=w2507, "Obs_state"=w2505) -> (w2506:refnum<class "S4GUI.lvclass">)
        }
        frame 400 {
          # "Estado de \"Pause\": fica parado aqui até o botão START seja pressionado."
        }
      }
    }
    frame Error {
    }
  }
  "error out" <- w3
  "S4ACS_GUI out" <- w1
